vi "myRIO_BRig_RT_v0,77__PortC.vi"() -> ()   [LabVIEW 2014]
uses:
  myRIO_BRig_RT__Case_Exp_stateList.ctl
  myRIO_BRig_RT__Case_NonExp_stateList.ctl
  <vilib>/Platform/TimedLoop/XDataNode/timing_clust.ctl
  <vilib>/Platform/TimedLoop/XDataNode/nitl_modes.ctl
  <vilib>/Platform/TimedLoop/XDataNode/wakeup.ctl
  <vilib>/WebDAVClient/Advanced/SessionHandle.ctl
  <vilib>/myRIO/Common/Instrument Driver Framework/myRIO v1.0/UART/vis/myRIO v1.0 Close UART.vi
  <vilib>/FPGAPlugInAG/myRIO-1900/niLvFpga_Open_myRIO-1900.vi
  <vilib>/rvi/interface/common/dynamic/niFpgaDynamicAddResources.vi
  <vilib>/Utility/error.llb/Error Cluster From Error Code.vi
  <vilib>/rvi/errors/niLvFpgaAdjustHostInterfaceError.vi
  <vilib>/FPGAPlugInAG/Dynamic/niLvFpga_Close_Dynamic.vi
  <vilib>/myRIO/Common/Instrument Driver Framework/Utilities/vis/FPGA Ref Manager.vi
  <vilib>/myRIO/Common/Instrument Driver Framework/myRIO v1.0/myRIO v1.0 Reset FPGA.vi
  <vilib>/myRIO/Common/Instrument Driver Framework/myRIO v1.0/IRQ/vis/myRIO v1.0 IRQ Info FGV.vi
  <vilib>/myRIO/Common/Instrument Driver Framework/myRIO v1.0/IRQ/vis/myRIO v1.0 Timer IRQ Info FGV.vi
  <vilib>/myRIO/Common/Instrument Driver Framework/myRIO v1.0/IRQ/vis/myRIO v1.0 ISR Agent.vi
  <vilib>/rvi/interface/nirviOpenFPGA/nirviOpenFPGA.xnode
  FPGA Bitfiles/myRIOBRig_FPGATarget_myRIOBRigFPGAv3,_Jim92IOu6W4.lvbitx
  myRIO_BRig_FPGA_v3,70__PortC.vi
  <vilib>/rvi/interface/nirviReadWriteControl/nirviReadWriteControl.xnode
  <vilib>/Platform/TimedLoop/XDataNode/XDataNode.xnode
  <vilib>/rvi/interface/nirviCloseFPGA/nirviCloseFPGA.xnode
  <vilib>/Platform/TimedLoop/XDataNode/XDNodeRunTimeDep.lvlib
  <vilib>/rvi/interface/Simulation/niFpgaSimulationCallBeginRW.vi
  <vilib>/myRIO/Instrument Drivers/Utilities/Utilities.lvlib
  <vilib>/WebDAVClient/NI_WebDAV.lvlib
  NiFpgaLv.dll
panel:
  in  "Cue1Param_AudioLed_Count_NS":u16
  in  "Cue1Param_AudioLed_Count_Switch":u16
  in  "Cue1Param_AudioLed_Probability_NS":u16
  in  "Cue1Param_CueType_NS":u16(slide) max=2 step=1 scale=0.0..2.0
  in  "Cue1Param_AudioLed_Probability_Switch":u16
  in  "Cue1Param_CueType_Switch":u16(slide) max=2 step=1 scale=0.0..2.0
  in  "CueLed_Freq":dbl=10.0
  in  "CueLed_Tpeak":dbl=2.0
  in  "CueLed_duration":u16
  in  "Laser_power_step_l2":dbl
  in  "Laser_power_max_l2":dbl
  in  "Laser_power_min_l2":dbl
  in  "Laser_Tshutter_l2":dbl=2.0
  in  "Laser_Freq_l2":dbl=10.0
  in  "Laser_Tpeak_l2":dbl=2.0
  in  "Laser_duration_l2":u16
  in  "LC_Sel_Count_NS_l2":u16
  in  "LC_Sel_Count_Switch_l2":u16
  in  "LC_Sel_Probability_NS_l2":u16
  in  "LC_Sel_Block_NS_l2":u16(slide) max=2 step=1 scale=0.0..2.0
  in  "LC_Sel_OnOff_NS_l2":bool
  in  "LC_Sel_Probability_Switch_l2":u16
  in  "LC_Sel_Block_Switch_l2":u16(slide) max=2 step=1 scale=0.0..2.0
  in  "LC_Sel_OnOff_Switch_l2":bool
  in  "LC_Sel_Tdelay_NS_l2":u16
  in  "LC_Sel_Tdelay_Switch_l2":u16
  in  "LC_Cue1_Count_NS_l2":u16
  in  "LC_Cue1_Count_Switch_l2":u16
  in  "LC_Cue1_delayOpt_NS_l2":bool
  in  "LC_ENL1_delayOpt_NS_l2":bool
  in  "LC_ENL1_Count_NS_l2":u16
  in  "LC_ENL1_Count_Switch_l2":u16
  in  "LC_Cue1_delayOpt_Switch_l2":bool
  in  "LC_ENL1_delayOpt_Switch_l2":bool
  in  "LC_Cue1_Probability_NS_l2":u16
  in  "LC_Cue1_Block_NS_l2":u16(slide) max=2 step=1 scale=0.0..2.0
  in  "LC_Cue1_OnOff_NS_l2":bool
  in  "LC_Cue1_Probability_Switch_l2":u16
  in  "LC_Cue1_Block_Switch_l2":u16(slide) max=2 step=1 scale=0.0..2.0
  in  "LC_Cue1_OnOff_Switch_l2":bool
  in  "LC_ENL1_Probability_NS_l2":u16 max=100 step=1
  in  "LC_ENL1_Block_NS_l2":u16(slide) max=2 step=1 scale=0.0..2.0
  in  "LC_ENL1_OnOff_NS_l2":bool
  in  "LC_ENL1_Probability_Switch_l2":u16 max=100 step=1
  in  "LC_ENL1_Block_Switch_l2":u16(slide) max=2 step=1 scale=0.0..2.0
  in  "LC_Cue1_Tdelay_NS_l2":u16
  in  "LC_ENL1_Tdelay_NS_l2":u16
  in  "LC_Cue1_Tdelay_Switch_l2":u16
  in  "LC_ENL1_Tdelay_Switch_l2":u16
  in  "LC_ENL1_OnOff_Switch_l2":bool
  in  "LC_Wrong_Probability_l2":u16
  in  "LC_Wrong_Trial_l2":u16(slide) max=2 step=1 scale=0.0..2.0
  in  "LC_Wrong_Block_l2":u16(slide) max=2 step=1 scale=0.0..2.0
  in  "LC_Wrong_OnOff_l2":bool
  in  "LC_l2_Reward_Probability":u16
  in  "LC_l2_Reward_Trial":u16(slide) max=2 step=1 scale=0.0..2.0
  in  "LC_l2_Reward_Block":u16(slide) max=2 step=1 scale=0.0..2.0
  in  "LC_l2_Reward_OnOff":bool
  in  "LC_Wrong_Tdelay_l2":u16
  in  "LC_l2_Reward_Tdelay":u16
  in  "LC_Sel_Count_NS_l1":u16
  in  "LC_Sel_Count_Switch_l1":u16
  in  "LC_Sel_Probability_NS_l1":u16
  in  "LC_Sel_Block_NS_l1":u16(slide) max=2 step=1 scale=0.0..2.0
  in  "LC_Sel_OnOff_NS_l1":bool
  in  "LC_Sel_Probability_Switch_l1":u16
  in  "LC_Sel_Block_Switch_l1":u16(slide) max=2 step=1 scale=0.0..2.0
  in  "LC_Sel_OnOff_Switch_l1":bool
  in  "LC_Sel_Tdelay_NS_l1":u16
  in  "LC_Sel_Tdelay_Switch_l1":u16
  out "I_connect_TCP":bool
  out "error out 5":errorcluster
  in  "get_countPerMS":bool
  in  "count_warmup_R_reset":bool
  in  "count_warmup_L_reset":bool
  out "count_warmup_R":u16
  out "count_warmup_L":u16
  out "SolenoidReward":bool
  in  "SolenoidProbability_L":u16=50 caption="Reward Time [ms]" min=1 max=1000 step=1
  in  "SolenoidProbability_R":u16=50 caption="Reward Time [ms]" min=1 max=1000 step=1
  out "output_PortA":dbl caption="LaserPower"
  out "error out 4":errorcluster
  in  "Laser_power_step_l1":dbl
  in  "Laser_power_max_l1":dbl
  in  "Recording":bool
  out "error out 3":errorcluster
  out "error out 2":errorcluster
  in  "Laser_power_min_l1":dbl
  in  "FPGA_count2ms":dbl=159.0
  in  "Laser_Tshutter_l1":dbl=2.0
  in  "Laser_Freq_l1":dbl=10.0
  in  "Laser_Tpeak_l1":dbl=2.0
  in  "Laser_duration_l1":u16
  out "error out":errorcluster
  in  "LC_Cue1_Count_NS_l1":u16
  in  "LC_Cue1_Count_Switch_l1":u16
  in  "LC_Cue1_delayOpt_NS_l1":bool
  in  "LC_ENL1_delayOpt_NS_l1":bool
  in  "LC_ENL1_Count_NS_l1":u16
  in  "LC_ENL1_Count_Switch_l1":u16
  in  "LC_Cue1_delayOpt_Switch_l1":bool
  in  "LC_ENL1_delayOpt_Switch_l1":bool
  in  "Tcycle_Cue_max":u16=1000 caption="Max" min=5 max=5000 step=5
  in  "Tcycle_Cue_min":u16=1000 caption="Min" min=5 max=5000 step=5
  in  "SendData":bool
  out "cSpout":enum16{"Left", "Right"}(ring) caption="Left or Right Spout"
  out "A4":u32 caption="LickCounter_Right"
  out "A2":u32 caption="LickCounter_Left"
  in  "laserResponse_wrong_LED":bool
  out "error_initTrial":errorcluster
  out "error_Selection_pre":errorcluster
  out "error_Selection":errorcluster
  out "SelectWrong":bool
  out "SelectReward":bool
  in  "Left(F)_or_Right(T)":bool
  in  "ignoreWrong":bool
  in  "SelectionState":bool
  in  "laserResponse_wrong":bool
  in  "laserResponse_reward":bool
  in  "laserResponse_reward_LED":bool
  out "nRewards_Right":u16 caption="# Rewards Total (Right)"
  out "nRewards_Left":u16 caption="# Rewards Total (Left)"
  out "nRewards_cur":u16 caption="# Rewards in Current Block"
  out "TpB_target":u16 caption="Target Trials Per Block"
  out "cState_NonExp":T1 caption="WarmUp State"
  out "iBlock":u16 caption="Current Block"
  out "cState":T2 caption="Experimental State"
  out "iTrial":u16 caption="Current Trial"
  in  "warmupType":u8(slide) max=2 step=1 scale=0.0..2.0
  in  "TestConnection":bool
  in  "warmup":bool caption="WarmUp"
  in  "Data Set Prefix":string="Exp1_TM2"
  out "Connected To Host?":bool
  in  "Host Password":string="sabalab"
  in  "Host UserName":string="Test2"
  in  "sp_RightSpout":u16(slide)=2 max=2 step=1 scale=0.0..2.0
  in  "sp_LeftSpout":u16(slide)=2 max=2 step=1 scale=0.0..2.0
  in  "BUR_max":u16 caption="Count Reward Structure  (0 = off)"
  in  "LC_Wrong_Probability_l1":u16
  in  "LC_Wrong_Trial_l1":u16(slide) max=2 step=1 scale=0.0..2.0
  in  "LC_Wrong_Block_l1":u16(slide) max=2 step=1 scale=0.0..2.0
  in  "LC_Wrong_OnOff_l1":bool
  in  "LC_Reward_Probability_l1":u16
  in  "LC_Reward_Trial_l1":u16(slide) max=2 step=1 scale=0.0..2.0
  in  "LC_Reward_Block_l1":u16(slide) max=2 step=1 scale=0.0..2.0
  in  "LC_Reward_OnOff_l1":bool
  in  "LC_Cue1_Probability_NS_l1":u16
  in  "LC_Cue1_Block_NS_l1":u16(slide) max=2 step=1 scale=0.0..2.0
  in  "LC_Cue1_OnOff_NS_l1":bool
  in  "LC_Cue1_Probability_Switch_l1":u16
  in  "LC_Cue1_Block_Switch_l1":u16(slide) max=2 step=1 scale=0.0..2.0
  in  "LC_Cue1_OnOff_Switch_l1":bool
  in  "LC_ENL1_Probability_NS_l1":u16 max=100 step=1
  in  "LC_ENL1_Block_NS_l1":u16(slide) max=2 step=1 scale=0.0..2.0
  in  "LC_ENL1_OnOff_NS_l1":bool
  in  "LC_ENL1_Probability_Switch_l1":u16 max=100 step=1
  in  "LC_ENL1_Block_Switch_l1":u16(slide) max=2 step=1 scale=0.0..2.0
  in  "Tcycle_Timeout":u16=1000 caption="Timeout Time [ms]" min=10 max=10000 step=1
  in  "Tcycle_Wrong":u16=1000 caption="Wrong Time [ms]" min=10 max=10000 step=1
  in  "Tcycle_Selection":u16=1000 caption="Answer Time [ms]" min=1 max=10000 step=1
  in  "Tcycle_RewardPost":u16=1000 caption="Consumption Time [ms]" min=250 max=10000 step=250
  in  "Tcycle_Reward_L":u16=500 caption="Reward Time [ms]" min=1 max=1000 step=1
  in  "Tcycle_Reward_R":u16=500 caption="Reward Time [ms]" min=1 max=1000 step=1
  in  "TpB_Max_R":u16=4 caption="Max TrialsPerBlock" min=1 max=12 step=1
  in  "TpB_Min_R":u16=4 caption="Min TrialsPerBlock" min=1 max=12 step=1
  in  "TpB_Max_L":u16=4 caption="Max TrialsPerBlock" min=1 max=12 step=1
  in  "TpB_Min_L":u16=4 caption="Min TrialsPerBlock" min=1 max=12 step=1
  in  "BUR_min":u16 caption="Count Reward Structure\n(0 = off)"
  in  "TrialUntilReward":bool caption="Ignore Wrong Selection"
  in  "CueCycles":u16=1 caption="Cue Structure" min=1 max=1 step=1
  in  "MTrig_Laser_Tcycle":u16=10 caption="Time [ms]"
  in  "MTrig_Laser_trig":bool
  in  "MTrig_Audio_trig__R":bool caption="Trigger Audio"
  in  "MTrig_Audio_trig__L":bool caption="Trigger Audio"
  in  "RewCalib_Trig_R":bool caption="Calibrate_R"
  in  "RewCalib_Trig_L":bool caption="Calibrate_L"
  in  "MTrig_Solenoid_Tcycle__R":u16=300 caption="Time [ms]"
  in  "MTrig_Solenoid_Tcycle__L":u16=300 caption="Time [ms]"
  in  "MTrig_Solenoid_trig__R":bool caption="Solenoid"
  in  "MTrig_Solenoid_trig__L":bool caption="Solenoid"
  in  "STOP_abort":bool caption="Stop LabView\n(Stops myRio and FPGA)"
  in  "STOP_endBlock":bool caption="Stop Experiment\n@ End of Block"
  in  "STOP_endTrial":bool caption="Stop Experiment\n@ End of Trial"
  in  "START":bool caption="Start Experiment"
  in  "Tcycle_CuePenalty":u16=1000 caption="Penalty" min=1 max=10000 step=1
  in  "Audio_Amp__R":u16=100 caption="Amp"
  in  "Audio_Freq__R":u8=5 caption="Freq [kHz]" max=14 step=1
  in  "Audio_Amp__L":u16=100 caption="Amp"
  in  "Audio_Freq__L":u8=5 caption="Freq [kHz]" max=14 step=1
  in  "LC_Wrong_Tdelay_l1":u16
  in  "LC_Cue1_Tdelay_NS_l1":u16
  in  "LC_ENL1_Tdelay_NS_l1":u16
  in  "LC_Reward_Tdelay_l1":u16
  in  "LC_Cue1_Tdelay_Switch_l1":u16
  in  "LC_ENL1_Tdelay_Switch_l1":u16
  in  "LC_ENL1_OnOff_Switch_l1":bool
  in  "Tcycle_ENLPenalty":u16=100 caption="Penalty" min=10 max=10000 step=10
  in  "Tcycle_ENL_max":u16=1000 caption="Max" min=250 max=10000 step=250
  in  "Tcycle_ENL_min":u16=1000 caption="Min" min=250 max=10000 step=250
  # "Communication (Host PC)"
  # "Recording Rig"
  # "Experimental Run"
  # "Current State"
  # "STOP experiment at"
  # "Global Parameters                                                         Trial Parameters"
  # "Left/Right        Give Reward?        Laser Power [V]"
  # "FPGA Count per [ms]"
  # "Experiment Task Structure"
  # "Timing [ms]"
  # "Block                   Trial            Target Trials       # Rewards \n                                                            Per Block             Current"
  # "Min            Max            Penalty"
  # "(1) = Switching\n(2) = Two Choice"
  # "WarmUp State"
  # "Lick Counter"
  # "Enforced\nNonLick"
  # "WarmUp"
  # "Left           Right"
  # "Cue then reward (no lick)\n \nLeft                    Right"
  # "# Rewards Total\n                                                                  Left                    Right"
  # "Cue"
  # "Experimental State"
  # "Selection\n \n\n \nReward\n    Dispense\n    Time\n \n    Dispense\n    Probability\n \n\n    Consumption\n    Time\n\nWrong Choice\n \n \nTimeout Penalty"
  # "Laser1 Control\n                               On/Off      Block        Probability [%]   Delay [ms]                              Count"
  # "Left                  Right"
  # "Manual Control"
  # "Enforced\nNonLick\n      1"
  # "Min"
  # "Max"
  # "from end"
  # "Solenoid\n \nLeft              Right"
  # "Switch\nTrial"
  # "Speaker\n \nLeft                    Right"
  # "Laser"
  # "from start"
  # "Trial Per Block Structure \n               Left                        Right"
  # "from end"
  # "NonSwitch\nTrials"
  # "from start"
  # "Time\n[ms]"
  # "Time\n[ms]"
  # "Time = Cue Min"
  # "Min"
  # "Cue 1"
  # "Power = Min"
  # "from end"
  # "Switch\nTrial"
  # "Max"
  # "from start"
  # "Cue Audio Parameters"
  # "Laser1 Parameters"
  # "Left                  Right"
  # "from end"
  # "Laser1 Response\n                               On/Off      Block       Trial       Probability [%]   Delay [ms]"
  # "Frequency\n[Hz]"
  # "NonSwitch\nTrials"
  # "Frequency\n[kHz]"
  # "from start"
  # "Timing [ms]\n Duration     Peak Width   Shutter"
  # "Selection Reward"
  # "Selection"
  # "Amp\n(0 - 32,000)"
  # "from start"
  # "Switch\nTrial"
  # "Laser Power [V]\nMin          Max              Step"
  # "Speaker\nPattern\nDuring Cue"
  # "Selection Wrong"
  # "from start"
  # "NonSwitch\nTrials"
  # "Cue LED Parameters"
  # "Laser2 Parameters"
  # "Laser2 Response\n                               On/Off      Block       Trial       Probability [%]   Delay [ms]"
  # "Laser2 Control\n                               On/Off      Block        Probability [%]   Delay [ms]                              Count"
  # "Frequency\n[Hz]"
  # "Frequency\n[Hz]"
  # "Selection Reward"
  # "Enforced\nNonLick\n      1"
  # "from end"
  # "Timing [ms]\n Duration     Peak Width"
  # "Timing [ms]\n Duration     Peak Width   Shutter"
  # "Switch\nTrial"
  # "from start"
  # "Selection Wrong"
  # "from end"
  # "Laser Power [V]\nMin          Max              Step"
  # "NonSwitch\nTrials"
  # "from start"
  # "Cue 1"
  # "from end"
  # "Switch\nTrial"
  # "from start"
  # "Cue1 Control\n                                         Cue Type                     Audio or LED       LED Probability [%]      Count"
  # "from end"
  # "NonSwitch\nTrials"
  # "Cue 1"
  # "from start"
  # "Switch\nTrial"
  # "Selection"
  # "from start"
  # "Switch\nTrial"
  # "NonSwitch\nTrials"
  # "from start"
  # "NonSwitch\nTrials"
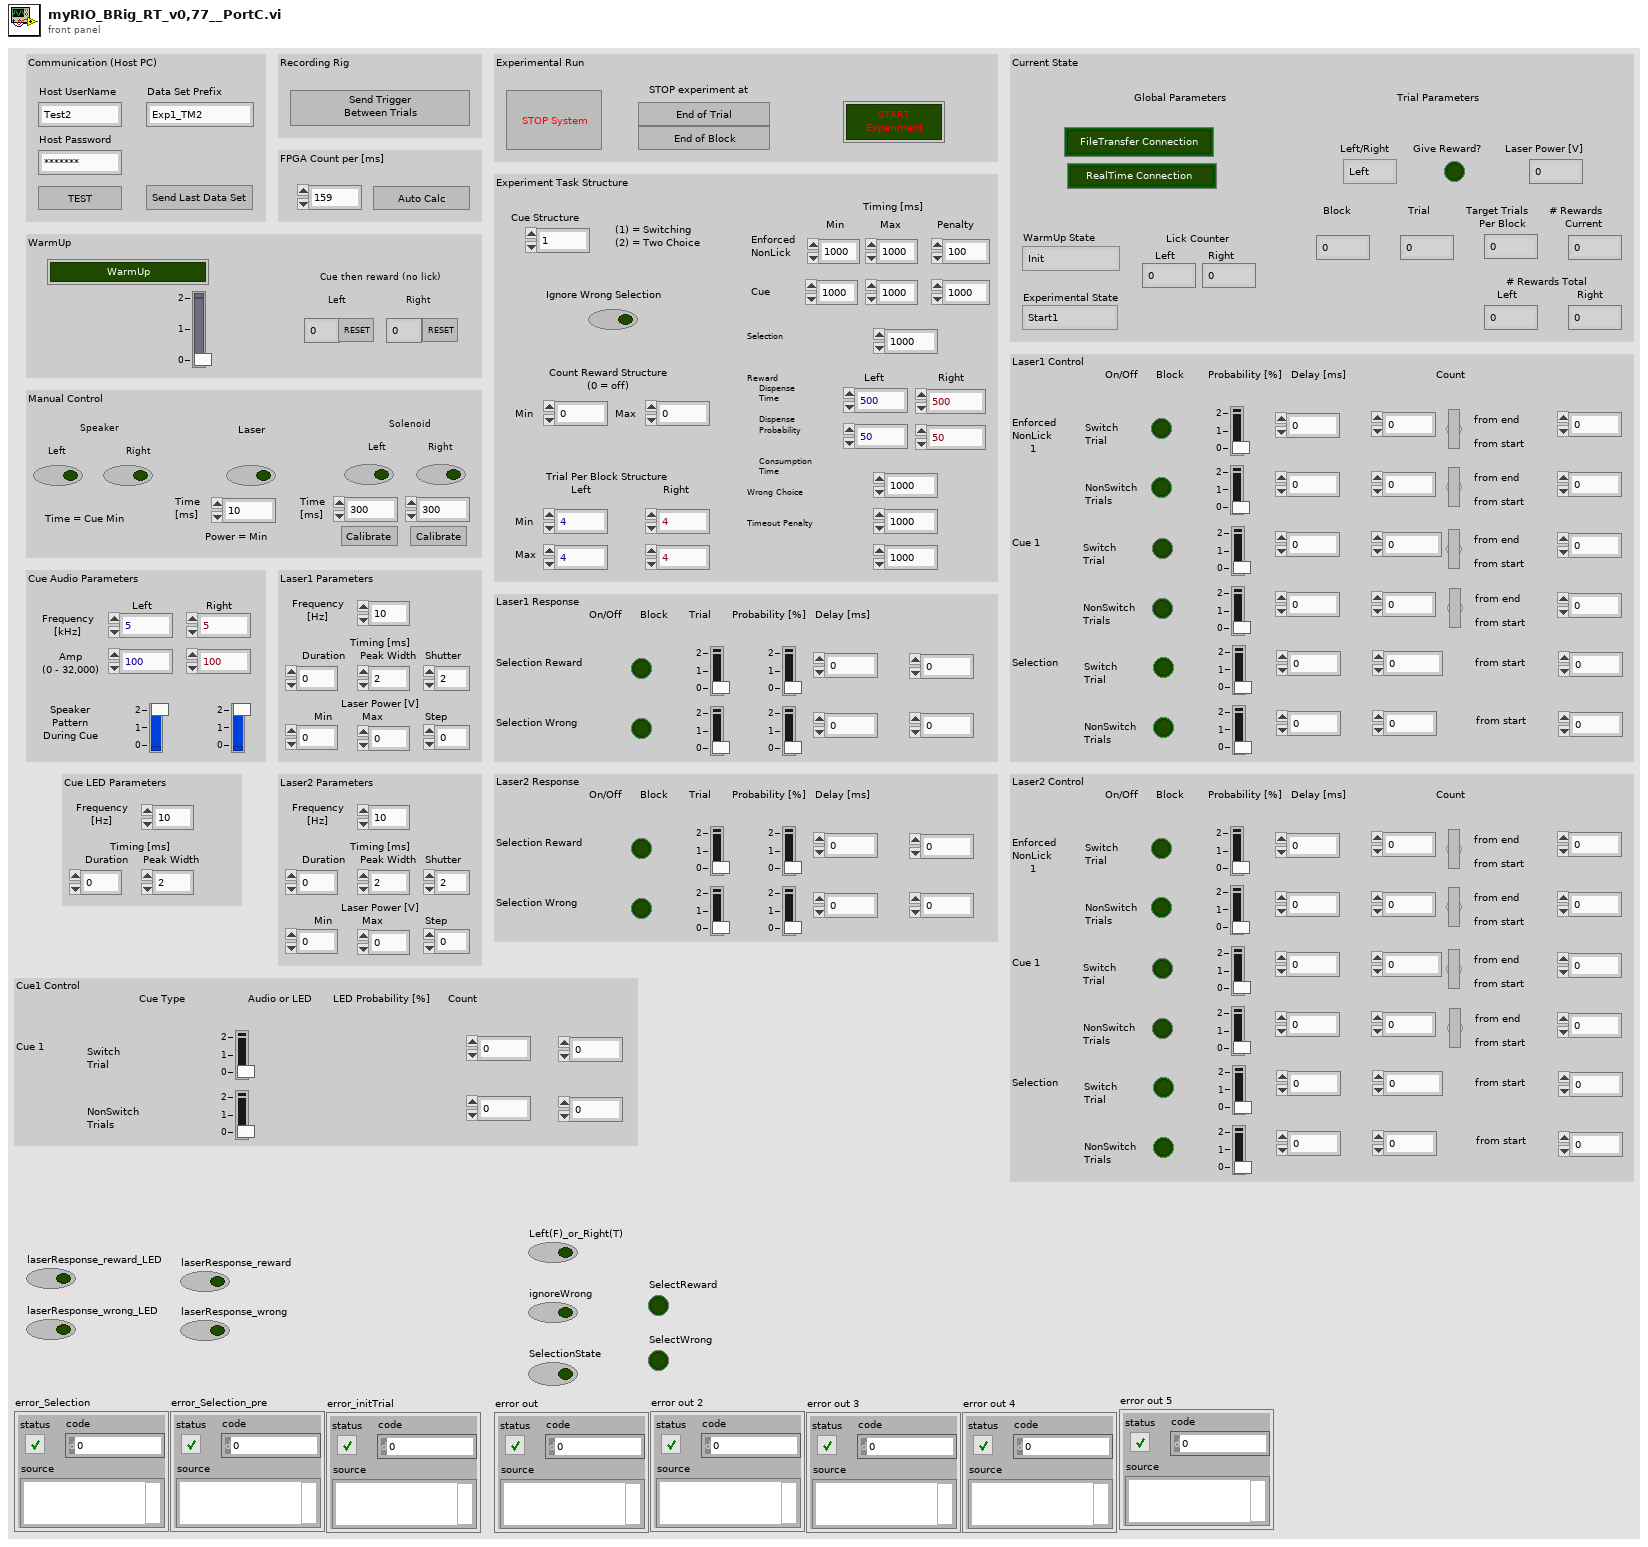
[diagram p1: front panel]
types:
  T1 = typedef "myRIO_BRig_RT__Case_NonExp_stateList.ctl" = enum16{"Init", "UploadSettings_pre", "UploadSettings_Read_dataExp", "UploadSettings_dataExp_1", "UploadSettings_dataExp_2", "UploadSettings_Read_dataLC", "UploadSettings_dataLC_1", "UploadSettings_dataLC_2", "UploadSettings_dataLC_3", "UploadSettings_dataLC_4", "UploadSettings_Read_dataMTrig", "UploadSettings_dataMTrig_1", "UploadSettings_post", "Idle_pre", "IdleEmpty", "IdleEmpty2", "IdleEmpty3", "IdleEmpty4", "Idle", "Idle_2", "Idle_3", "Idle_4", "Idle_5", "Idle_6", "Idle_post", "Cue_pre__pre", "Cue_pre", "Cue", "Cue_LED", "Cue_post", "RewardCalibration_pre", "DispenseWater_pre__pre", "DispenseWater_pre", "DispenseWater", "DispenseWater_post", "TestConnection", "SendData", "Get_FPGA_count_per_ms", "End"}
  T2 = typedef "myRIO_BRig_RT__Case_Exp_stateList.ctl" = enum16{"Start1", "Start2", "Start3", "saveSettings1", "saveSettings2", "saveSettings3", "saveSettings4", "saveSettings_LC_ENL_l1", "saveSettings_LC_ENL_l2", "saveSettings_LC_Cue_l1", "saveSettings_LC_Cue_l2", "saveSettings6_LC_l1_Other", "SaveSettings6_LC_l2_Other", "setSettings_Audio", "setSettings_Laser", "initBlock_pre", "initBlock", "initBlock2", "initBlock_post", "initTrial_pre", "initTrial", "initTrial2", "initTrial3", "initTrial4", "initTrial_LC_ENL1", "initTrial_LC_Cue1", "initTrial_LC_Cue1_2", "initTrial_LC_Sel", "initTrial_post", "ENL1_pre", "ENL1", "ENL1_post", "ENL1Penalty_pre", "ENL1Penalty", "ENL2_pre", "ENL2", "ENL2Penalty_pre", "ENL2Penalty", "Cue1_pre", "Cue1", "Cue1_post", "Cue1Penalty_pre", "Cue1Penalty", "Cue2_pre", "Cue2", "Cue2Penalty_pre", "Cue2Penalty", "Selection_pre", "Selection", "Select_post", "SelectReward_pre", "SelectReward", "SelectRewardPost_pre", "SelectRewardPost", "SelectWrong_pre", "SelectWrong", "SelectWrong_post", "SelectTimeout_pre", "SelectTimeout", "SelectTimeout_post", "endTrial_pre", "endTrial1", "endTrial2", "endTrial3", "endTrial_post", "endBlock_pre", "endBlock", "endBlock_post", "endExp", "commConnect", "commUpload_pre", "commUpload_dataBlock", "commUpload_dataCurrent", "commUpload_dataExp", "commUpload_dataLC", "commUpload_dataTrial", "commUpload_post", "saveData_pre", "saveData_dataBlock", "saveData_dataCurrent", "saveData_dataExp", "saveData_dataLC", "saveData_dataTrial", "saveData_post", "empty_endBlock1", "empty_endBlock2", "empty_endTrial1", "empty_endTrial2", "empty_endTrial3", "empty_endTrial4", "empty_endTrial5", "dummyState", "dummyState_endBlock"}
  T3 = typedef "XDNodeRunTimeDep.lvlib/timing_clust.ctl" = cluster{"Expected End [f-1]":u64, "Actual End [f-1]":u64, "Finished Late? [f-1]":bool, "Expected End [i-1]":u64, "Actual End [i-1]":u64, "Finished Late? [i-1]":bool, "Expected Start [i]":u64, "Actual Start [i]":u64, "Expected Start [f]":u64, "Actual Start [f]":u64, "Source Name":string, "Structure Name":string, "Period":i64, "Deadline":i64, "Offset":i64, "Start":i64, "Priority":i32, "Timeout":i32, "Mode":T4, "Wakeup Reason":T5, "Error":errorcluster, "Source Type":string, "Secondary Source Type":string, "Global End Time":u64, "Global Start Time":u64, "Frame Duration":u64, "Iteration Duration":u64, "Assigned CPU":i32, "I/O Scan Engine Mode":u32}
  T4 = typedef "XDNodeRunTimeDep.lvlib/nitl_modes.ctl" = enum32{"No Change", "Process missed periods, maintain original phase", "Discard missed periods, maintain original phase", "Process missed periods, ignore original phase", "Discard missed periods, ignore original phase"}
  T5 = typedef "XDNodeRunTimeDep.lvlib/wakeup.ctl" = enum32{"Normal", "Aborted", "Asynchronous wakeup", "Timing source error", "Timed loop error", "Timeout"}
  T6 = typedef "NI_WebDAV.lvlib/SessionHandle.ctl" = refnum<k1>
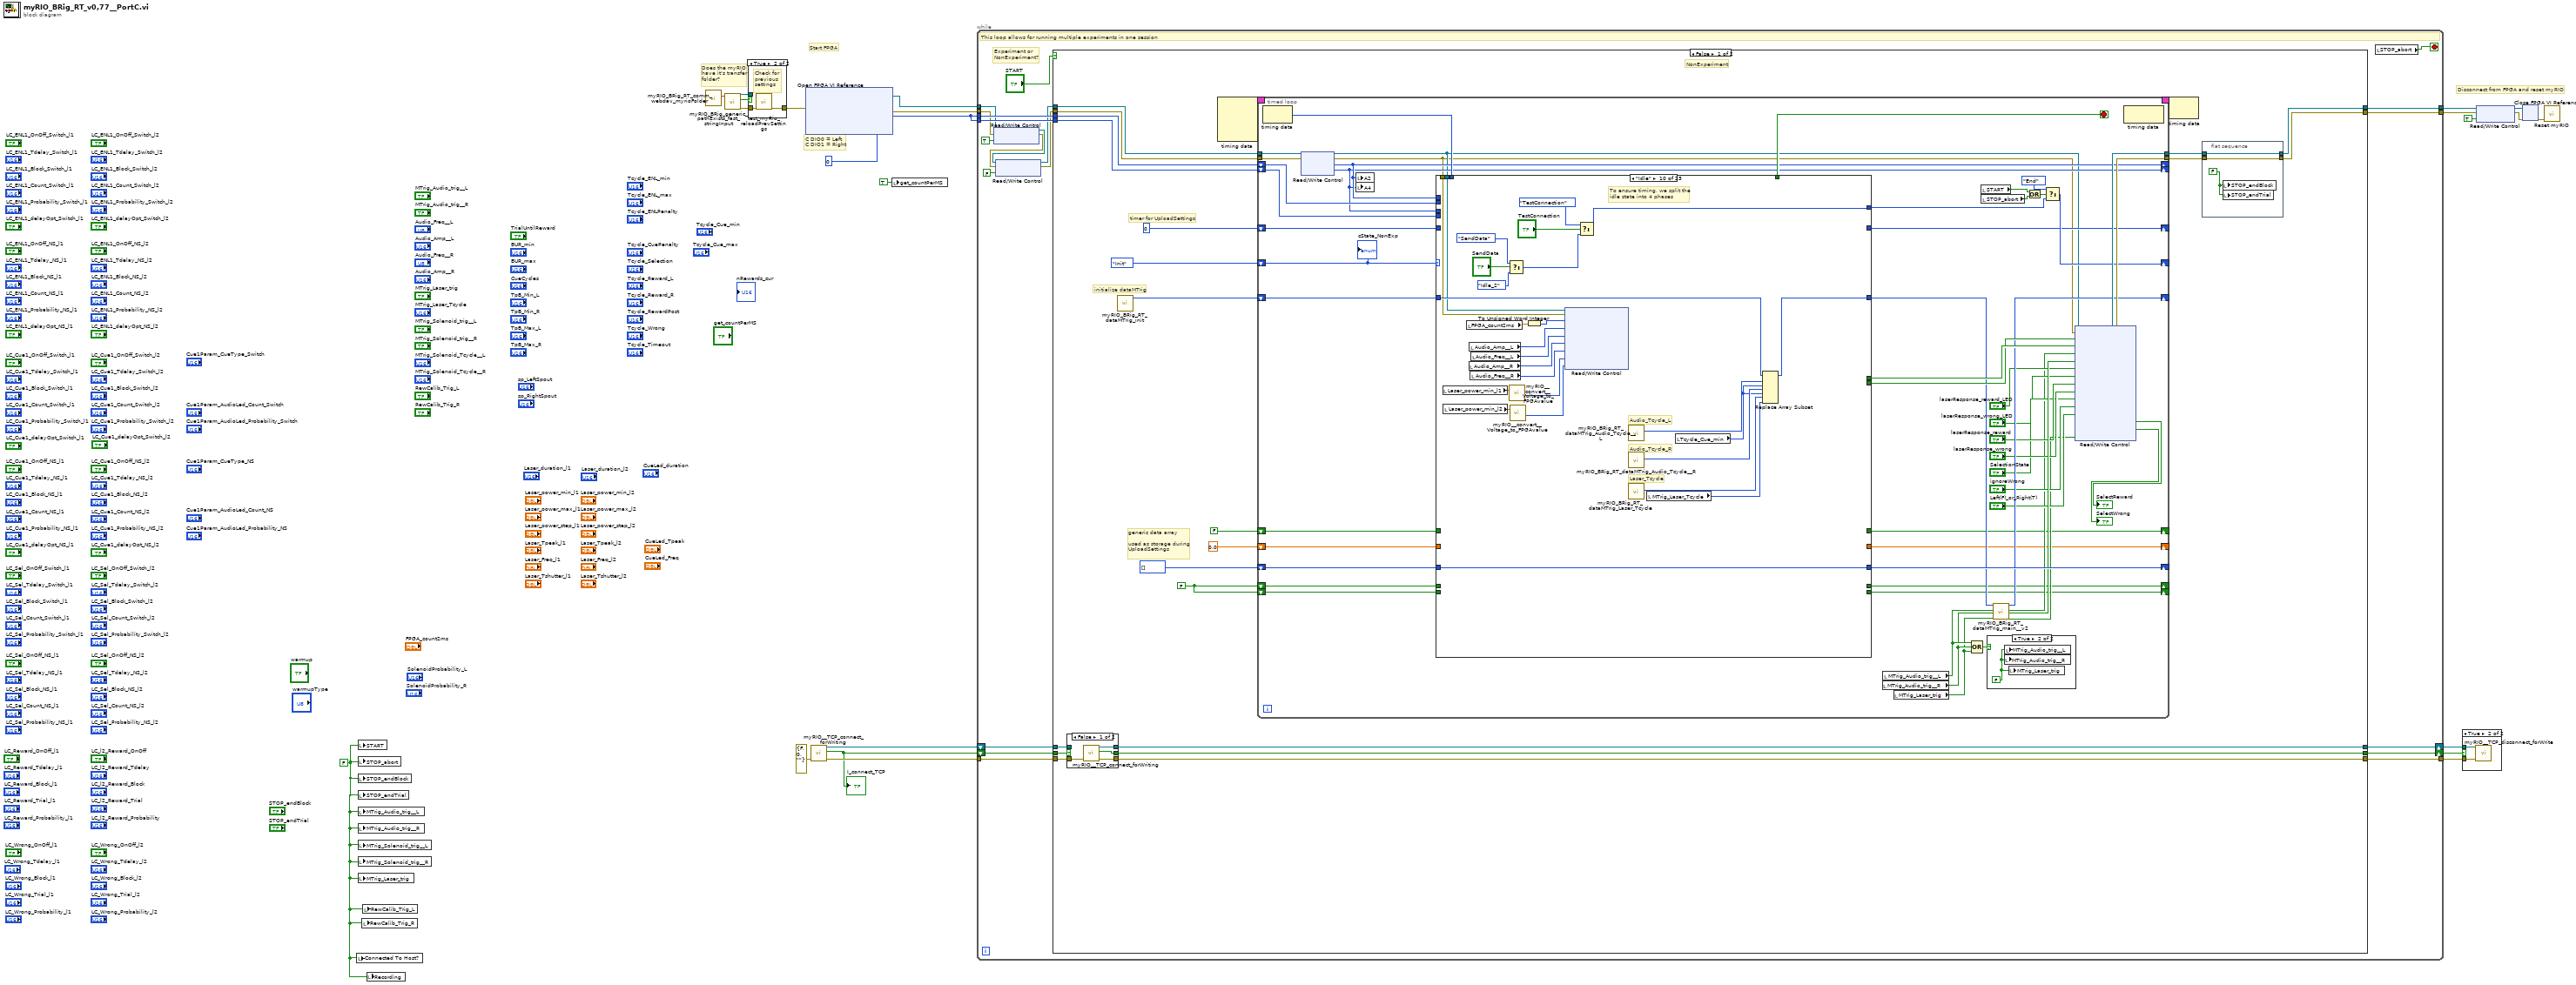
[diagram p0: block diagram]
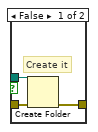
[diagram p3: hidden frame]
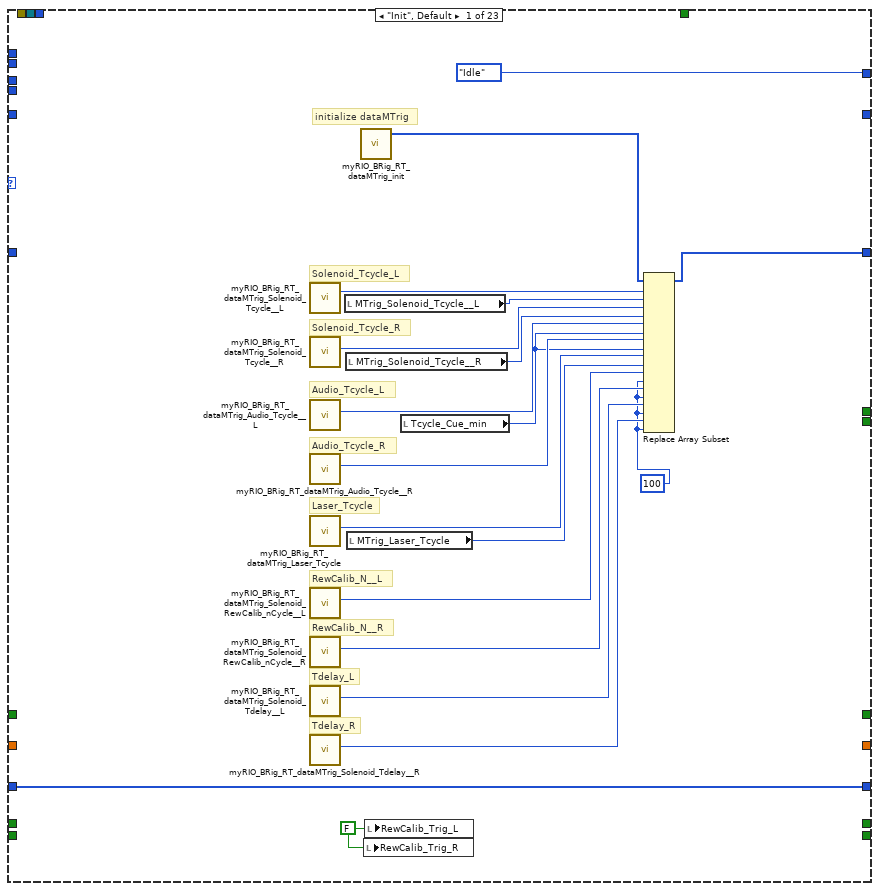
[diagram p6: hidden frame]
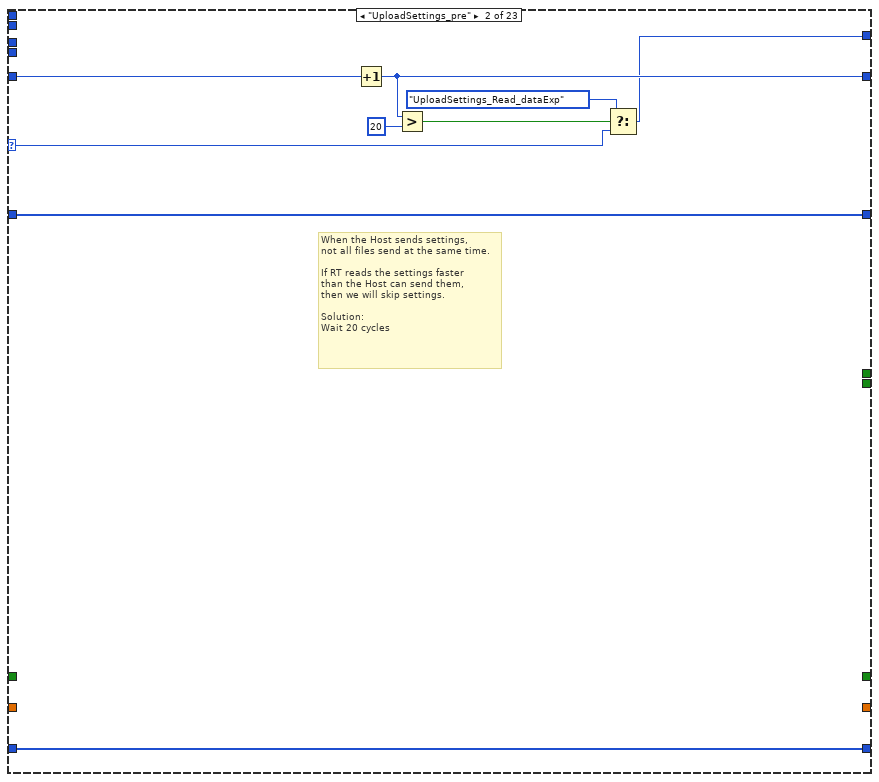
[diagram p7: hidden frame]
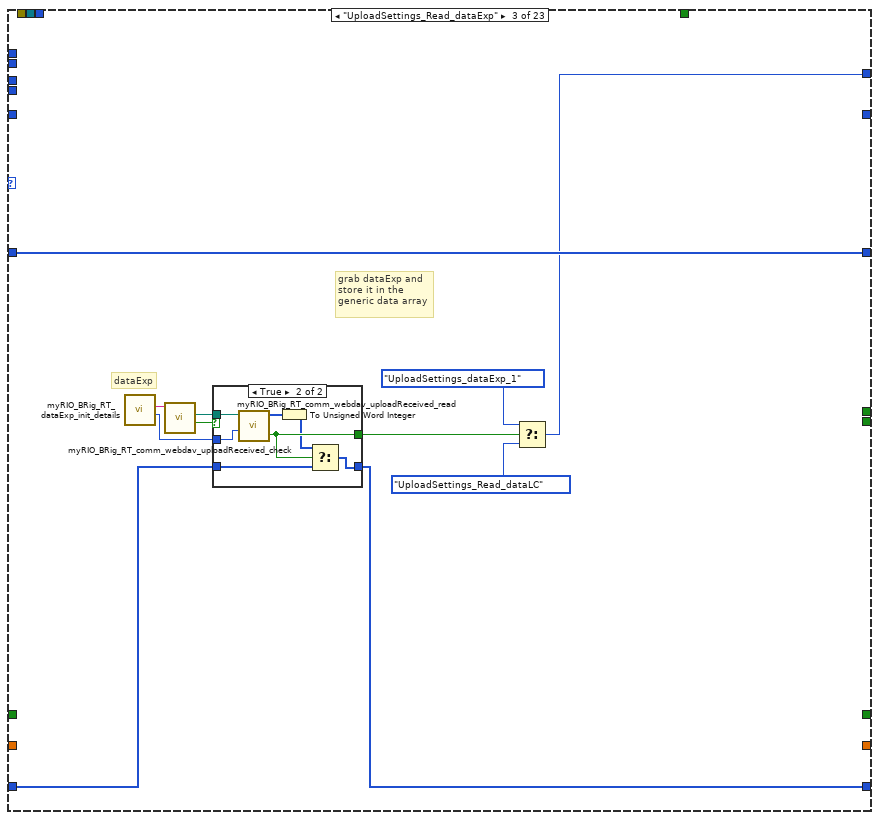
[diagram p8: hidden frame]
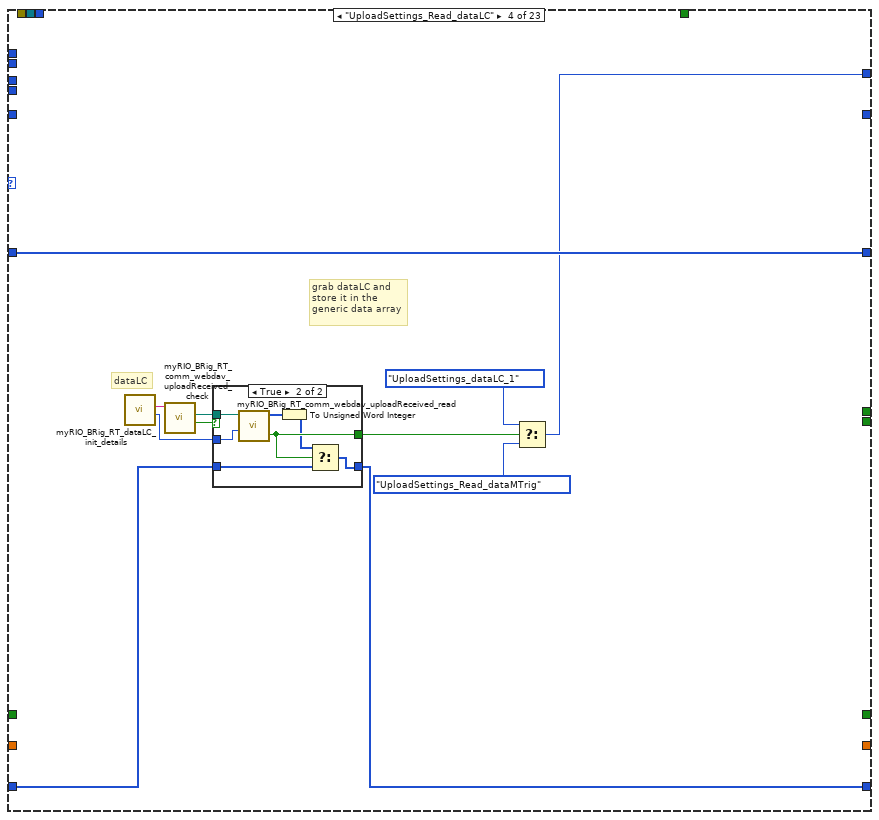
[diagram p10: hidden frame]
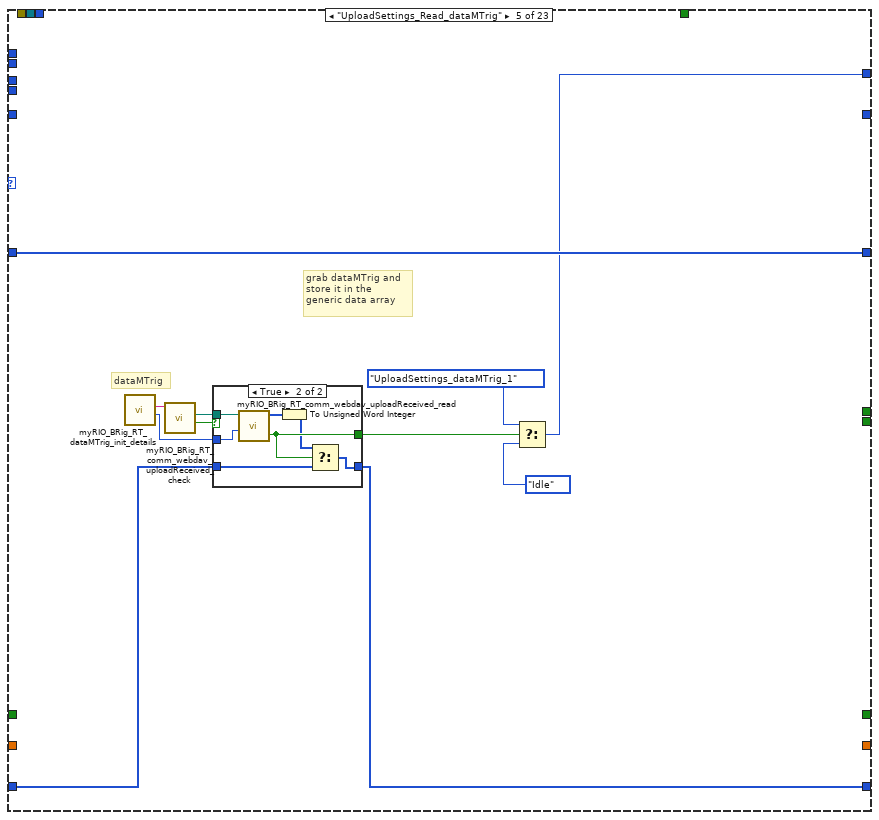
[diagram p12: hidden frame]
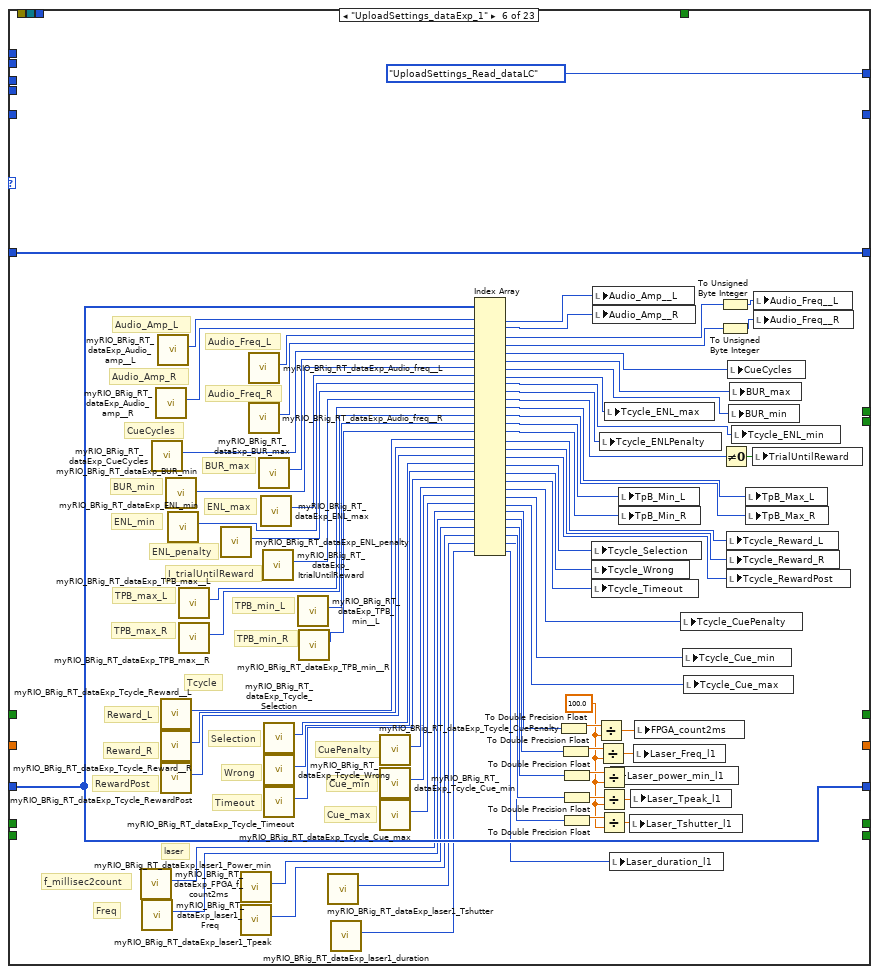
[diagram p14: hidden frame]
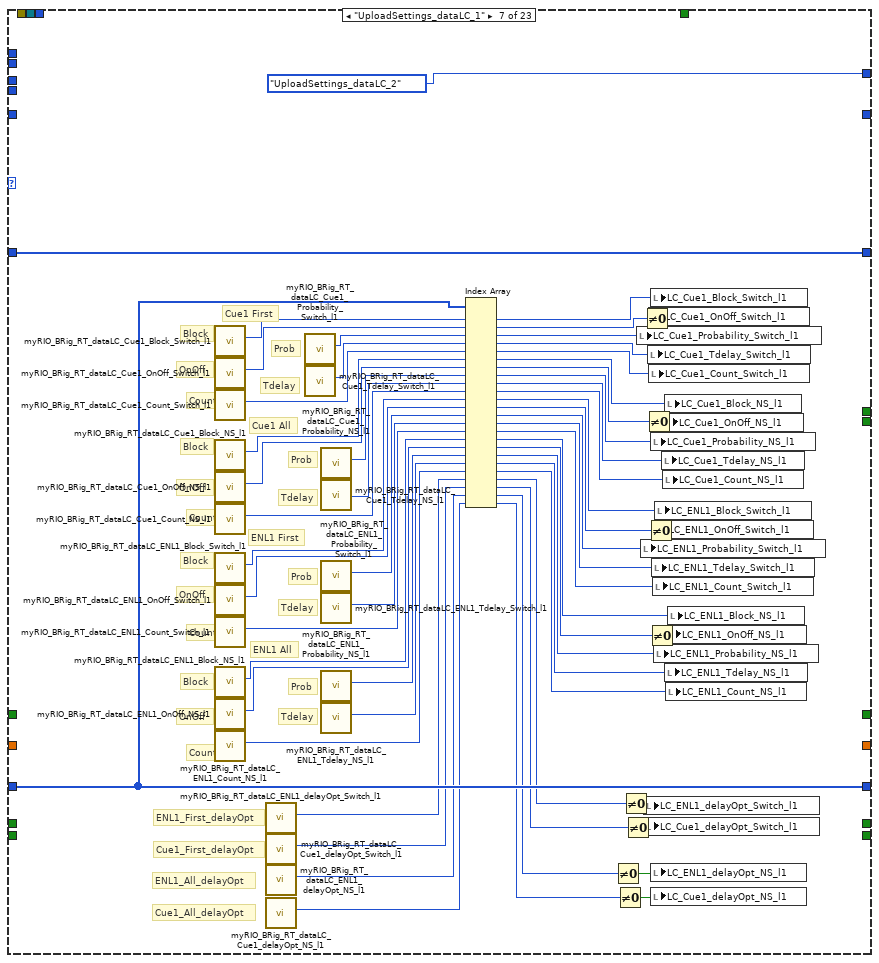
[diagram p15: hidden frame]
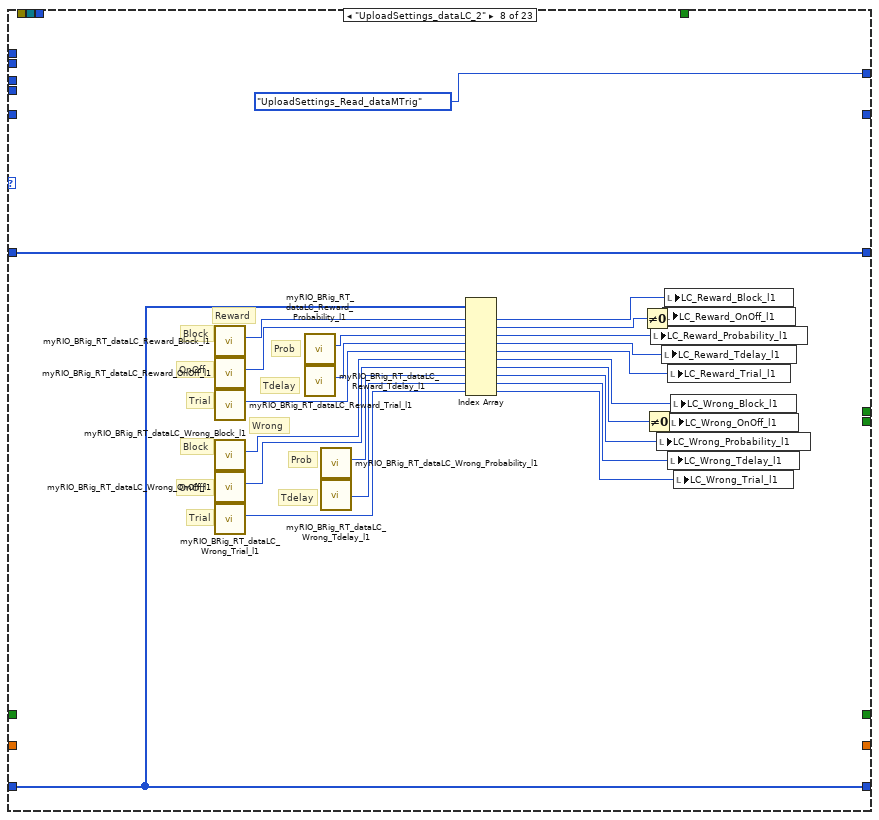
[diagram p16: hidden frame]
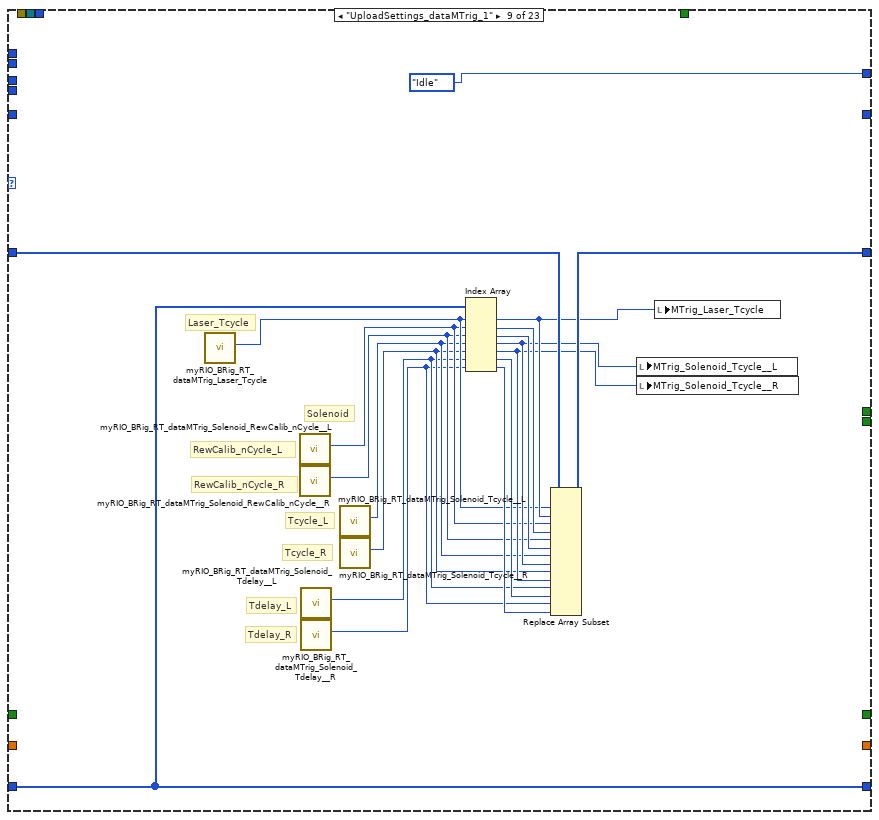
[diagram p17: hidden frame]
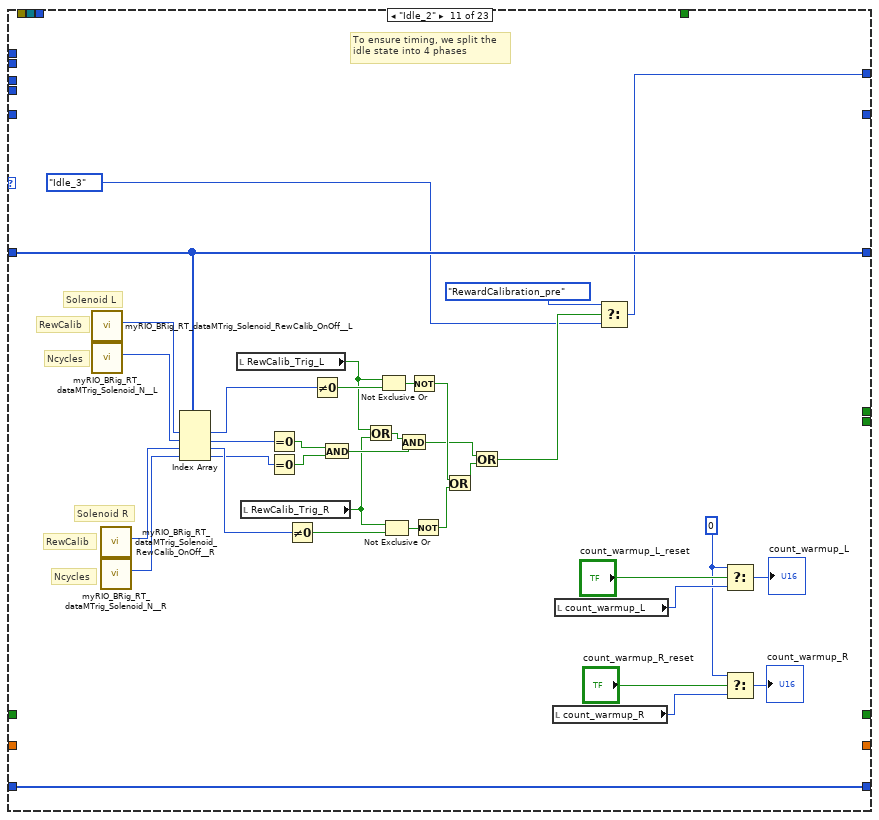
[diagram p18: hidden frame]
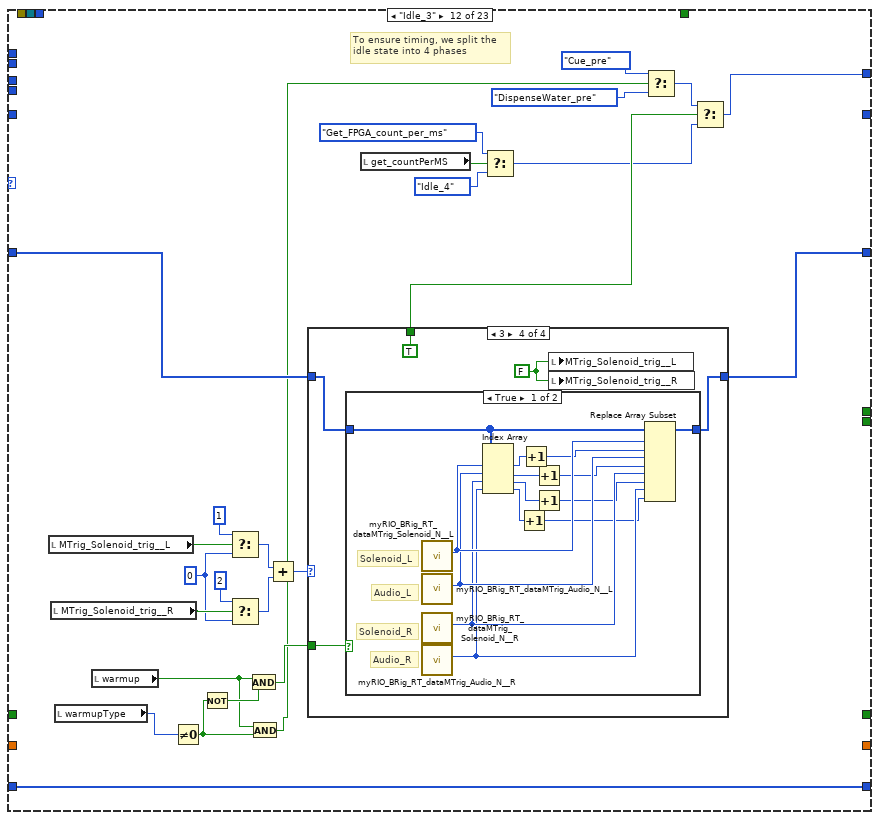
[diagram p19: hidden frame]
diagram:
  w17 = u32 0
  w1 = FALSE
  # "Does the myRIO\nhave it's transfer\nfolder?"
  # "C DIO0 = Left\nC DIO1 = Right"
  # "Start FPGA"
  # "Disconnect from FPGA and reset myRIO"
  n1 = local write "Connected To Host?"(w1) -> ()
  n2 = local write "START"(w1) -> ()
  n3 = local write "STOP_abort"(w1) -> ()
  n4 = local write "STOP_endBlock"(w1) -> ()
  n5 = local write "STOP_endTrial"(w1) -> ()
  n6 = local write "MTrig_Audio_trig__L"(w1) -> ()
  n7 = local write "MTrig_Audio_trig__R"(w1) -> ()
  n8 = local write "MTrig_Solenoid_trig__L"(w1) -> ()
  n9 = local write "MTrig_Solenoid_trig__R"(w1) -> ()
  n10 = local write "MTrig_Laser_trig"(w1) -> ()
  n11 = local write "RewCalib_Trig_R"(w1) -> ()
  n12 = local write "RewCalib_Trig_L"(w1) -> ()
  n13 = local write "Recording"(w1) -> ()
  n14 = call "myRIO_BRig_RT_comm_webdav_myrioFolder.vi"() -> ("output_myrioFolder"=w14:string)  [unwired: 11 in]
  n15 = call "myRIO_BRig_generic_pathExists_fast_stringInput.vi"("input_filePath"=w14) -> ("output_error"=w13:errorcluster, "output_Iexist"=w12:bool, "output_filePath"=w11:path)  [unwired: 8 in]
  n16 = case shown="True" w12 {
    tunnel: w11 -> [w26 _]
    tunnel: w13 -> [w25 w28]
    tunnel: [w24 w27] -> w9
    frame False {
      # "Create it"
      n17 = Create Folder(path (use dialog)=w26, error in=w25) -> (error out=w24:errorcluster)  [unwired: 1 in, 2 out]
    }
    frame True {
      # "Check for\nprevious\nsettings"
      n18 = call "test_myRio_reloadPrevSettings.vi"("input_error"=w28) -> ("output_error"=w27:errorcluster)  [unwired: 10 in]
    }
  }
  n19 = xnode "Open FPGA VI Reference"("error in"=w9) -> ("FPGA VI Reference Out"=w19:refnum<k20>, "error out"=w18:errorcluster)  [unwired: 1 in]
  n20 = call "myRIO__TCP_connect_forWriting.vi"("input_error"=errorcluster {"status"=FALSE, "code"=0, "source"=""}) -> ("output_error"=w7:errorcluster, "output_connected"=w6:bool, "output_hTCP"=w10:refnum<k5>)  [unwired: 8 in]
  "I_connect_TCP" <- w6
  n21 = local write "get_countPerMS"(TRUE ("get_countPerMS")) -> ()
  n22 = while {
    tunnel: w19 -> [w38]
    tunnel: w18 -> [w43]
    tunnel: w17 -> [w46]
    tunnel: w17 -> [w45]
    tunnel: [w36] -> w16
    tunnel: [w35] -> w15
    shift-right: [w32] -> w5
    shift-left: w6 -> [w33]
    tunnel: w7 -> [w31]
    shift-right: [w30] -> w4
    shift-left: w10 -> [w34]
    tunnel: [w29] -> w3
    stop <- w44 stop-if-true
    # "Experiment or\nNonExperiment?"
    # "This loop allows for running multiple experiments in one session"
    n23 = xnode "Read/Write Control"("FPGA VI Reference In"=w38, "error in"=w43, "Counts_Reset"=TRUE) -> ("FPGA VI Reference Out"=w40:refnum<k20>, "error out"=w41:errorcluster)
    n24 = xnode "Read/Write Control"("FPGA VI Reference In"=w40, "error in"=w41, "Counts_Reset"=FALSE) -> ("FPGA VI Reference Out"=w37:refnum<k20>, "error out"=w39:errorcluster)
    n25 = case shown="False" "START" {
      tunnel: w46 -> [w67 w989]
      tunnel: w45 -> [w66 w988]
      tunnel: w39 -> [w64 w919]
      tunnel: w37 -> [w65 w920]
      tunnel: [w62 w985] -> w36
      tunnel: [w60 w980] -> w35
      tunnel: w34 -> [w53 w931]
      tunnel: [w51 w935] -> w30
      tunnel: w33 -> [w52 w933]
      tunnel: [w50 w934] -> w32
      tunnel: w31 -> [w54 w932]
      tunnel: [w49 w930] -> w29
      frame False {
        w57 = FALSE
        # "generic data array\n\nused as storage during\nUploadSettings"
        # "timer for UploadSettings"
        # "initialize dataMTrig"
        # "NonExperiment"
        n26 = case shown="False" w52 {
          selector: w52 -> [_ w76]
          tunnel: w54 -> [w73 w78]
          tunnel: [w74 w78] -> w49
          tunnel: w53 -> [_ w77]
          tunnel: [w75 w77] -> w51
          tunnel: [w72 w76] -> w50
          frame False {
            n27 = call "myRIO__TCP_connect_forWriting.vi"("input_error"=w73) -> ("output_error"=w74:errorcluster, "output_connected"=w72:bool, "output_hTCP"=w75:refnum<k5>)  [unwired: 8 in]
          }
          frame True {
          }
        }
        n28 = call "myRIO_BRig_RT_dataMTrig_init.vi"() -> ("output_dataMTrig"=w68:u16[])  [unwired: 5 in]
        n29 = node-c288() -> (w71:T3)  [unwired: 4 in]
        n30 = timed-loop {
          timing: w71 -> [_]
          timing-out: [_] -> w70
          shift-right: [w120] -> _
          shift-left: w68 -> [w132]
          shift-right: [w114] -> _
          shift-left: myRIO_BRig_RT__Case_NonExp_stateList."Init" ("Enum") -> [w126]
          shift-right: [w98] -> _
          shift-left: w67 -> [w99]
          shift-right: [w96] -> _
          shift-left: w66 -> [w97]
          tunnel: [w128] -> w63
          tunnel: [w127] -> w61
          tunnel: w64 -> [w130]
          tunnel: w65 -> [w129]
          shift-right: [w125] -> _
          shift-left: u16[] [] ("output_data") -> [w124]
          shift-right: [w100] -> _
          shift-left: u16 0 ("Audio_Amp__L") -> [w101]
          shift-right: [w93] -> _
          shift-left: w57 -> [w95]
          shift-right: [w92] -> _
          shift-left: w57 -> [w94]
          shift-right: [w88] -> _
          shift-left: FALSE -> [w89]
          shift-right: [w86] -> _
          shift-left: 0.0 -> [w87]
          stop <- w133 stop-if-true
          n31 = node-c288() -> (w131:i64)  [unwired: 1 in]
          n32 = xnode "Read/Write Control"("FPGA VI Reference In"=w129, "error in"=w130) -> ("FPGA VI Reference Out"=w91:refnum<k20>, "error out"=w90:errorcluster, "A2_LickL"=w98:u32, "A4_LickR"=w96:u32)
          n33 = local write "A2"(w98) -> ()
          n34 = local write "A4"(w96) -> ()
          n35 = case shown="\"Idle\"" w126 {
            selector: w126 -> [_ w158 _ _ _ _ _ _ _ _ _ _ _ _ w586 _ _ w794 _ _ _ w869 w913]
            tunnel: [myRIO_BRig_RT__Case_NonExp_stateList."Idle" ("Enum") w156 w163 w182 w201 myRIO_BRig_RT__Case_NonExp_stateList."UploadSettings_Read_dataLC" ("Enum") myRIO_BRig_RT__Case_NonExp_stateList."UploadSettings_dataLC_2" ("Enum") myRIO_BRig_RT__Case_NonExp_stateList."UploadSettings_Read_dataMTrig" ("f") myRIO_BRig_RT__Case_NonExp_stateList."Idle" ("Enum") w418 w434 w473 w554 myRIO_BRig_RT__Case_NonExp_stateList."Cue" ("t") w581 myRIO_BRig_RT__Case_NonExp_stateList."DispenseWater_pre" ("Enum") w739 w792 w815 myRIO_BRig_RT__Case_NonExp_stateList."Idle" ("Enum") myRIO_BRig_RT__Case_NonExp_stateList."Idle" ("Enum") w868 w913] -> w115
            tunnel: [w145 w155 w173 w192 w211 w296 w355 w380 w396 w422 w449 w478 w552 w570 w587 w649 w776 w799 w826 w861 w867 w880 w911] -> w121
            tunnel: [_ _ _ _ _ _ _ _ _ _ _ _ _ _ _ _ _ _ _ _ _ _ TRUE] -> w133
            tunnel: w132 -> [_ w155 w173 w192 w211 w296 w355 w380 w397 w421 w449 w479 w552 w571 w588 w635 w772 w800 w827 w861 w867 w880 w911]
            tunnel: w131 -> [_ _ _ _ _ _ _ _ _ _ _ _ _ _ _ _ _ w804 _ _ _ _ _]
            tunnel: [w138 w154 w164 w183 w202 w245 w311 w356 w381 w417 w433 w467 w551 w560 w595 w630 w724 w777 w808 w853 w865 w879 w910] -> w125
            tunnel: w124 -> [w138 w154 w165 w184 w203 w245 w311 w356 w381 w417 w433 w467 w551 w560 w595 w630 w724 w777 w808 w853 w865 w879 w910]
            tunnel: [_ _ _ _ _ _ _ _ _ _ _ _ _ _ _ _ _ w801 _ _ _ _ _] -> w123
            tunnel: [_ _ _ _ _ _ _ _ _ _ _ _ _ _ _ _ _ w783 _ _ _ _ _] -> w122
            tunnel: w101 -> [_ w162 _ _ _ _ _ _ _ _ _ _ _ _ _ _ _ _ _ _ _ _ _]
            tunnel: [_ w161 _ _ _ _ _ _ _ _ _ _ _ _ _ _ _ _ _ _ _ _ _] -> w100
            tunnel: w99 -> [_ _ _ _ _ _ _ _ _ _ _ _ _ _ w592 _ _ _ _ _ _ _ _]
            tunnel: w98 -> [_ _ _ _ _ _ _ _ _ _ _ _ _ _ w593 _ _ _ _ _ _ _ _]
            tunnel: w97 -> [_ _ _ _ _ _ _ _ _ _ _ _ _ _ w590 _ _ _ _ _ _ _ _]
            tunnel: w96 -> [_ _ _ _ _ _ _ _ _ _ _ _ _ _ w591 _ _ _ _ _ _ _ _]
            tunnel: w95 -> [_ _ _ _ _ _ _ _ _ _ _ _ _ _ w578 _ _ _ _ _ _ _ _]
            tunnel: w94 -> [_ _ _ _ _ _ _ _ _ _ _ _ _ _ w577 _ _ _ _ _ _ _ _]
            tunnel: [_ _ _ _ _ _ _ _ _ _ _ _ _ w559 w578 _ _ _ _ _ _ _ _] -> w93
            tunnel: [_ _ _ _ _ _ _ _ _ _ _ _ _ w558 w577 _ _ _ _ _ _ _ _] -> w92
            tunnel: w91 -> [_ _ _ _ _ _ _ _ _ w408 _ _ _ _ _ _ _ _ _ _ _ w874 _]
            tunnel: w90 -> [_ _ _ _ _ _ _ _ _ w407 _ _ _ _ _ _ _ _ _ _ _ w873 _]
            tunnel: w89 -> [_ _ _ _ _ _ _ _ _ _ _ _ _ _ _ _ _ _ _ _ _ w878 _]
            tunnel: [_ _ _ _ _ _ _ _ _ _ _ _ _ _ _ _ _ _ _ _ _ TRUE _] -> w88
            tunnel: w87 -> [_ _ _ _ _ _ _ _ _ _ _ _ _ _ _ _ _ _ _ _ _ w876 _]
            tunnel: [_ _ _ _ _ _ _ _ _ _ _ _ _ _ _ _ _ _ _ _ _ w875 _] -> w86
            frame "Init", Default {
              w139 = FALSE ("RewCalib_Trig_L")
              w135 = u16 100 ("new element/subarray")
              # "Tdelay_R"
              # "Tdelay_L"
              # "RewCalib_N__R"
              # "RewCalib_N__L"
              # "Solenoid_Tcycle_R"
              # "Solenoid_Tcycle_L"
              # "Laser_Tcycle"
              # "Audio_Tcycle_R"
              # "Audio_Tcycle_L"
              # "initialize dataMTrig"
              n36 = call "myRIO_BRig_RT_dataMTrig_Solenoid_Tcycle__L.vi"() -> ("output_Solenoid_Tcycle__L"=w147:i32)  [unwired: 11 in]
              n37 = call "myRIO_BRig_RT_dataMTrig_Solenoid_Tcycle__R.vi"() -> ("output_Solenoid_Tcycle__R"=w148:i32)  [unwired: 11 in]
              n38 = call "myRIO_BRig_RT_dataMTrig_Audio_Tcycle__L.vi"() -> ("output_Audio_Tcycle__L"=w149:i32)  [unwired: 11 in]
              n39 = call "myRIO_BRig_RT_dataMTrig_Audio_Tcycle__R.vi"() -> ("output_Audio_Tcycle__R"=w150:i32)  [unwired: 11 in]
              n40 = call "myRIO_BRig_RT_dataMTrig_Laser_Tcycle.vi"() -> ("output_Laser_Tcycle"=w151:i32)  [unwired: 11 in]
              n41 = call "myRIO_BRig_RT_dataMTrig_Solenoid_RewCalib_nCycle__L.vi"() -> ("output_Solenoid_RewCalib_nCycle__L"=w143:i32)  [unwired: 11 in]
              n42 = call "myRIO_BRig_RT_dataMTrig_Solenoid_RewCalib_nCycle__R.vi"() -> ("output_Solenoid_RewCalib_nCycle__R"=w142:i32)  [unwired: 11 in]
              n43 = call "myRIO_BRig_RT_dataMTrig_Solenoid_Tdelay__L.vi"() -> ("output_Solenoid_Tdelay__L"=w141:i32)  [unwired: 11 in]
              n44 = call "myRIO_BRig_RT_dataMTrig_Solenoid_Tdelay__R.vi"() -> ("output_Solenoid_Tdelay__R"=w140:i32)  [unwired: 11 in]
              n45 = local read "MTrig_Solenoid_Tcycle__L"() -> (w152:u16)
              n46 = local read "MTrig_Solenoid_Tcycle__R"() -> (w153:u16)
              n47 = local read "MTrig_Laser_Tcycle"() -> (w136:u16)
              n48 = call "myRIO_BRig_RT_dataMTrig_init.vi"() -> ("output_dataMTrig"=w146:u16[])  [unwired: 5 in]
              n49 = local write "RewCalib_Trig_R"(w139) -> ()
              n50 = local write "RewCalib_Trig_L"(w139) -> ()
              n51 = local read "Tcycle_Cue_min"() -> (w137:u16)
              n52 = Replace Array Subset(array=w146, new element #1=w152, index #1=w147, new element #2=w153, index #2=w148, new element #3=w137, index #3=w149, new element #4=w137, index #4=w150, new element #5=w136, index #5=w151, new element #6=w135, index #6=w143, new element #7=w135, index #7=w142, new element #8=w135, index #8=w141, new element #9=w135, index #9=w140) -> (w145:u16[])
            }
            frame "UploadSettings_pre" {
              # "When the Host sends settings,\nnot all files send at the same time.\n\nIf RT reads the settings faster\nthan the Host can send them,\nthen we will skip settings.\n\nSolution:\nWait 20 cycles"
              n53 = Increment(x=w162) -> (x+1=w161:u16)
              n54 = Greater?(x=w161, y=u16 20) -> (0:w159:bool)
              n55 = Select(t=myRIO_BRig_RT__Case_NonExp_stateList."UploadSettings_Read_dataExp", s=w159, f=w158) -> (s? t:f=w156:T1)
            }
            frame "UploadSettings_Read_dataExp" {
              # "grab dataExp and\nstore it in the\ngeneric data array"
              # "dataExp"
              n56 = call "myRIO_BRig_RT_dataExp_init_details.vi"() -> ("output_dataSize"=w169:i32, "output_dataName"=w172:string)  [unwired: 10 in]
              n57 = call "myRIO_BRig_RT_comm_webdav_uploadReceived_check.vi"("input_dataName"=w172) -> ("output_Iexist"=w171:bool, "output_dataPath"=w170:path)  [unwired: 9 in]
              n58 = case shown="True" w171 {
                tunnel: w170 -> [_ w181]
                tunnel: w169 -> [_ w180]
                tunnel: [_ w179] -> w168
                tunnel: w165 -> [w174 w178]
                tunnel: [w174 w175] -> w164
                frame False {
                }
                frame True {
                  n59 = call "myRIO_BRig_RT_comm_webdav_uploadReceived_read.vi"("input_dataSize"=w180, "input_filePath"=w181) -> ("output_Ivalid"=w179:bool, "output_data"=w177:i64[])  [unwired: 8 in]
                  n60 = To Unsigned Word Integer(number=w177) -> (unsigned 16bit integer=w176:u16[])
                  n61 = Select(t=w176, s=w179, f=w178) -> (s? t:f=w175:u16[])
                }
              }
              n62 = Select(t=myRIO_BRig_RT__Case_NonExp_stateList."UploadSettings_dataExp_1", s=w168, f=myRIO_BRig_RT__Case_NonExp_stateList."UploadSettings_Read_dataLC" ("t")) -> (s? t:f=w163:T1)
            }
            frame "UploadSettings_Read_dataLC" {
              # "grab dataLC and\nstore it in the\ngeneric data array"
              # "dataLC"
              n63 = call "myRIO_BRig_RT_dataLC_init_details.vi"() -> ("output_dataSize"=w188:i32, "output_dataName"=w191:string)  [unwired: 10 in]
              n64 = call "myRIO_BRig_RT_comm_webdav_uploadReceived_check.vi"("input_dataName"=w191) -> ("output_Iexist"=w190:bool, "output_dataPath"=w189:path)  [unwired: 9 in]
              n65 = case shown="True" w190 {
                tunnel: w189 -> [_ w200]
                tunnel: w188 -> [_ w199]
                tunnel: [_ w198] -> w187
                tunnel: w184 -> [w193 w197]
                tunnel: [w193 w194] -> w183
                frame False {
                }
                frame True {
                  n66 = call "myRIO_BRig_RT_comm_webdav_uploadReceived_read.vi"("input_dataSize"=w199, "input_filePath"=w200) -> ("output_Ivalid"=w198:bool, "output_data"=w196:i64[])  [unwired: 8 in]
                  n67 = To Unsigned Word Integer(number=w196) -> (unsigned 16bit integer=w195:u16[])
                  n68 = Select(t=w195, s=w198, f=w197) -> (s? t:f=w194:u16[])
                }
              }
              n69 = Select(t=myRIO_BRig_RT__Case_NonExp_stateList."UploadSettings_dataLC_1", s=w187, f=myRIO_BRig_RT__Case_NonExp_stateList."UploadSettings_Read_dataMTrig" ("t")) -> (s? t:f=w182:T1)
            }
            frame "UploadSettings_Read_dataMTrig" {
              # "grab dataMTrig and\nstore it in the\ngeneric data array"
              # "dataMTrig"
              n70 = call "myRIO_BRig_RT_dataMTrig_init_details.vi"() -> ("output_dataSize"=w207:i32, "output_dataName"=w210:string)  [unwired: 10 in]
              n71 = call "myRIO_BRig_RT_comm_webdav_uploadReceived_check.vi"("input_dataName"=w210) -> ("output_Iexist"=w209:bool, "output_dataPath"=w208:path)  [unwired: 9 in]
              n72 = case shown="True" w209 {
                tunnel: w208 -> [_ w219]
                tunnel: w207 -> [_ w218]
                tunnel: [_ w217] -> w206
                tunnel: w203 -> [w212 w216]
                tunnel: [w212 w213] -> w202
                frame False {
                }
                frame True {
                  n73 = call "myRIO_BRig_RT_comm_webdav_uploadReceived_read.vi"("input_dataSize"=w218, "input_filePath"=w219) -> ("output_Ivalid"=w217:bool, "output_data"=w215:i64[])  [unwired: 8 in]
                  n74 = To Unsigned Word Integer(number=w215) -> (unsigned 16bit integer=w214:u16[])
                  n75 = Select(t=w214, s=w217, f=w216) -> (s? t:f=w213:u16[])
                }
              }
              n76 = Select(t=myRIO_BRig_RT__Case_NonExp_stateList."UploadSettings_dataMTrig_1", s=w206, f=myRIO_BRig_RT__Case_NonExp_stateList."Idle" ("t")) -> (s? t:f=w201:T1)
            }
            frame "UploadSettings_dataExp_1" {
              w228 = 100.0 ("y")
              # "Freq"
              # "f_millisec2count"
              # "laser"
              # "Cue_max"
              # "Cue_min"
              # "CuePenalty"
              # "Timeout"
              # "Wrong"
              # "Selection"
              # "RewardPost"
              # "Reward_R"
              # "Reward_L"
              # "Tcycle"
              # "TPB_min_R"
              # "TPB_min_L"
              # "TPB_max_R"
              # "TPB_max_L"
              # "I_trialUntilReward"
              # "ENL_penalty"
              # "ENL_min"
              # "ENL_max"
              # "BUR_max"
              # "BUR_min"
              # "CueCycles"
              # "Audio_Freq_R"
              # "Audio_Freq_L"
              # "Audio_Amp_R"
              # "Audio_Amp_L"
              n77 = call "myRIO_BRig_RT_dataExp_FPGA_f_count2ms.vi"() -> ("output_FPGA_f_count2ms"=w242:i32)  [unwired: 11 in]
              n78 = call "myRIO_BRig_RT_dataExp_laser1_Freq.vi"() -> ("output_laser1_Freq"=w241:i32)  [unwired: 11 in]
              n79 = call "myRIO_BRig_RT_dataExp_CueCycles.vi"() -> ("output_CueCycles"=w288:i32)  [unwired: 11 in]
              n80 = call "myRIO_BRig_RT_dataExp_Audio_amp__R.vi"() -> ("output_Audio_amp__R"=w292:i32)  [unwired: 11 in]
              n81 = call "myRIO_BRig_RT_dataExp_Audio_amp__L.vi"() -> ("output_Audio_amp__L"=w294:i32)  [unwired: 11 in]
              n82 = call "myRIO_BRig_RT_dataExp_Tcycle_Reward__L.vi"() -> ("output_Tcycle_Reward__L"=w265:i32)  [unwired: 11 in]
              n83 = call "myRIO_BRig_RT_dataExp_Tcycle_Reward__R.vi"() -> ("output_Tcycle_Reward__R"=w264:i32)  [unwired: 11 in]
              n84 = call "myRIO_BRig_RT_dataExp_Tcycle_RewardPost.vi"() -> ("output_Tcycle_RewardPost"=w263:i32)  [unwired: 11 in]
              n85 = call "myRIO_BRig_RT_dataExp_BUR_min.vi"() -> ("output_BUR_min"=w285:i32)  [unwired: 11 in]
              n86 = call "myRIO_BRig_RT_dataExp_ENL_min.vi"() -> ("output_ENL_min"=w281:i32)  [unwired: 11 in]
              n87 = call "myRIO_BRig_RT_dataExp_TPB_max__L.vi"() -> ("output_TPB_max__L"=w273:i32)  [unwired: 11 in]
              n88 = call "myRIO_BRig_RT_dataExp_TPB_max__R.vi"() -> ("output_TPB_max__R"=w272:i32)  [unwired: 11 in]
              n89 = call "myRIO_BRig_RT_dataExp_ENL_penalty.vi"() -> ("output_ENL_penalty"=w280:i32)  [unwired: 11 in]
              n90 = call "myRIO_BRig_RT_dataExp_laser1_Power_min.vi"() -> ("output_laser1_Power_min"=w240:i32)  [unwired: 11 in]
              n91 = call "myRIO_BRig_RT_dataExp_laser1_Tpeak.vi"() -> ("output_laser1_Tpeak"=w239:i32)  [unwired: 11 in]
              n92 = call "myRIO_BRig_RT_dataExp_Audio_freq__L.vi"() -> ("output_Audio_freq__L"=w290:i32)  [unwired: 11 in]
              n93 = call "myRIO_BRig_RT_dataExp_Audio_freq__R.vi"() -> ("output_Audio_freq__R"=w289:i32)  [unwired: 11 in]
              n94 = call "myRIO_BRig_RT_dataExp_BUR_max.vi"() -> ("output_BUR_max"=w286:i32)  [unwired: 11 in]
              n95 = call "myRIO_BRig_RT_dataExp_ENL_max.vi"() -> ("output_ENL_max"=w282:i32)  [unwired: 11 in]
              n96 = call "myRIO_BRig_RT_dataExp_ItrialUntilReward.vi"() -> ("output_I_trialUntilReward"=w276:i32)  [unwired: 11 in]
              n97 = call "myRIO_BRig_RT_dataExp_Tcycle_Selection.vi"() -> ("output_Tcycle_Selection"=w262:i32)  [unwired: 11 in]
              n98 = call "myRIO_BRig_RT_dataExp_Tcycle_Wrong.vi"() -> ("output_Tcycle_Wrong"=w261:i32)  [unwired: 11 in]
              n99 = call "myRIO_BRig_RT_dataExp_Tcycle_Timeout.vi"() -> ("output_Tcycle_Timeout"=w260:i32)  [unwired: 11 in]
              n100 = call "myRIO_BRig_RT_dataExp_TPB_min__L.vi"() -> ("output_TPB_min__L"=w271:i32)  [unwired: 11 in]
              n101 = call "myRIO_BRig_RT_dataExp_TPB_min__R.vi"() -> ("output_TPB_min__R"=w270:i32)  [unwired: 11 in]
              n102 = call "myRIO_BRig_RT_dataExp_laser1_Tshutter.vi"() -> ("output_laser1_Tshutter"=w238:i32)  [unwired: 11 in]
              n103 = call "myRIO_BRig_RT_dataExp_laser1_duration.vi"() -> ("output_laser1_duration"=w237:i32)  [unwired: 11 in]
              n104 = call "myRIO_BRig_RT_dataExp_Tcycle_CuePenalty.vi"() -> ("output_Tcycle_CuePenalty"=w253:i32)  [unwired: 11 in]
              n105 = call "myRIO_BRig_RT_dataExp_Tcycle_Cue_min.vi"() -> ("output_Tcycle_Cue_min"=w252:i32)  [unwired: 11 in]
              n106 = call "myRIO_BRig_RT_dataExp_Tcycle_Cue_max.vi"() -> ("output_Tcycle_Cue_max"=w251:i32)  [unwired: 11 in]
              n107 = Index Array(array=w245, index #1=w294, index #2=w292, index #3=w290, index #4=w289, index #5=w288, index #6=w286, index #7=w285, index #8=w282, index #9=w281, index #10=w280, index #11=w276, index #12=w273, index #13=w272, index #14=w271, index #15=w270, index #16=w265, index #17=w264, index #18=w263, index #19=w262, index #20=w261, index #21=w260, index #22=w253, index #23=w252, index #24=w251, index #25=w242, index #26=w241, index #27=w240, index #28=w239, index #29=w238, index #30=w237) -> (element #1=w293:u16, element #2=w291:u16, element #3=w248:u16, element #4=w247:u16, element #5=w287:u16, element #6=w284:u16, element #7=w283:u16, element #8=w279:u16, element #9=w278:u16, element #10=w277:u16, element #11=w274:u16, element #12=w269:u16, element #13=w268:u16, element #14=w267:u16, element #15=w266:u16, element #16=w259:u16, element #17=w258:u16, element #18=w257:u16, element #19=w256:u16, element #20=w255:u16, element #21=w254:u16, element #22=w250:u16, element #23=w244:u16, element #24=w243:u16, element #25=w236:u16, element #26=w227:u16, element #27=w226:u16, element #28=w225:u16, element #29=w224:u16, element #30=w220:u16)
              n108 = To Double Precision Float(number=w236) -> (double precision float=w235:dbl)
              n109 = To Double Precision Float(number=w227) -> (double precision float=w233:dbl)
              n110 = To Double Precision Float(number=w226) -> (double precision float=w231:dbl)
              n111 = To Double Precision Float(number=w225) -> (double precision float=w230:dbl)
              n112 = To Double Precision Float(number=w224) -> (double precision float=w229:dbl)
              n113 = local write "Tcycle_Selection"(w256) -> ()
              n114 = local write "Tcycle_Wrong"(w255) -> ()
              n115 = local write "Tcycle_Timeout"(w254) -> ()
              n116 = local write "Audio_Amp__L"(w293) -> ()
              n117 = local write "Audio_Amp__R"(w291) -> ()
              n118 = Divide(x=w235, y=w228) -> (x/y=w234:dbl)
              n119 = Divide(x=w233, y=w228) -> (x/y=w232:dbl)
              n120 = Divide(x=w231, y=w228) -> (x/y=w223:dbl)
              n121 = Divide(x=w230, y=w228) -> (x/y=w222:dbl)
              n122 = Divide(x=w229, y=w228) -> (x/y=w221:dbl)
              n123 = local write "Tcycle_ENLPenalty"(w277) -> ()
              n124 = local write "Tcycle_ENL_max"(w279) -> ()
              n125 = local write "Laser_duration_l1"(w220) -> ()
              n126 = local write "Laser_power_min_l1"(w223) -> ()
              n127 = local write "TpB_Min_L"(w267) -> ()
              n128 = local write "TpB_Min_R"(w266) -> ()
              n129 = local write "Laser_Tshutter_l1"(w221) -> ()
              n130 = local write "Laser_Tpeak_l1"(w222) -> ()
              n131 = local write "Laser_Freq_l1"(w232) -> ()
              n132 = local write "FPGA_count2ms"(w234) -> ()
              n133 = local write "Tcycle_CuePenalty"(w250) -> ()
              n134 = local write "Tcycle_Cue_min"(w244) -> ()
              n135 = local write "Tcycle_Cue_max"(w243) -> ()
              n136 = To Unsigned Byte Integer(number=w248) -> (unsigned 8bit integer=w249:u8)
              n137 = To Unsigned Byte Integer(number=w247) -> (unsigned 8bit integer=w246:u8)
              n138 = Not Equal To 0?(x=w274) -> (x != 0?=w275:bool)
              n139 = local write "Tcycle_Reward_L"(w259) -> ()
              n140 = local write "Tcycle_Reward_R"(w258) -> ()
              n141 = local write "Tcycle_RewardPost"(w257) -> ()
              n142 = local write "CueCycles"(w287) -> ()
              n143 = local write "BUR_min"(w283) -> ()
              n144 = local write "BUR_max"(w284) -> ()
              n145 = local write "Tcycle_ENL_min"(w278) -> ()
              n146 = local write "TpB_Max_L"(w269) -> ()
              n147 = local write "TpB_Max_R"(w268) -> ()
              n148 = local write "TrialUntilReward"(w275) -> ()
              n149 = local write "Audio_Freq__L"(w249) -> ()
              n150 = local write "Audio_Freq__R"(w246) -> ()
            }
            frame "UploadSettings_dataLC_1" {
              # "Cue1_All_delayOpt"
              # "ENL1_All_delayOpt"
              # "Cue1_First_delayOpt"
              # "ENL1_First_delayOpt"
              # "ENL1 First"
              # "Cue1 All"
              # "Cue1 First"
              # "Count"
              # "Tdelay"
              # "Prob"
              # "OnOff"
              # "Block"
              # "ENL1 All"
              # "Count"
              # "Tdelay"
              # "Prob"
              # "OnOff"
              # "Block"
              # "Count"
              # "Tdelay"
              # "Prob"
              # "Block"
              # "OnOff"
              # "Count"
              # "Tdelay"
              # "Prob"
              # "OnOff"
              # "Block"
              n151 = call "myRIO_BRig_RT_dataLC_Cue1_Block_Switch_l1.vi"() -> ("output_Cue1_Block_Switch_l1"=w353:i32)  [unwired: 11 in]
              n152 = call "myRIO_BRig_RT_dataLC_Cue1_OnOff_Switch_l1.vi"() -> ("output_Cue1_OnOff_Switch_l1"=w351:i32)  [unwired: 11 in]
              n153 = call "myRIO_BRig_RT_dataLC_Cue1_Count_Switch_l1.vi"() -> ("output_Cue1_Count_Switch_l1"=w348:i32)  [unwired: 11 in]
              n154 = call "myRIO_BRig_RT_dataLC_Cue1_Block_NS_l1.vi"() -> ("output_Cue1_Block_NS_l1"=w335:i32)  [unwired: 11 in]
              n155 = call "myRIO_BRig_RT_dataLC_Cue1_OnOff_NS_l1.vi"() -> ("output_Cue1_OnOff_NS_l1"=w334:i32)  [unwired: 11 in]
              n156 = call "myRIO_BRig_RT_dataLC_Cue1_Count_NS_l1.vi"() -> ("output_Cue1_Count_NS_l1"=w345:i32)  [unwired: 11 in]
              n157 = call "myRIO_BRig_RT_dataLC_ENL1_Block_Switch_l1.vi"() -> ("output_ENL1_Block_Switch_l1"=w333:i32)  [unwired: 11 in]
              n158 = call "myRIO_BRig_RT_dataLC_ENL1_OnOff_Switch_l1.vi"() -> ("output_ENL1_OnOff_Switch_l1"=w344:i32)  [unwired: 11 in]
              n159 = call "myRIO_BRig_RT_dataLC_ENL1_Count_Switch_l1.vi"() -> ("output_ENL1_Count_Switch_l1"=w341:i32)  [unwired: 11 in]
              n160 = call "myRIO_BRig_RT_dataLC_ENL1_Block_NS_l1.vi"() -> ("output_ENL1_All_Block"=w340:i32)  [unwired: 11 in]
              n161 = call "myRIO_BRig_RT_dataLC_ENL1_OnOff_NS_l1.vi"() -> ("output_ENL1_OnOff_NS_l1"=w339:i32)  [unwired: 11 in]
              n162 = call "myRIO_BRig_RT_dataLC_ENL1_Count_NS_l1.vi"() -> ("output_ENL1_Count_NS_l1"=w336:i32)  [unwired: 11 in]
              n163 = call "myRIO_BRig_RT_dataLC_ENL1_delayOpt_Switch_l1.vi"() -> ("output_ENL1_delayOpt_Switch_l1"=w310:i32)  [unwired: 11 in]
              n164 = call "myRIO_BRig_RT_dataLC_Cue1_delayOpt_Switch_l1.vi"() -> ("output_Cue1_delayOpt_Switch_l1"=w309:i32)  [unwired: 11 in]
              n165 = call "myRIO_BRig_RT_dataLC_ENL1_delayOpt_NS_l1.vi"() -> ("output_ENL1_delayOpt_NS_l1"=w302:i32)  [unwired: 11 in]
              n166 = call "myRIO_BRig_RT_dataLC_Cue1_delayOpt_NS_l1.vi"() -> ("output_Cue1_delayOpt_NS_l1"=w301:i32)  [unwired: 11 in]
              n167 = call "myRIO_BRig_RT_dataLC_Cue1_Probability_Switch_l1.vi"() -> ("output_Cue1_Probability_Switch_l1"=w350:i32)  [unwired: 11 in]
              n168 = call "myRIO_BRig_RT_dataLC_Cue1_Tdelay_Switch_l1.vi"() -> ("output_Cue1_Tdelay_Switch_l1"=w349:i32)  [unwired: 11 in]
              n169 = call "myRIO_BRig_RT_dataLC_Cue1_Probability_NS_l1.vi"() -> ("output_Cue1_l1_All_Probability"=w347:i32)  [unwired: 11 in]
              n170 = call "myRIO_BRig_RT_dataLC_Cue1_Tdelay_NS_l1.vi"() -> ("output_Cue1_Tdelay_NS_l1"=w346:i32)  [unwired: 11 in]
              n171 = call "myRIO_BRig_RT_dataLC_ENL1_Probability_Switch_l1.vi"() -> ("output_ENL1_Probability_Switch_l1"=w343:i32)  [unwired: 11 in]
              n172 = call "myRIO_BRig_RT_dataLC_ENL1_Tdelay_Switch_l1.vi"() -> ("output_ENL1_Tdelay_Switch_l1"=w342:i32)  [unwired: 11 in]
              n173 = call "myRIO_BRig_RT_dataLC_ENL1_Probability_NS_l1.vi"() -> ("output_ENL1_Probability_NS_l1"=w338:i32)  [unwired: 11 in]
              n174 = call "myRIO_BRig_RT_dataLC_ENL1_Tdelay_NS_l1.vi"() -> ("output_ENL1_Tdelay_NS_l1"=w337:i32)  [unwired: 11 in]
              n175 = Index Array(array=w311, index #1=w353, index #2=w351, index #3=w350, index #4=w349, index #5=w348, index #6=w335, index #7=w334, index #8=w347, index #9=w346, index #10=w345, index #11=w333, index #12=w344, index #13=w343, index #14=w342, index #15=w341, index #16=w340, index #17=w339, index #18=w338, index #19=w337, index #20=w336, index #21=w310, index #22=w309, index #23=w302, index #24=w301) -> (element #1=w352:u16, element #2=w331:u16, element #3=w330:u16, element #4=w329:u16, element #5=w328:u16, element #6=w324:u16, element #7=w323:u16, element #8=w322:u16, element #9=w321:u16, element #10=w320:u16, element #11=w319:u16, element #12=w318:u16, element #13=w317:u16, element #14=w316:u16, element #15=w303:u16, element #16=w315:u16, element #17=w314:u16, element #18=w313:u16, element #19=w312:u16, element #20=w304:u16, element #21=w307:u16, element #22=w305:u16, element #23=w298:u16, element #24=w297:u16)
              n176 = Not Equal To 0?(x=w298) -> (x != 0?=w300:bool)
              n177 = Not Equal To 0?(x=w297) -> (x != 0?=w299:bool)
              n178 = Not Equal To 0?(x=w307) -> (x != 0?=w308:bool)
              n179 = Not Equal To 0?(x=w305) -> (x != 0?=w306:bool)
              n180 = local write "LC_Cue1_Probability_Switch_l1"(w330) -> ()
              n181 = local write "LC_ENL1_Probability_Switch_l1"(w317) -> ()
              n182 = Not Equal To 0?(x=w331) -> (x != 0?=w332:bool)
              n183 = Not Equal To 0?(x=w323) -> (x != 0?=w327:bool)
              n184 = local write "LC_ENL1_delayOpt_Switch_l1"(w308) -> ()
              n185 = local write "LC_Cue1_delayOpt_Switch_l1"(w306) -> ()
              n186 = Not Equal To 0?(x=w318) -> (x != 0?=w326:bool)
              n187 = Not Equal To 0?(x=w314) -> (x != 0?=w325:bool)
              n188 = local write "LC_Cue1_Tdelay_Switch_l1"(w329) -> ()
              n189 = local write "LC_Cue1_OnOff_Switch_l1"(w332) -> ()
              n190 = local write "LC_Cue1_Count_Switch_l1"(w328) -> ()
              n191 = local write "LC_Cue1_Block_Switch_l1"(w352) -> ()
              n192 = local write "LC_Cue1_Probability_NS_l1"(w322) -> ()
              n193 = local write "LC_ENL1_delayOpt_NS_l1"(w300) -> ()
              n194 = local write "LC_Cue1_delayOpt_NS_l1"(w299) -> ()
              n195 = local write "LC_ENL1_Tdelay_Switch_l1"(w316) -> ()
              n196 = local write "LC_ENL1_OnOff_Switch_l1"(w326) -> ()
              n197 = local write "LC_ENL1_Count_Switch_l1"(w303) -> ()
              n198 = local write "LC_ENL1_Probability_NS_l1"(w313) -> ()
              n199 = local write "LC_ENL1_Block_Switch_l1"(w319) -> ()
              n200 = local write "LC_Cue1_Tdelay_NS_l1"(w321) -> ()
              n201 = local write "LC_Cue1_OnOff_NS_l1"(w327) -> ()
              n202 = local write "LC_Cue1_Count_NS_l1"(w320) -> ()
              n203 = local write "LC_Cue1_Block_NS_l1"(w324) -> ()
              n204 = local write "LC_ENL1_Tdelay_NS_l1"(w312) -> ()
              n205 = local write "LC_ENL1_OnOff_NS_l1"(w325) -> ()
              n206 = local write "LC_ENL1_Count_NS_l1"(w304) -> ()
              n207 = local write "LC_ENL1_Block_NS_l1"(w315) -> ()
            }
            frame "UploadSettings_dataLC_2" {
              # "Wrong"
              # "Reward"
              # "Trial"
              # "Tdelay"
              # "Prob"
              # "Block"
              # "OnOff"
              # "Trial"
              # "Tdelay"
              # "Prob"
              # "OnOff"
              # "Block"
              n208 = call "myRIO_BRig_RT_dataLC_Reward_Block_l1.vi"() -> ("output_Reward_Block_l1"=w378:i32)  [unwired: 11 in]
              n209 = call "myRIO_BRig_RT_dataLC_Reward_OnOff_l1.vi"() -> ("output_Reward_OnOff_l1"=w376:i32)  [unwired: 11 in]
              n210 = call "myRIO_BRig_RT_dataLC_Reward_Trial_l1.vi"() -> ("output_Reward_Trial_l1"=w373:i32)  [unwired: 11 in]
              n211 = call "myRIO_BRig_RT_dataLC_Wrong_Block_l1.vi"() -> ("output_Wrong_Block_l1"=w369:i32)  [unwired: 11 in]
              n212 = call "myRIO_BRig_RT_dataLC_Wrong_OnOff_l1.vi"() -> ("output_Wrong_OnOff_l1"=w368:i32)  [unwired: 11 in]
              n213 = call "myRIO_BRig_RT_dataLC_Wrong_Trial_l1.vi"() -> ("output_Wrong_Trial_l1"=w370:i32)  [unwired: 11 in]
              n214 = call "myRIO_BRig_RT_dataLC_Reward_Probability_l1.vi"() -> ("output_Reward_Probability_l1"=w375:i32)  [unwired: 11 in]
              n215 = call "myRIO_BRig_RT_dataLC_Reward_Tdelay_l1.vi"() -> ("output_Reward_Tdelay_l1"=w374:i32)  [unwired: 11 in]
              n216 = call "myRIO_BRig_RT_dataLC_Wrong_Probability_l1.vi"() -> ("output_Wrong_Probability_l1"=w372:i32)  [unwired: 11 in]
              n217 = call "myRIO_BRig_RT_dataLC_Wrong_Tdelay_l1.vi"() -> ("output_Wrong_Tdelay_l1"=w371:i32)  [unwired: 11 in]
              n218 = Index Array(array=w356, index #1=w378, index #2=w376, index #3=w375, index #4=w374, index #5=w373, index #6=w369, index #7=w368, index #8=w372, index #9=w371, index #10=w370) -> (element #1=w377:u16, element #2=w366:u16, element #3=w365:u16, element #4=w364:u16, element #5=w363:u16, element #6=w361:u16, element #7=w360:u16, element #8=w359:u16, element #9=w358:u16, element #10=w357:u16)
              n219 = Not Equal To 0?(x=w366) -> (x != 0?=w367:bool)
              n220 = Not Equal To 0?(x=w360) -> (x != 0?=w362:bool)
              n221 = local write "LC_Reward_Probability_l1"(w365) -> ()
              n222 = local write "LC_Wrong_Probability_l1"(w359) -> ()
              n223 = local write "LC_Reward_Tdelay_l1"(w364) -> ()
              n224 = local write "LC_Reward_OnOff_l1"(w367) -> ()
              n225 = local write "LC_Reward_Block_l1"(w377) -> ()
              n226 = local write "LC_Reward_Trial_l1"(w363) -> ()
              n227 = local write "LC_Wrong_Tdelay_l1"(w358) -> ()
              n228 = local write "LC_Wrong_OnOff_l1"(w362) -> ()
              n229 = local write "LC_Wrong_Block_l1"(w361) -> ()
              n230 = local write "LC_Wrong_Trial_l1"(w357) -> ()
            }
            frame "UploadSettings_dataMTrig_1" {
              # "Tdelay_R"
              # "Tdelay_L"
              # "Tcycle_R"
              # "Tcycle_L"
              # "RewCalib_nCycle_R"
              # "RewCalib_nCycle_L"
              # "Solenoid"
              # "Laser_Tcycle"
              n231 = call "myRIO_BRig_RT_dataMTrig_Laser_Tcycle.vi"() -> ("output_Laser_Tcycle"=w388:i32)  [unwired: 11 in]
              n232 = call "myRIO_BRig_RT_dataMTrig_Solenoid_RewCalib_nCycle__L.vi"() -> ("output_Solenoid_RewCalib_nCycle__L"=w387:i32)  [unwired: 11 in]
              n233 = call "myRIO_BRig_RT_dataMTrig_Solenoid_RewCalib_nCycle__R.vi"() -> ("output_Solenoid_RewCalib_nCycle__R"=w386:i32)  [unwired: 11 in]
              n234 = call "myRIO_BRig_RT_dataMTrig_Solenoid_Tdelay__L.vi"() -> ("output_Solenoid_Tdelay__L"=w383:i32)  [unwired: 11 in]
              n235 = call "myRIO_BRig_RT_dataMTrig_Solenoid_Tdelay__R.vi"() -> ("output_Solenoid_Tdelay__R"=w382:i32)  [unwired: 11 in]
              n236 = call "myRIO_BRig_RT_dataMTrig_Solenoid_Tcycle__L.vi"() -> ("output_Solenoid_Tcycle__L"=w385:i32)  [unwired: 11 in]
              n237 = call "myRIO_BRig_RT_dataMTrig_Solenoid_Tcycle__R.vi"() -> ("output_Solenoid_Tcycle__R"=w384:i32)  [unwired: 11 in]
              n238 = Index Array(array=w381, index #1=w388, index #2=w387, index #3=w386, index #4=w385, index #5=w384, index #6=w383, index #7=w382) -> (element #1=w395:u16, element #2=w394:u16, element #3=w393:u16, element #4=w392:u16, element #5=w391:u16, element #6=w390:u16, element #7=w389:u16)
              n239 = Replace Array Subset(array=w397, new element #1=w395, index #1=w388, new element #2=w394, index #2=w387, new element #3=w393, index #3=w386, new element #4=w392, index #4=w385, new element #5=w391, index #5=w384, new element #6=w390, index #6=w383, new element #7=w389, index #7=w382) -> (w396:u16[])
              n240 = local write "MTrig_Solenoid_Tcycle__L"(w392) -> ()
              n241 = local write "MTrig_Solenoid_Tcycle__R"(w391) -> ()
              n242 = local write "MTrig_Laser_Tcycle"(w395) -> ()
            }
            frame "Idle" {
              # "To ensure timing, we split the\nidle state into 4 phases"
              # "Laser_Tcycle"
              # "Audio_Tcycle_R"
              # "Audio_Tcycle_L"
              n243 = local read "Laser_power_min_l1"() -> (w402:dbl)
              n244 = local read "Laser_power_min_l2"() -> (w400:dbl)
              n245 = local read "FPGA_count2ms"() -> (w410:dbl)
              n246 = local read "Audio_Amp__R"() -> (w404:u16)
              n247 = local read "Audio_Amp__L"() -> (w406:u16)
              n248 = local read "Audio_Freq__R"() -> (w403:u8)
              n249 = local read "Audio_Freq__L"() -> (w405:u8)
              n250 = Select(t=myRIO_BRig_RT__Case_NonExp_stateList."SendData" ("Enum"), s="SendData", f=myRIO_BRig_RT__Case_NonExp_stateList."Idle_2" ("Enum")) -> (s? t:f=w413:T1)
              n251 = call "myRIO__convert__Voltage_to_FPGAvalue.vi"("input_voltage"=w402) -> ("output_PortC"=w401:i16)  [unwired: 9 in, 1 out]
              n252 = call "myRIO__convert__Voltage_to_FPGAvalue.vi"("input_voltage"=w400) -> ("output_PortC"=w399:i16)  [unwired: 9 in, 1 out]
              n253 = To Unsigned Word Integer(number=w410) -> (unsigned 16bit integer=w409:u16)
              n254 = xnode "Read/Write Control"("FPGA VI Reference In"=w408, "error in"=w407, "k1__counter_per_ms"=w409, "audioAmp_L"=w406, "audioFreq_L_kHz"=w405, "audioAmp_R"=w404, "audioFreq_R_kHz"=w403, "AnaOut_0"=w401, "AnaOut_1"=w399) -> ()  [unwired: 2 out]
              n255 = Select(t=myRIO_BRig_RT__Case_NonExp_stateList."TestConnection" ("Enum"), s="TestConnection", f=w413) -> (s? t:f=w418:T1)
              n256 = call "myRIO_BRig_RT_dataMTrig_Audio_Tcycle__L.vi"() -> ("output_Audio_Tcycle__L"=w425:i32)  [unwired: 11 in]
              n257 = call "myRIO_BRig_RT_dataMTrig_Audio_Tcycle__R.vi"() -> ("output_Audio_Tcycle__R"=w424:i32)  [unwired: 11 in]
              n258 = call "myRIO_BRig_RT_dataMTrig_Laser_Tcycle.vi"() -> ("output_Laser_Tcycle"=w423:i32)  [unwired: 11 in]
              n259 = local read "MTrig_Laser_Tcycle"() -> (w411:u16)
              n260 = local read "Tcycle_Cue_min"() -> (w412:u16)
              n261 = Replace Array Subset(array=w421, new element #1=w412, index #1=w425, new element #2=w412, index #2=w424, new element #3=w411, index #3=w423) -> (w422:u16[])
            }
            frame "Idle_2" {
              w427 = u16 0 ("t")
              # "To ensure timing, we split the\nidle state into 4 phases"
              # "Ncycles"
              # "Ncycles"
              # "RewCalib"
              # "RewCalib"
              # "Solenoid R"
              # "Solenoid L"
              n262 = call "myRIO_BRig_RT_dataMTrig_Solenoid_RewCalib_OnOff__L.vi"() -> ("output_Solenoid_RewCalib_OnOff__L"=w458:i32)  [unwired: 11 in]
              n263 = call "myRIO_BRig_RT_dataMTrig_Solenoid_N__L.vi"() -> ("output_Solenoid_N__L"=w446:i32)  [unwired: 11 in]
              n264 = call "myRIO_BRig_RT_dataMTrig_Solenoid_RewCalib_OnOff__R.vi"() -> ("output_Solenoid_RewCalib_OnOff__R"=w443:i32)  [unwired: 11 in]
              n265 = call "myRIO_BRig_RT_dataMTrig_Solenoid_N__R.vi"() -> ("output_Solenoid_N__R"=w442:i32)  [unwired: 11 in]
              n266 = Index Array(array=w449, index #1=w458, index #2=w446, index #3=w443, index #4=w442) -> (element #1=w445:u16, element #2=w440:u16, element #3=w441:u16, element #4=w439:u16)
              n267 = local read "RewCalib_Trig_L"() -> (w438:bool)
              n268 = local read "RewCalib_Trig_R"() -> (w437:bool)
              n269 = Equal To 0?(x=w440) -> (x = 0?=w448:bool)
              n270 = Equal To 0?(x=w439) -> (x = 0?=w447:bool)
              n271 = Not Equal To 0?(x=w441) -> (x != 0?=w459:bool)
              n272 = Not Equal To 0?(x=w445) -> (x != 0?=w460:bool)
              n273 = And(x=w448, y=w447) -> (x .and. y?=w452:bool)
              n274 = Or(x=w438, y=w437) -> (x .or. y?=w453:bool)
              n275 = Not Exclusive Or(1:w460, 2:w438) -> (0:w455:bool)
              n276 = Not Exclusive Or(1:w459, 2:w437) -> (0:w457:bool)
              n277 = And(x=w453, y=w452) -> (x .and. y?=w435:bool)
              n278 = Not(x=w455) -> (.not. x?=w454:bool)
              n279 = Not(x=w457) -> (.not. x?=w456:bool)
              n280 = Or(x=w454, y=w456) -> (x .or. y?=w436:bool)
              n281 = Or(x=w435, y=w436) -> (x .or. y?=w451:bool)
              n282 = local read "count_warmup_R"() -> (w426:u16)
              n283 = local read "count_warmup_L"() -> (w431:u16)
              n284 = Select(t=myRIO_BRig_RT__Case_NonExp_stateList."RewardCalibration_pre" ("Enum"), s=w451, f=myRIO_BRig_RT__Case_NonExp_stateList."Idle_3" ("Enum")) -> (s? t:f=w434:T1)
              n285 = Select(t=w427, s="count_warmup_L_reset", f=w431) -> (s? t:f=→"count_warmup_L":u16)
              n286 = Select(t=w427, s="count_warmup_R_reset", f=w426) -> (s? t:f=→"count_warmup_R":u16)
            }
            frame "Idle_3" {
              w483 = u8 0 ("f")
              # "To ensure timing, we split the\nidle state into 4 phases"
              n287 = local read "MTrig_Solenoid_trig__L"() -> (w474:bool)
              n288 = local read "MTrig_Solenoid_trig__R"() -> (w484:bool)
              n289 = local read "warmupType"() -> (w466:u8)
              n290 = local read "warmup"() -> (w476:bool)
              n291 = Not Equal To 0?(x=w466) -> (x != 0?=w465:bool)
              n292 = Not(x=w465) -> (.not. x?=w477:bool)
              n293 = Select(t=u8 1, s=w474, f=w483) -> (s? t:f=w482:u8)
              n294 = Select(t=u8 2, s=w484, f=w483) -> (s? t:f=w481:u8)
              n295 = And(x=w476, y=w477) -> (x .and. y?=w475:bool)
              n296 = And(x=w476, y=w465) -> (x .and. y?=w470:bool)
              n297 = Add(x=w482, y=w481) -> (x+y=w480:u8)
              n298 = case shown="3" w480 {
                tunnel: w479 -> [w487 w491 w509 w527]
                tunnel: [w487 w490 w508 w526] -> w478
                tunnel: w475 -> [_ w489 w507 w525]
                tunnel: [_ TRUE TRUE TRUE] -> w472
                frame 0, Default {
                }
                frame 1 {
                  n299 = case shown="True" w489 {
                    tunnel: w491 -> [w500 w505]
                    tunnel: [w499 w504] -> w490
                    frame True {
                      # "Audio_L"
                      # "Solenoid_L"
                      n300 = call "myRIO_BRig_RT_dataMTrig_Solenoid_N__L.vi"() -> ("output_Solenoid_N__L"=w496:i32)  [unwired: 11 in]
                      n301 = call "myRIO_BRig_RT_dataMTrig_Audio_N__L.vi"() -> ("output_Audio_N__L"=w494:i32)  [unwired: 11 in]
                      n302 = Index Array(array=w500, index #1=w496, index #2=w494) -> (element #1=w498:u16, element #2=w497:u16)
                      n303 = Increment(x=w498) -> (x+1=w495:u16)
                      n304 = Increment(x=w497) -> (x+1=w493:u16)
                      n305 = Replace Array Subset(array=w500, new element #1=w495, index #1=w496, new element #2=w493, index #2=w494) -> (w499:u16[])
                    }
                    frame False {
                      # "Solenoid_L"
                      n306 = call "myRIO_BRig_RT_dataMTrig_Solenoid_N__L.vi"() -> ("output_Solenoid_N__L"=w502:i32)  [unwired: 11 in]
                      n307 = Index Array(array=w505, index=w502) -> (element=w503:u16)
                      n308 = Increment(x=w503) -> (x+1=w501:u16)
                      n309 = Replace Array Subset(array=w505, new element=w501, index=w502) -> (w504:u16[])
                    }
                  }
                  n310 = local write "MTrig_Solenoid_trig__L"(FALSE) -> ()
                }
                frame 2 {
                  n311 = case shown="True" w507 {
                    tunnel: w509 -> [w518 w523]
                    tunnel: [w517 w522] -> w508
                    frame True {
                      # "Audio_R"
                      # "Solenoid_R"
                      n312 = call "myRIO_BRig_RT_dataMTrig_Solenoid_N__R.vi"() -> ("output_Solenoid_N__R"=w514:i32)  [unwired: 11 in]
                      n313 = call "myRIO_BRig_RT_dataMTrig_Audio_N__R.vi"() -> ("output_Audio_N__R"=w513:i32)  [unwired: 11 in]
                      n314 = Index Array(array=w518, index #1=w514, index #2=w513) -> (element #1=w516:u16, element #2=w515:u16)
                      n315 = Increment(x=w515) -> (x+1=w511:u16)
                      n316 = Increment(x=w516) -> (x+1=w512:u16)
                      n317 = Replace Array Subset(array=w518, new element #1=w512, index #1=w514, new element #2=w511, index #2=w513) -> (w517:u16[])
                    }
                    frame False {
                      # "Solenoid_R"
                      n318 = call "myRIO_BRig_RT_dataMTrig_Solenoid_N__R.vi"() -> ("output_Solenoid_N__R"=w519:i32)  [unwired: 11 in]
                      n319 = Index Array(array=w523, index=w519) -> (element=w521:u16)
                      n320 = Increment(x=w521) -> (x+1=w520:u16)
                      n321 = Replace Array Subset(array=w523, new element=w520, index=w519) -> (w522:u16[])
                    }
                  }
                  n322 = local write "MTrig_Solenoid_trig__R"(FALSE) -> ()
                }
                frame 3 {
                  w528 = FALSE
                  n323 = case shown="True" w525 {
                    tunnel: w527 -> [w542 w550]
                    tunnel: [w541 w549] -> w526
                    frame True {
                      # "Audio_R"
                      # "Solenoid_R"
                      # "Audio_L"
                      # "Solenoid_L"
                      n324 = call "myRIO_BRig_RT_dataMTrig_Solenoid_N__L.vi"() -> ("output_Solenoid_N__L"=w536:i32)  [unwired: 11 in]
                      n325 = call "myRIO_BRig_RT_dataMTrig_Audio_N__L.vi"() -> ("output_Audio_N__L"=w534:i32)  [unwired: 11 in]
                      n326 = call "myRIO_BRig_RT_dataMTrig_Solenoid_N__R.vi"() -> ("output_Solenoid_N__R"=w532:i32)  [unwired: 11 in]
                      n327 = call "myRIO_BRig_RT_dataMTrig_Audio_N__R.vi"() -> ("output_Audio_N__R"=w531:i32)  [unwired: 11 in]
                      n328 = Index Array(array=w542, index #1=w536, index #2=w534, index #3=w532, index #4=w531) -> (element #1=w540:u16, element #2=w539:u16, element #3=w538:u16, element #4=w537:u16)
                      n329 = Increment(x=w537) -> (x+1=w529:u16)
                      n330 = Increment(x=w540) -> (x+1=w535:u16)
                      n331 = Increment(x=w539) -> (x+1=w533:u16)
                      n332 = Increment(x=w538) -> (x+1=w530:u16)
                      n333 = Replace Array Subset(array=w542, new element #1=w535, index #1=w536, new element #2=w533, index #2=w534, new element #3=w530, index #3=w532, new element #4=w529, index #4=w531) -> (w541:u16[])
                    }
                    frame False {
                      # "Solenoid_R"
                      # "Solenoid_L"
                      n334 = call "myRIO_BRig_RT_dataMTrig_Solenoid_N__L.vi"() -> ("output_Solenoid_N__L"=w546:i32)  [unwired: 11 in]
                      n335 = call "myRIO_BRig_RT_dataMTrig_Solenoid_N__R.vi"() -> ("output_Solenoid_N__R"=w543:i32)  [unwired: 11 in]
                      n336 = Index Array(array=w550, index #1=w546, index #2=w543) -> (element #1=w548:u16, element #2=w547:u16)
                      n337 = Increment(x=w548) -> (x+1=w545:u16)
                      n338 = Increment(x=w547) -> (x+1=w544:u16)
                      n339 = Replace Array Subset(array=w550, new element #1=w545, index #1=w546, new element #2=w544, index #2=w543) -> (w549:u16[])
                    }
                  }
                  n340 = local write "MTrig_Solenoid_trig__L"(w528) -> ()
                  n341 = local write "MTrig_Solenoid_trig__R"(w528) -> ()
                }
              }
              n342 = local read "get_countPerMS"() -> (w464:bool)
              n343 = Select(t=myRIO_BRig_RT__Case_NonExp_stateList."Get_FPGA_count_per_ms" ("Enum"), s=w464, f=myRIO_BRig_RT__Case_NonExp_stateList."Idle_4" ("Enum")) -> (s? t:f=w462:T1)
              n344 = Select(t=myRIO_BRig_RT__Case_NonExp_stateList."Cue_pre", s=w470, f=myRIO_BRig_RT__Case_NonExp_stateList."DispenseWater_pre" ("Enum")) -> (s? t:f=w468:T1)
              n345 = Select(t=w468, s=w472, f=w462) -> (s? t:f=w473:T1)
            }
            frame "Idle_4" {
              # "use dataMTrig as it is one of the last to transfer"
              # "To ensure timing, we split the\nidle state into 4 phases"
              n346 = call "myRIO_BRig_RT_comm_webdav_uploadReceived_check_v2,0.vi"("input_dataName"="dataMTrig") -> ("output_Iexist"=w556:bool)  [unwired: 9 in, 1 out]
              n347 = Select(t=myRIO_BRig_RT__Case_NonExp_stateList."UploadSettings_pre" ("Enum"), s=w556, f=myRIO_BRig_RT__Case_NonExp_stateList."Idle") -> (s? t:f=w554:T1)
            }
            frame "Cue_pre" {
              w566 = u16 1 ("t")
              w565 = u16 0 ("new element/subarray")
              w562 = u16 0 ("new element/subarray")
              # "Ncycle"
              # "count"
              # "Audio_R"
              # "Solenoid_R"
              # "Solenoid_L"
              # "Ncycle"
              # "count"
              # "Audio_L"
              n348 = call "myRIO_BRig_RT_dataMTrig_Solenoid_N__L.vi"() -> ("output_Solenoid_N__L"=w575:i32)  [unwired: 11 in]
              n349 = call "myRIO_BRig_RT_dataMTrig_Solenoid_N__R.vi"() -> ("output_Solenoid_N__R"=w574:i32)  [unwired: 11 in]
              n350 = Index Array(array=w571, index #1=w575, index #2=w574) -> (element #1=w573:u16, element #2=w572:u16)
              n351 = Not Equal To 0?(x=w572) -> (x != 0?=w558:bool)
              n352 = Not Equal To 0?(x=w573) -> (x != 0?=w559:bool)
              n353 = Select(t=w566, s=w559, f=w565) -> (s? t:f=w567:u16)
              n354 = Select(t=w566, s=w558, f=w565) -> (s? t:f=w561:u16)
              n355 = call "myRIO_BRig_RT_dataMTrig_Audio_c__L.vi"() -> ("output_Audio_c__L"=w569:i32)  [unwired: 11 in]
              n356 = call "myRIO_BRig_RT_dataMTrig_Audio_N__L.vi"() -> ("output_Audio_N__L"=w568:i32)  [unwired: 11 in]
              n357 = call "myRIO_BRig_RT_dataMTrig_Audio_c__R.vi"() -> ("output_Audio_c__R"=w564:i32)  [unwired: 11 in]
              n358 = call "myRIO_BRig_RT_dataMTrig_Audio_N__R.vi"() -> ("output_Audio_N__R"=w563:i32)  [unwired: 11 in]
              n359 = Replace Array Subset(array=w571, new element #1=w562, index #1=w569, new element #2=w567, index #2=w568, new element #3=w562, index #3=w564, new element #4=w561, index #4=w563) -> (w570:u16[])
            }
            frame "Cue" {
              # "lick did not occur or warmupType==1"
              # "lick occurred?"
              # "Ncycle"
              # "Audio_R"
              # "Ncycle"
              # "Audio_L"
              n360 = local read "warmupType"() -> (w585:u8)
              n361 = Greater?(x=w591, y=w590) -> (0:w594:bool)
              n362 = Greater?(x=w593, y=w592) -> (0:w589:bool)
              n363 = Or(x=w589, y=w594) -> (x .or. y?=w583:bool)
              n364 = Equal?(x=w585, y=u8 1) -> (x = y?=w579:bool)
              n365 = Not(x=w583) -> (.not. x?=w582:bool)
              n366 = call "myRIO_BRig_RT_dataMTrig_Audio_N__L.vi"() -> ("output_Audio_N__L"=w597:i32)  [unwired: 11 in]
              n367 = call "myRIO_BRig_RT_dataMTrig_Audio_N__R.vi"() -> ("output_Audio_N__R"=w596:i32)  [unwired: 11 in]
              n368 = Or(x=w582, y=w579) -> (x .or. y?=w580:bool)
              n369 = case shown="True" w580 {
                tunnel: w597 -> [w603 w621]
                tunnel: w596 -> [w602 w620]
                tunnel: w588 -> [w605 w615]
                tunnel: [w604 w615] -> w587
                tunnel: w586 -> [_ w613]
                tunnel: [myRIO_BRig_RT__Case_NonExp_stateList."Idle" ("t") w612] -> w581
                tunnel: w579 -> [_ w611]
                tunnel: w578 -> [_ w607]
                tunnel: w577 -> [_ w606]
                frame False {
                  w598 = u16 0 ("new element/subarray")
                  # "lick occurred and warmupType==2"
                  n370 = call "myRIO_BRig_RT_dataMTrig_Solenoid_N__R.vi"() -> ("output_Solenoid_N__R"=w599:i32)  [unwired: 11 in]
                  n371 = call "myRIO_BRig_RT_dataMTrig_Solenoid_N__L.vi"() -> ("output_Solenoid_N__L"=w600:i32)  [unwired: 11 in]
                  n372 = Replace Array Subset(array=w605, new element #1=w598, index #1=w603, new element #2=w598, index #2=w602, new element #3=w598, index #3=w600, new element #4=w598, index #4=w599) -> (w604:u16[])
                }
                frame True {
                  n373 = Not(x=w611) -> (.not. x?=w610:bool)
                  n374 = Index Array(array=w615, index #1=w621, index #2=w620) -> (element #1=w619:u16, element #2=w618:u16)
                  n375 = Equal To 0?(x=w619) -> (x = 0?=w617:bool)
                  n376 = Equal To 0?(x=w618) -> (x = 0?=w616:bool)
                  n377 = And(x=w617, y=w616) -> (x .and. y?=w609:bool)
                  n378 = And(x=w609, y=w610) -> (x .and. y?=w608:bool)
                  n379 = case shown="True" w608 {
                    tunnel: w607 -> [_ w629]
                    tunnel: w606 -> [_ w624]
                    frame False {
                    }
                    frame True {
                      n380 = local read "count_warmup_R"() -> (w622:u16)
                      n381 = local read "count_warmup_L"() -> (w627:u16)
                      n382 = Increment(x=w622) -> (x+1=w625:u16)
                      n383 = Increment(x=w627) -> (x+1=w628:u16)
                      n384 = Select(t=w625, s=w624, f=w622) -> (s? t:f=w623:u16)
                      n385 = Select(t=w628, s=w629, f=w627) -> (s? t:f=w626:u16)
                      n386 = local write "count_warmup_R"(w623) -> ()
                      n387 = local write "count_warmup_L"(w626) -> ()
                    }
                  }
                  n388 = Select(t=myRIO_BRig_RT__Case_NonExp_stateList."DispenseWater_pre", s=w609, f=w613) -> (s? t:f=w612:T1)
                }
              }
            }
            frame "RewardCalibration_pre" {
              (unwired) FALSE
              w631 = FALSE
              w642 = u8 0
              w658 = u8 0
              # "Are we starting a RewardCalibration?\nOr are we stopping a RewardCalibration?\nOr is a RewardCalibration over?"
              # "RewCalib\nOnOff"
              # "N"
              # "Solenoid R"
              # "RewCalib\nOnOff"
              # "N"
              # "Solenoid L"
              n389 = local read "RewCalib_Trig_L"() -> (w665:bool)
              n390 = local read "RewCalib_Trig_R"() -> (w634:bool)
              n391 = call "myRIO_BRig_RT_dataMTrig_Solenoid_N__R.vi"() -> ("output_Solenoid_N__R"=w636:i32)  [unwired: 11 in]
              n392 = call "myRIO_BRig_RT_dataMTrig_Solenoid_RewCalib_OnOff__R.vi"() -> ("output_Solenoid_RewCalib_OnOff__R"=w633:i32)  [unwired: 11 in]
              n393 = call "myRIO_BRig_RT_dataMTrig_Solenoid_N__L.vi"() -> ("output_Solenoid_N__L"=w651:i32)  [unwired: 11 in]
              n394 = call "myRIO_BRig_RT_dataMTrig_Solenoid_RewCalib_OnOff__L.vi"() -> ("output_Solenoid_RewCalib_OnOff__L"=w652:i32)  [unwired: 11 in]
              n395 = Index Array(array=w635, index #1=w636, index #2=w633) -> (element #1=w646:u16, element #2=w641:u16)
              n396 = Index Array(array=w635, index #1=w651, index #2=w652) -> (element #1=w662:u16, element #2=w657:u16)
              n397 = Equal To 0?(x=w646) -> (x = 0?=w647:bool)
              n398 = Not Equal To 0?(x=w641) -> (x != 0?=w644:bool)
              n399 = Equal To 0?(x=w662) -> (x = 0?=w663:bool)
              n400 = Not Equal To 0?(x=w657) -> (x != 0?=w660:bool)
              n401 = local write "MTrig_Solenoid_trig__L"(w631) -> ()
              n402 = local write "MTrig_Solenoid_trig__R"(w631) -> ()
              n403 = Select(t=u8 1, s=w634, f=w642) -> (s? t:f=w638:u8)
              n404 = Select(t=u8 1, s=w665, f=w658) -> (s? t:f=w654:u8)
              n405 = Select(t=u8 2, s=w647, f=w642) -> (s? t:f=w639:u8)
              n406 = Select(t=u8 4, s=w644, f=w642) -> (s? t:f=w640:u8)
              n407 = Select(t=u8 2, s=w663, f=w658) -> (s? t:f=w655:u8)
              n408 = Select(t=u8 4, s=w660, f=w658) -> (s? t:f=w656:u8)
              n409 = Compound Arithmetic op=ADD(w638, w639, w640) -> (w637:u8)
              n410 = Compound Arithmetic op=ADD(w654, w655, w656) -> (w653:u8)
              n411 = case shown="7" w653 {
                tunnel: w635 -> [w695 w700 w702 w707 w712 w714 w717 w722]
                tunnel: [w695 w701 w702 w708 w713 w714 w718 w723] -> w650
                tunnel: w652 -> [_ w698 _ w705 w710 _ w716 w721]
                tunnel: w651 -> [_ w699 _ w706 w711 _ _ _]
                frame 0, Default {
                }
                frame 1 {
                  n412 = Replace Array Subset(array=w700, new element #1=u16 100 ("new element/subarray"), index #1=w699, new element #2=u16 1 ("new element/subarray"), index #2=w698) -> (w701:u16[])
                }
                frame 2 {
                }
                frame 3 {
                  n413 = Replace Array Subset(array=w707, new element #1=u16 100 ("new element/subarray"), index #1=w706, new element #2=u16 1 ("new element/subarray"), index #2=w705) -> (w708:u16[])
                }
                frame 4 {
                  w709 = u16 0 ("new element/subarray")
                  n414 = Replace Array Subset(array=w712, new element #1=w709, index #1=w711, new element #2=w709, index #2=w710) -> (w713:u16[])
                }
                frame 5 {
                }
                frame 6 {
                  n415 = Replace Array Subset(array=w717, new element=u16 0 ("new element/subarray"), index=w716) -> (w718:u16[])
                }
                frame 7 {
                  n416 = local write "RewCalib_Trig_L"(FALSE ("RewCalib_Trig_L")) -> ()
                  n417 = Replace Array Subset(array=w722, new element=u16 0 ("new element/subarray"), index=w721) -> (w723:u16[])
                }
              }
              n418 = case shown="7" w637 {
                tunnel: w650 -> [w666 w671 w673 w678 w683 w685 w688 w693]
                tunnel: [w666 w672 w673 w679 w684 w685 w689 w694] -> w649
                tunnel: w633 -> [_ w669 _ w676 w681 _ w687 w692]
                tunnel: w636 -> [_ w670 _ w677 w682 _ _ _]
                frame 0, Default {
                }
                frame 1 {
                  n419 = Replace Array Subset(array=w671, new element #1=u16 100 ("new element/subarray"), index #1=w670, new element #2=u16 1 ("new element/subarray"), index #2=w669) -> (w672:u16[])
                }
                frame 2 {
                }
                frame 3 {
                  n420 = Replace Array Subset(array=w678, new element #1=u16 100 ("new element/subarray"), index #1=w677, new element #2=u16 1 ("new element/subarray"), index #2=w676) -> (w679:u16[])
                }
                frame 4 {
                  w680 = u16 0 ("new element/subarray")
                  n421 = Replace Array Subset(array=w683, new element #1=w680, index #1=w682, new element #2=w680, index #2=w681) -> (w684:u16[])
                }
                frame 5 {
                }
                frame 6 {
                  n422 = Replace Array Subset(array=w688, new element=u16 0 ("new element/subarray"), index=w687) -> (w689:u16[])
                }
                frame 7 {
                  n423 = local write "RewCalib_Trig_R"(FALSE ("RewCalib_Trig_L")) -> ()
                  n424 = Replace Array Subset(array=w693, new element=u16 0 ("new element/subarray"), index=w692) -> (w694:u16[])
                }
              }
            }
            frame "DispenseWater_pre" {
              w730 = u16 0 ("t")
              w773 = u16 0 ("new element/subarray")
              # "just trust me on this one"
              # "RewCalib\nOnOff"
              # "RewCalib\nOnOff"
              # "nCycle"
              # "Solenoid__R"
              # "Tdelay"
              # "delay"
              # "nCycle"
              # "Solenoid__L"
              # "Tdelay"
              # "delay"
              # "Solenoid__R"
              # "count"
              # "Solenoid_Tcycle_R"
              # "Solenoid_Tcycle_L"
              # "Solenoid__L"
              # "count"
              n425 = call "myRIO_BRig_RT_dataMTrig_Solenoid_RewCalib_OnOff__L.vi"() -> ("output_Solenoid_RewCalib_OnOff__L"=w737:i32)  [unwired: 11 in]
              n426 = call "myRIO_BRig_RT_dataMTrig_Solenoid_N__L.vi"() -> ("output_Solenoid_N__L"=w728:i32)  [unwired: 11 in]
              n427 = call "myRIO_BRig_RT_dataMTrig_Solenoid_delay__L.vi"() -> ("output_Solenoid_delay__L"=w771:i32)  [unwired: 11 in]
              n428 = call "myRIO_BRig_RT_dataMTrig_Solenoid_Tdelay__L.vi"() -> ("output_Solenoid_Tdelay__L"=w770:i32)  [unwired: 11 in]
              n429 = call "myRIO_BRig_RT_dataMTrig_Solenoid_N__R.vi"() -> ("output_Solenoid_N__R"=w726:i32)  [unwired: 11 in]
              n430 = call "myRIO_BRig_RT_dataMTrig_Solenoid_delay__R.vi"() -> ("output_Solenoid_delay__R"=w760:i32)  [unwired: 11 in]
              n431 = call "myRIO_BRig_RT_dataMTrig_Solenoid_Tdelay__R.vi"() -> ("output_Solenoid_Tdelay__R"=w759:i32)  [unwired: 11 in]
              n432 = call "myRIO_BRig_RT_dataMTrig_Solenoid_RewCalib_OnOff__R.vi"() -> ("output_Solenoid_RewCalib_OnOff__R"=w733:i32)  [unwired: 11 in]
              n433 = Index Array(array=w772, index #1=w728, index #2=w771, index #3=w770, index #4=w726, index #5=w760, index #6=w759, index #7=w737, index #8=w733) -> (element #1=w729:u16, element #2=w769:u16, element #3=w764:u16, element #4=w732:u16, element #5=w754:u16, element #6=w753:u16, element #7=w738:u16, element #8=w735:u16)
              n434 = Equal To 0?(x=w769) -> (x = 0?=w768:bool)
              n435 = Equal To 0?(x=w754) -> (x = 0?=w758:bool)
              n436 = local read "RewCalib_Trig_L"() -> (w749:bool)
              n437 = local read "RewCalib_Trig_R"() -> (w744:bool)
              n438 = Not Equal To 0?(x=w729) -> (x != 0?=w767:bool)
              n439 = Not Equal To 0?(x=w732) -> (x != 0?=w757:bool)
              n440 = local read "MTrig_Solenoid_Tcycle__L"() -> (w766:u16)
              n441 = local read "MTrig_Solenoid_Tcycle__R"() -> (w752:u16)
              n442 = Not Equal To 0?(x=w738) -> (x != 0?=w748:bool)
              n443 = Not Equal To 0?(x=w735) -> (x != 0?=w746:bool)
              n444 = Not(x=w749) -> (.not. x?=w747:bool)
              n445 = Not(x=w744) -> (.not. x?=w745:bool)
              n446 = And(x=w748, y=w747) -> (x .and. y?=w743:bool)
              n447 = And(x=w746, y=w745) -> (x .and. y?=w742:bool)
              n448 = call "myRIO_BRig_RT_dataMTrig_Solenoid_c__L.vi"() -> ("output_Solenoid_c__L"=w775:i32)  [unwired: 11 in]
              n449 = call "myRIO_BRig_RT_dataMTrig_Solenoid_c__R.vi"() -> ("output_Solenoid_c__R"=w774:i32)  [unwired: 11 in]
              n450 = Select(t=w766, s=w767, f=u16 0) -> (s? t:f=w763:u16)
              n451 = Or(x=w743, y=w742) -> (x .or. y?=w731:bool)
              n452 = Select(t=w752, s=w757, f=u16 0) -> (s? t:f=w755:u16)
              n453 = Select(t=w763, s=w768, f=w764) -> (s? t:f=w761:u16)
              n454 = Select(t=w755, s=w758, f=w753) -> (s? t:f=w750:u16)
              n455 = call "myRIO_BRig_RT_dataMTrig_Solenoid_Tcycle__L.vi"() -> ("output_Solenoid_Tcycle__L"=w762:i32)  [unwired: 11 in]
              n456 = call "myRIO_BRig_RT_dataMTrig_Solenoid_Tcycle__R.vi"() -> ("output_Solenoid_Tcycle__R"=w751:i32)  [unwired: 11 in]
              n457 = Select(t=w730, s=w731, f=w729) -> (s? t:f=w727:u16)
              n458 = Select(t=w730, s=w731, f=w732) -> (s? t:f=w725:u16)
              n459 = Select(t=myRIO_BRig_RT__Case_NonExp_stateList."Idle" ("Enum"), s=w731, f=myRIO_BRig_RT__Case_NonExp_stateList."DispenseWater" ("Enum")) -> (s? t:f=w739:T1)
              n460 = Select(t=w730, s=w731, f=w738) -> (s? t:f=w736:u16)
              n461 = Select(t=w730, s=w731, f=w735) -> (s? t:f=w734:u16)
              n462 = Replace Array Subset(array=w772, new element #1=w773, index #1=w775, new element #2=w773, index #2=w774, new element #3=w761, index #3=w762, new element #4=w750, index #4=w751, new element #5=w736, index #5=w737, new element #6=w734, index #6=w733, new element #7=w727, index #7=w728, new element #8=w725, index #8=w726) -> (w776:u16[])
            }
            frame "DispenseWater" {
              # "D"
              # "C"
              # "B"
              # "A"
              # "(A) Add COUNT and INCREMENT\n(B) Is (A) smaller than Tcycle?\n(C) Are we dispensing water or in the delay phase?\n(D) If (A) is smaller than Tcycle   AND   if we are dispensing water\n      then send TRUE to solenoid"
              # "delay"
              # "Tcycle"
              # "Solenoid__R"
              # "count"
              # "delay"
              # "Tcycle"
              # "Solenoid__L"
              # "count"
              n463 = To Unsigned Word Integer(number=w804) -> (unsigned 16bit integer=w786:u16)
              n464 = call "myRIO_BRig_RT_dataMTrig_Solenoid_delay__R.vi"() -> ("output_Solenoid_delay__R"=w790:i32)  [unwired: 11 in]
              n465 = call "myRIO_BRig_RT_dataMTrig_Solenoid_c__R.vi"() -> ("output_Solenoid_c__R"=w789:i32)  [unwired: 11 in]
              n466 = call "myRIO_BRig_RT_dataMTrig_Solenoid_Tcycle__R.vi"() -> ("output_Solenoid_Tcycle__R"=w791:i32)  [unwired: 11 in]
              n467 = call "myRIO_BRig_RT_dataMTrig_Solenoid_delay__L.vi"() -> ("output_Solenoid_delay__L"=w806:i32)  [unwired: 11 in]
              n468 = call "myRIO_BRig_RT_dataMTrig_Solenoid_c__L.vi"() -> ("output_Solenoid_c__L"=w798:i32)  [unwired: 11 in]
              n469 = call "myRIO_BRig_RT_dataMTrig_Solenoid_Tcycle__L.vi"() -> ("output_Solenoid_Tcycle__L"=w807:i32)  [unwired: 11 in]
              n470 = Index Array(array=w800, index #1=w798, index #2=w807, index #3=w806, index #4=w789, index #5=w791, index #6=w790) -> (element #1=w805:u16, element #2=w795:u16, element #3=w803:u16, element #4=w785:u16, element #5=w782:u16, element #6=w781:u16)
              n471 = Add(x=w805, y=w786) -> (x+y=w796:u16)
              n472 = Add(x=w785, y=w786) -> (x+y=w787:u16)
              n473 = Less?(x=w796, y=w795) -> (x < y?=w779:bool)
              n474 = Equal To 0?(x=w803) -> (x = 0?=w802:bool)
              n475 = Less?(x=w787, y=w782) -> (x < y?=w780:bool)
              n476 = Equal To 0?(x=w781) -> (x = 0?=w788:bool)
              n477 = And(x=w779, y=w802) -> (x .and. y?=w801:bool)
              n478 = Or(x=w779, y=w780) -> (x .or. y?=w778:bool)
              n479 = And(x=w780, y=w788) -> (x .and. y?=w783:bool)
              n480 = Select(t=w796, s=w779, f=w795) -> (s? t:f=w797:u16)
              n481 = Select(t=w787, s=w780, f=w782) -> (s? t:f=w784:u16)
              n482 = Replace Array Subset(array=w800, new element #1=w797, index #1=w798, new element #2=w784, index #2=w789) -> (w799:u16[])
              n483 = Select(t=w794, s=w778, f=myRIO_BRig_RT__Case_NonExp_stateList."DispenseWater_post" ("Enum")) -> (s? t:f=w792:T1)
            }
            frame "DispenseWater_post" {
              # "nCycle"
              # "delay"
              # "Solenoid__R"
              # "nCycle"
              # "delay"
              # "Solenoid__L"
              n484 = call "myRIO_BRig_RT_dataMTrig_Solenoid_N__L.vi"() -> ("output_Solenoid_N__L"=w825:i32)  [unwired: 11 in]
              n485 = call "myRIO_BRig_RT_dataMTrig_Solenoid_delay__L.vi"() -> ("output_Solenoid_delay__L"=w824:i32)  [unwired: 11 in]
              n486 = call "myRIO_BRig_RT_dataMTrig_Solenoid_N__R.vi"() -> ("output_Solenoid_N__R"=w821:i32)  [unwired: 11 in]
              n487 = call "myRIO_BRig_RT_dataMTrig_Solenoid_delay__R.vi"() -> ("output_Solenoid_delay__R"=w820:i32)  [unwired: 11 in]
              n488 = Index Array(array=w827, index #1=w825, index #2=w824, index #3=w821, index #4=w820) -> (element #1=w829:u16, element #2=w828:u16, element #3=w812:u16, element #4=w814:u16)
              n489 = Not Equal To 0?(x=w829) -> (x != 0?=w830:bool)
              n490 = Not Equal To 0?(x=w812) -> (x != 0?=w813:bool)
              n491 = case shown="True" w813 {
                selector: w813 -> [_ w834]
                tunnel: w812 -> [w832 w840]
                tunnel: w814 -> [_ w841]
                tunnel: [w832 w838] -> w811
                tunnel: [u16 0 w837] -> w810
                tunnel: [_ w834] -> w809
                frame False {
                }
                frame True {
                  n492 = Equal To 0?(x=w841) -> (x = 0?=w833:bool)
                  n493 = Decrement(x=w840) -> (x-1=w839:u16)
                  n494 = Select(t=w839, s=w833, f=w840) -> (s? t:f=w838:u16)
                  n495 = Select(t=u16 1, s=w833, f=u16 0) -> (s? t:f=w837:u16)
                }
              }
              n496 = case shown="True" w830 {
                selector: w830 -> [_ w845]
                tunnel: w829 -> [w843 w851]
                tunnel: w828 -> [_ w852]
                tunnel: [w843 w849] -> w823
                tunnel: [u16 0 w848] -> w822
                tunnel: [_ w845] -> w819
                frame False {
                }
                frame True {
                  n497 = Equal To 0?(x=w852) -> (x = 0?=w844:bool)
                  n498 = Decrement(x=w851) -> (x-1=w850:u16)
                  n499 = Select(t=w850, s=w844, f=w851) -> (s? t:f=w849:u16)
                  n500 = Select(t=u16 1, s=w844, f=u16 0) -> (s? t:f=w848:u16)
                }
              }
              n501 = Or(x=w819, y=w809) -> (x .or. y?=w818:bool)
              n502 = Replace Array Subset(array=w827, new element #1=w823, index #1=w825, new element #2=w822, index #2=w824, new element #3=w811, index #3=w821, new element #4=w810, index #4=w820) -> (w826:u16[])
              n503 = Select(t=myRIO_BRig_RT__Case_NonExp_stateList."DispenseWater_pre" ("Enum"), s=w818, f=myRIO_BRig_RT__Case_NonExp_stateList."Idle" ("Enum")) -> (s? t:f=w815:T1)
            }
            frame "TestConnection" {
              n504 = local read "Host Password"() -> (w859:string)
              n505 = local read "Host UserName"() -> (w860:string)
              n506 = call "myRIO_BRig_RT_comm_webdav_testConnect.vi"("input_password"=w859, "input_username"=w860) -> ("output_Iconnected"=w857:bool)  [unwired: 9 in]
              n507 = Select(t="Connection accepted!" ("message"), s=w857, f="Error!") -> (s? t:f=w855:string)
              n508 = One Button Dialog(message=w855) -> ()  [unwired: 1 in, 1 out]
            }
            frame "SendData" {
              n509 = local read "Data Set Prefix"() -> (w862:string)
              n510 = local read "Host Password"() -> (w863:string)
              n511 = local read "Host UserName"() -> (w864:string)
              n512 = call "myRIO_BRig_RT_comm_webdav_sendData_all.vi"("Host Filename Prefix"=w862, "Host Password"=w863, "Host UserName"=w864) -> ()  [unwired: 9 in]
            }
            frame "Get_FPGA_count_per_ms" {
              n513 = case shown="False" w878 {
                selector: w878 -> [w881 _]
                tunnel: w876 -> [_ w894]
                tunnel: [w885 w894] -> w875
                tunnel: w874 -> [w884 w892]
                tunnel: w873 -> [w883 w891]
                tunnel: [w882 w889] -> w872
                tunnel: [w881 w888] -> w871
                frame False {
                  n514 = Get Date/Time In Seconds() -> (seconds since 1Jan1904=w886:timestamp)
                  n515 = xnode "Read/Write Control"("FPGA VI Reference In"=w884, "error in"=w883, "timeTrial_trig"=TRUE ("timeTrial")) -> ("error out"=w882:errorcluster)  [unwired: 1 out]
                  n516 = To Double Precision Float(number=w886) -> (double precision float=w885:dbl)
                  n517 = local write "get_countPerMS"(w881) -> ()
                }
                frame True {
                  w890 = 1.0
                  n518 = Get Date/Time In Seconds() -> (seconds since 1Jan1904=w895:timestamp)
                  n519 = To Double Precision Float(number=w895) -> (double precision float=w896:dbl)
                  n520 = Subtract(x=w896, y=w894) -> (x-y=w893:dbl)
                  n521 = Less Or Equal?(x=w890, y=w893) -> (x <= y?=w888:bool)
                  n522 = case shown="True" w888 {
                    tunnel: w892 -> [_ w909]
                    tunnel: w891 -> [w897 w908]
                    tunnel: w890 -> [_ w899]
                    tunnel: [w897 w898] -> w889
                    frame False {
                    }
                    frame True {
                      n523 = xnode "Read/Write Control"("FPGA VI Reference In"=w909, "error in"=w908) -> ("FPGA VI Reference Out"=w906:refnum<k20>, "error out"=w905:errorcluster, "timeTrial_count"=w900:u32)
                      n524 = Multiply(x=w899, y=1000.0) -> (x*y=w903:dbl)
                      n525 = To Double Precision Float(number=w900) -> (double precision float=w902:dbl)
                      n526 = Divide(x=w902, y=w903) -> (x/y=w904:dbl)
                      n527 = local write "FPGA_count2ms"(w904) -> ()
                      n528 = xnode "Read/Write Control"("FPGA VI Reference In"=w906, "error in"=w905, "timeTrial_trig"=FALSE ("timeTrial")) -> ("error out"=w898:errorcluster)  [unwired: 1 out]
                    }
                  }
                }
              }
              "error out 5" <- w872
              n529 = Select(t=myRIO_BRig_RT__Case_NonExp_stateList."Idle" ("Enum"), s=w871, f=w869) -> (s? t:f=w868:T1)
            }
            frame "End" {
            }
          }
          n530 = local read "MTrig_Audio_trig__R"() -> (w84:bool)
          n531 = local read "MTrig_Audio_trig__L"() -> (w85:bool)
          n532 = local read "MTrig_Laser_trig"() -> (w83:bool)
          n533 = Compound Arithmetic op=OR(w85, w84, w83) -> (w82:bool)
          n534 = local read "START"() -> (w118:bool)
          n535 = local read "STOP_abort"() -> (w117:bool)
          n536 = case shown="True" w82 {
            frame False {
            }
            frame True {
              w134 = FALSE
              n537 = local write "MTrig_Audio_trig__R"(w134) -> ()
              n538 = local write "MTrig_Audio_trig__L"(w134) -> ()
              n539 = local write "MTrig_Laser_trig"(w134) -> ()
            }
          }
          n540 = call "myRIO_BRig_RT_dataMTrig_main__v2.vi"("input_dataMTrig"=w121, "input_Audio_trig_L"=w85, "input_Audio_trig_R"=w84, "input_Laser_trig"=w83) -> ("output_dataMTrig"=w120:u16[], "output_Audio_L"=w102:bool, "output_Audio_R"=w113:bool, "output_Laser"=w105:bool)  [unwired: 12 in]
          n541 = Or(x=w118, y=w117) -> (x .or. y?=w116:bool)
          n542 = Select(t=myRIO_BRig_RT__Case_NonExp_stateList."End" ("Enum"), s=w116, f=w115) -> (s? t:f=w114:T1)
          n543 = xnode "Read/Write Control"("FPGA VI Reference In"=w91, "error in"=w90, "A1_SR"=w122, "A3_SL"=w123, "audioTrigger_L"=w102, "audioTrigger_R"=w113, "LR_reward_Event_l1"="laserResponse_reward_LED", "LR_wrong_Event_l1"="laserResponse_wrong_LED", "LR_reward_Laser_l1"="laserResponse_reward", "LR_wrong_Laser_l1"="laserResponse_wrong", "SelectionState"="SelectionState", "ignoreWrong"="ignoreWrong", "Left(F)_or_Right(T)"="Left(F)_or_Right(T)", "LC_Laser_l1"=w105) -> ("FPGA VI Reference Out"=w128:refnum<k20>, "error out"=w127:errorcluster, "SelectReward"=→"SelectReward":bool, "SelectWrong"=→"SelectWrong":bool)
          n544 = node-c288() -> ()  [unwired: 1 in, 1 out]
          "cState_NonExp" <- w126
        }
        n545 = node-c288(w70) -> ()  [unwired: 1 out]
        n546 = flat-sequence {
          tunnel: w63 -> [w81]
          tunnel: [w81] -> w62
          tunnel: w61 -> [w80]
          tunnel: [w80] -> w60
          frame #0 {
            w79 = FALSE
            n547 = local write "STOP_endBlock"(w79) -> ()
            n548 = local write "STOP_endTrial"(w79) -> ()
          }
        }
      }
      frame True {
        w922 = u16 0
        w941 = u8 0
        w942 = u16 0 ("idxDataBlock")
        w944 = u16 100 ("new element/subarray")
        w945 = u16 100 ("new element/subarray")
        w965 = T6 refnum items=["Session NI_WebDAV"] ("output_hSession")
        w974 = FALSE
        w975 = u16 0
        w929 = FALSE
        # "dummyState counter"
        # "audio__L\naudio__R"
        # "Audio params"
        # "nRewards"
        # "idxDataBlock"
        # "Solenoid_Tdelay_R"
        # "Solenoid_Tdelay_L"
        # "RewCalib_N__R"
        # "RewCalib_N__L"
        # "Save dataLick to file\nSend file to Host\nSave dataMTrig\nSend file to Host\nDisconnect"
        # "dataTrial"
        # "dataTrial"
        # "Solenoid_Tcycle_R"
        # "Solenoid_Tcycle_L"
        # "Laser_Tcycle"
        # "Audio_Tcycle_R"
        # "Audio_Tcycle_L"
        # "dataLick"
        # "dataLC"
        # "dataLC"
        # "dataBlock"
        # "dataBlock"
        # "dataMTrig"
        # "dataMTrig"
        # "dataExp"
        # "dataCurrent"
        # "dataExp"
        # "dataCurrent"
        # "spout"
        # "state"
        n549 = call "myRIO_BRig_RT_dataMTrig_Solenoid_Tcycle__L.vi"() -> ("output_Solenoid_Tcycle__L"=w971:i32)  [unwired: 11 in]
        n550 = call "myRIO_BRig_RT_dataMTrig_Solenoid_Tcycle__R.vi"() -> ("output_Solenoid_Tcycle__R"=w970:i32)  [unwired: 11 in]
        n551 = call "myRIO_BRig_RT_dataMTrig_Audio_Tcycle__L.vi"() -> ("output_Audio_Tcycle__L"=w969:i32)  [unwired: 11 in]
        n552 = call "myRIO_BRig_RT_dataMTrig_Audio_Tcycle__R.vi"() -> ("output_Audio_Tcycle__R"=w968:i32)  [unwired: 11 in]
        n553 = call "myRIO_BRig_RT_dataMTrig_Laser_Tcycle.vi"() -> ("output_Laser_Tcycle"=w967:i32)  [unwired: 11 in]
        n554 = local read "MTrig_Solenoid_Tcycle__L"() -> (w950:u16)
        n555 = local read "MTrig_Solenoid_Tcycle__R"() -> (w949:u16)
        n556 = local read "Tcycle_Reward_L"() -> (w946:u16)
        n557 = local read "Tcycle_Reward_R"() -> (w947:u16)
        n558 = local read "MTrig_Laser_Tcycle"() -> (w948:u16)
        n559 = call "myRIO_BRig_RT_dataMTrig_Solenoid_RewCalib_nCycle__L.vi"() -> ("output_Solenoid_RewCalib_nCycle__L"=w953:i32)  [unwired: 11 in]
        n560 = call "myRIO_BRig_RT_dataMTrig_Solenoid_Tdelay__L.vi"() -> ("output_Solenoid_Tdelay__L"=w955:i32)  [unwired: 11 in]
        n561 = call "myRIO_BRig_RT_dataMTrig_Solenoid_RewCalib_nCycle__R.vi"() -> ("output_Solenoid_RewCalib_nCycle__R"=w954:i32)  [unwired: 11 in]
        n562 = call "myRIO_BRig_RT_dataMTrig_Solenoid_Tdelay__R.vi"() -> ("output_Solenoid_Tdelay__R"=w956:i32)  [unwired: 11 in]
        n563 = case shown="False" w933 {
          selector: w933 -> [_ w997]
          tunnel: w932 -> [w994 w999]
          tunnel: [w995 w999] -> w927
          tunnel: w931 -> [_ w998]
          tunnel: [w996 w998] -> w928
          tunnel: [w993 w997] -> w926
          frame False {
            n564 = call "myRIO__TCP_connect_forWriting.vi"("input_error"=w994) -> ("output_error"=w995:errorcluster, "output_connected"=w993:bool, "output_hTCP"=w996:refnum<k5>)  [unwired: 8 in]
          }
          frame True {
          }
        }
        n565 = call "myRIO_BRig_RT_dataLick_init.vi"() -> ("output_dataLick"=w977:u16[][])  [unwired: 11 in]
        n566 = call "myRIO_BRig_RT_dataCurrent_init.vi"() -> ("output_dataCurrent"=w984:u16[])  [unwired: 11 in]
        n567 = call "myRIO_BRig_RT_dataExp_init.vi"() -> ("output_dataExp"=w983:u16[])  [unwired: 11 in]
        n568 = call "myRIO_BRig_RT_dataMTrig_init.vi"() -> ("output_dataMTrig"=w973:u16[])  [unwired: 5 in]
        n569 = call "myRIO_BRig_RT_dataLC_init.vi"() -> ("output_dataLC"=w981:u16[])  [unwired: 11 in]
        n570 = call "myRIO_BRig_RT_dataBlock_init.vi"() -> ("output_dataBlock"=w982:u16[][])  [unwired: 11 in]
        n571 = call "myRIO_BRig_RT_dataTrial_init.vi"() -> ("output_dataTrial"=w966:u16[][])  [unwired: 11 in]
        n572 = local write "I_connect_TCP"(w926) -> ()
        n573 = Replace Array Subset(array=w973, new element #1=w945, index #1=w953, new element #2=w945, index #2=w954, new element #3=w944, index #3=w955, new element #4=w944, index #4=w956, new element #5=w950, index #5=w971, new element #6=w949, index #6=w970, new element #7=w946, index #7=w969, new element #8=w947, index #8=w968, new element #9=w948, index #9=w967) -> (w972:u16[])
        n574 = call "myRIO_BRig_RT_dataAnalog_init.vi"() -> ("output_dataAnalog"=w938:u16[][])  [unwired: 11 in]
        n575 = call "myRIO_BRig_RT_TCP__start_exp.vi"("input_hTCP"=w928, "input_I_connected_TCP"=w926, "input_error"=w927) -> ("output_hTCP"=w925:refnum<k5>, "output_error"=w924:errorcluster)  [unwired: 11 in]
        n576 = Get Date/Time In Seconds() -> (seconds since 1Jan1904=w952:timestamp)
        n577 = call "myRIO_BRig_RT_arrTrig_init.vi"() -> ("output_arrTrig"=w921:bool[])  [unwired: 11 in]
        n578 = To Double Precision Float(number=w952) -> (double precision float=w951:dbl)
        n579 = node-c288() -> (w992:T3)  [unwired: 4 in]
        n580 = timed-loop {
          timing: w992 -> [_]
          timing-out: [_] -> w991
          shift-right: [w1123] -> _
          shift-left: myRIO_BRig_RT__Case_Exp_stateList."Start1" ("Enum") -> [w1058]
          shift-right: [w1055] -> _
          shift-left: enum16{"Left", "Right"}."Left" -> [w1172]
          tunnel: w920 -> [w1170]
          tunnel: w919 -> [w1169]
          shift-right: [w1164] -> _
          shift-left: w989 -> [w1168]
          shift-right: [w1163] -> _
          shift-left: w988 -> [w1167]
          tunnel: [w1146] -> w986
          tunnel: [w1147] -> w987
          shift-right: [w1148] -> w957
          shift-left: w984 -> [w1115]
          shift-right: [w1162] -> _
          shift-left: w983 -> [w1112]
          shift-right: [w1135] -> w961
          shift-left: w972 -> [w1136]
          shift-right: [w1160] -> _
          shift-left: w982 -> [w1161]
          shift-right: [w1158] -> _
          shift-left: w981 -> [w1159]
          shift-right: [w1150] -> w963
          shift-left: w977 -> [w1151]
          shift-right: [w1137] -> _
          shift-left: w975 -> [w1145]
          shift-right: [w1109] -> _
          shift-left: w941 -> [w1144]
          shift-right: [w1138] -> _
          shift-left: w975 -> [w1143]
          shift-right: [w1139] -> _
          shift-left: w941 -> [w1142]
          shift-right: [w1110] -> _
          shift-left: w974 -> [w1140]
          shift-right: [w1111] -> _
          shift-left: w974 -> [w1141]
          shift-right: [w1121] -> _
          shift-left: w966 -> [w1122]
          shift-right: [w1120] -> w959
          shift-left: w965 -> [w1118]
          shift-right: [w1119] -> w960
          shift-left: FALSE ("output_Iconnected") -> [w1117]
          tunnel: "Data Set Prefix" -> [w1116]
          tunnel: [w1116] -> w958
          shift-right: [w1094] -> _
          shift-left: w929 -> [w1114]
          tunnel: w951 -> [w1113]
          shift-right: [w1107] -> _
          shift-left: 0 ("idxDataBlock") -> [w1108]
          shift-right: [w1104] -> _
          shift-left: w942 -> [w1106]
          shift-right: [w1103] -> _
          shift-left: w942 -> [w1105]
          shift-right: [w1093] -> _
          shift-left: w929 -> [w1099]
          shift-right: [w1096] -> _
          shift-left: w929 -> [w1098]
          shift-right: [w1095] -> _
          shift-left: w929 -> [w1097]
          shift-right: [w1081] -> w936
          shift-left: 0 -> [w1065]
          shift-right: [w1056] -> _
          shift-left: w922 -> [w1076]
          shift-right: [w1057] -> _
          shift-left: w922 -> [w1072]
          shift-right: [w1085] -> _
          shift-left: FALSE -> [w1085]
          shift-right: [w1071] -> _
          shift-left: w922 -> [w1079]
          shift-right: [w1082] -> w937
          shift-left: w938 -> [w1083]
          tunnel: w925 -> [w1070]
          tunnel: [w1069] -> w935
          tunnel: w926 -> [w1066]
          tunnel: [w1066] -> w934
          tunnel: w924 -> [w1068]
          tunnel: [w1067] -> w930
          shift-right: [w1061] -> _
          shift-left: w929 -> [w1062]
          shift-right: [w1059] -> _
          shift-left: w929 -> [w1060]
          shift-right: [w1053] -> _
          shift-left: u16 0 -> [w1054]
          shift-right: [w1051] -> _
          shift-left: w922 -> [w1052]
          shift-right: [w1048] -> _
          shift-left: w921 -> [w1049]
          stop <- w1157 stop-if-true
          # "Sel"
          # "Sel"
          # "Cue1"
          # "Cue1"
          # "ENL1"
          # "ENL1"
          # "iState"
          # "dataAnalog"
          # "index"
          # "iEvent"
          # "iBlock"
          # "iTrial"
          # "Laser"
          # "Audio R"
          # "Audio L"
          # "Solenoid R"
          # "Solenoid L"
          # "manual triggering"
          # "dataTrial"
          # "dataBlock"
          # "nRewards"
          # "dataExp"
          # "dataCurrent"
          # "audio__L\naudio__R"
          # "time stamp"
          # "Audio params"
          # "nRewards"
          # "idxDataBlock"
          # "idxDataBlock"
          # "activate"
          # "audio__L\naudio__R"
          # "amp__R\nfreq__R"
          # "amp__L\nfreq__L"
          # "dataLC"
          # "solenoid__R"
          # "solenoid__L"
          # "Did a lick occur?"
          # "Update lick counter"
          # "spout"
          # "spout"
          # "state"
          # "state"
          n581 = node-c288() -> ()  [unwired: 1 in, 1 out]
          n582 = local read "MTrig_Solenoid_trig__L"() -> (w1133:bool)
          n583 = local read "MTrig_Solenoid_trig__R"() -> (w1132:bool)
          n584 = local read "MTrig_Audio_trig__L"() -> (w1131:bool)
          n585 = local read "MTrig_Audio_trig__R"() -> (w1130:bool)
          n586 = xnode "Read/Write Control"("FPGA VI Reference In"=w1170, "error in"=w1169) -> ("FPGA VI Reference Out"=w1102:refnum<k20>, "error out"=w1101:errorcluster, "A2_LickL"=w1164:u32, "A4_LickR"=w1163:u32)
          "A2" <- w1164
          "A4" <- w1163
          n587 = local read "MTrig_Laser_trig"() -> (w1129:bool)
          n588 = Greater?(x=w1164, y=w1168) -> (0:w1166:bool)
          n589 = Greater?(x=w1163, y=w1167) -> (0:w1165:bool)
          n590 = Or(x=w1166, y=w1165) -> (x .or. y?=w1171:bool)
          n591 = call "myRIO_BRig_RT_dataMTrig_main.vi"("input_dataMTrig"=w1136, "input_Solenoid_trig_L"=w1133, "input_Solenoid_trig_R"=w1132, "input_Audio_trig_L"=w1131, "input_Audio_trig_R"=w1130, "input_Laser_trig"=w1129) -> ("output_Laser"=w1091:bool, "output_dataMTrig"=w1135:u16[], "output_Solenoid_L"=w1047:bool, "output_Solenoid_R"=w1125:bool, "output_Audio_L"=w1127:bool, "output_Audio_R"=w1128:bool)  [unwired: 8 in]
          n592 = Compound Arithmetic op=OR(w1133, w1132, w1131, w1130, w1129) -> (w1134:bool)
          n593 = case shown="True" w1134 {
            frame False {
            }
            frame True {
              w1173 = FALSE
              n594 = local write "MTrig_Solenoid_trig__L"(w1173) -> ()
              n595 = local write "MTrig_Solenoid_trig__R"(w1173) -> ()
              n596 = local write "MTrig_Audio_trig__L"(w1173) -> ()
              n597 = local write "MTrig_Audio_trig__R"(w1173) -> ()
              n598 = local write "MTrig_Laser_trig"(w1173) -> ()
            }
          }
          n599 = case shown="\"setSettings_Laser\"" w1058 {
            selector: w1058 -> [_ _ _ _ _ _ _ _ _ _ _ _ _ _ _ _ _ _ _ _ _ _ _ _ _ _ w2250 _ w2317 _ _ _ _ _ w2468 _ w2547 _ _ _ _ _ w2702 _ w2776 _ w2840 _ w2884 _ _ w2954 _ _ _ _ _ w3125 _ _ _ _ _ _ _ _ _ _ _ _ w3406 w3439]
            tunnel: [myRIO_BRig_RT__Case_Exp_stateList."Start2" ("Enum") myRIO_BRig_RT__Case_Exp_stateList."Start3" ("Enum") myRIO_BRig_RT__Case_Exp_stateList."saveSettings1" ("Enum") myRIO_BRig_RT__Case_Exp_stateList."saveSettings2" ("Enum") myRIO_BRig_RT__Case_Exp_stateList."saveSettings3" ("Enum") myRIO_BRig_RT__Case_Exp_stateList."saveSettings4" ("Enum") myRIO_BRig_RT__Case_Exp_stateList."saveSettings_LC_ENL_l1" ("Enum") myRIO_BRig_RT__Case_Exp_stateList."saveSettings_LC_ENL_l2" ("Enum") myRIO_BRig_RT__Case_Exp_stateList."saveSettings_LC_Cue_l1" ("Enum") myRIO_BRig_RT__Case_Exp_stateList."saveSettings_LC_Cue_l2" ("Enum") myRIO_BRig_RT__Case_Exp_stateList."saveSettings6_LC_l1_Other" ("Enum") myRIO_BRig_RT__Case_Exp_stateList."SaveSettings6_LC_l2_Other" ("Enum") myRIO_BRig_RT__Case_Exp_stateList."setSettings_Audio" ("Enum") myRIO_BRig_RT__Case_Exp_stateList."setSettings_Laser" ("Enum") myRIO_BRig_RT__Case_Exp_stateList."commConnect" ("Enum") w1944 myRIO_BRig_RT__Case_Exp_stateList."initTrial" ("Enum") w1989 myRIO_BRig_RT__Case_Exp_stateList."initTrial3" ("Enum") myRIO_BRig_RT__Case_Exp_stateList."initTrial_LC_ENL1" ("Enum") myRIO_BRig_RT__Case_Exp_stateList."ENL1_pre" ("Enum") myRIO_BRig_RT__Case_Exp_stateList."initTrial_LC_Cue1" ("Enum") myRIO_BRig_RT__Case_Exp_stateList."initTrial_LC_Cue1_2" ("Enum") myRIO_BRig_RT__Case_Exp_stateList."initTrial_LC_Sel" ("Enum") myRIO_BRig_RT__Case_Exp_stateList."initTrial4" ("Enum") w2209 w2247 myRIO_BRig_RT__Case_Exp_stateList."ENL1Penalty" ("Enum") w2318 myRIO_BRig_RT__Case_Exp_stateList."endExp" ("Enum") myRIO_BRig_RT__Case_Exp_stateList."endExp" ("Enum") myRIO_BRig_RT__Case_Exp_stateList."endExp" ("Enum") myRIO_BRig_RT__Case_Exp_stateList."endExp" ("Enum") w2421 w2467 myRIO_BRig_RT__Case_Exp_stateList."Cue1Penalty" ("Enum") w2545 myRIO_BRig_RT__Case_Exp_stateList."endExp" ("Enum") myRIO_BRig_RT__Case_Exp_stateList."endExp" ("Enum") myRIO_BRig_RT__Case_Exp_stateList."endExp" ("Enum") myRIO_BRig_RT__Case_Exp_stateList."endExp" ("Enum") w2642 w2708 myRIO_BRig_RT__Case_Exp_stateList."SelectReward" ("Enum") w2777 myRIO_BRig_RT__Case_Exp_stateList."SelectRewardPost" ("Enum") w2841 myRIO_BRig_RT__Case_Exp_stateList."SelectWrong" ("Enum") w2880 myRIO_BRig_RT__Case_Exp_stateList."endTrial1" ("Enum") myRIO_BRig_RT__Case_Exp_stateList."SelectTimeout" ("Enum") w2956 myRIO_BRig_RT__Case_Exp_stateList."endTrial1" ("Enum") myRIO_BRig_RT__Case_Exp_stateList."endTrial2" ("Enum") myRIO_BRig_RT__Case_Exp_stateList."endTrial3" ("Enum") w3042 w3108 w3125 myRIO_BRig_RT__Case_Exp_stateList."initBlock" ("Enum") w3152 myRIO_BRig_RT__Case_Exp_stateList."commUpload_dataExp" ("Enum") myRIO_BRig_RT__Case_Exp_stateList."endBlock" ("Enum") myRIO_BRig_RT__Case_Exp_stateList."commUpload_dataLC" ("Enum") myRIO_BRig_RT__Case_Exp_stateList."commUpload_dataTrial" ("Enum") myRIO_BRig_RT__Case_Exp_stateList."commUpload_dataCurrent" ("Enum") myRIO_BRig_RT__Case_Exp_stateList."saveData_dataCurrent" ("Enum") myRIO_BRig_RT__Case_Exp_stateList."saveData_dataExp" ("Enum") myRIO_BRig_RT__Case_Exp_stateList."saveData_dataLC" ("Enum") myRIO_BRig_RT__Case_Exp_stateList."saveData_dataTrial" ("Enum") myRIO_BRig_RT__Case_Exp_stateList."commUpload_pre" ("Enum") w3405 w3438] -> w1123
            tunnel: [w1202 w1221 w1243 w1298 w1346 w1414 w1481 w1545 w1609 w1673 w1737 w1780 w1824 w1850 w1915 w1921 w1952 w1966 w2005 w2036 w2072 w2097 w2122 w2139 w2183 w2225 w2263 w2294 w2322 w2338 w2360 w2379 w2398 w2438 w2489 w2515 w2544 w2565 w2586 w2605 w2624 w2653 w2726 w2751 w2774 w2788 w2838 w2862 w2894 w2915 w2935 w2966 w2989 w3001 w3020 w3062 w3081 w3124 w3141 w3155 w3189 w3210 w3231 w3252 w3273 w3301 w3321 w3348 w3368 w3392 w3426 w3459] -> w1055
            tunnel: w1172 -> [w1202 w1221 w1243 w1298 w1346 w1414 w1481 w1545 w1609 w1673 w1737 w1780 w1824 w1850 w1915 w1943 w1952 w1966 w2005 w2036 w2072 w2097 w2122 w2139 w2183 w2225 w2263 w2294 w2322 w2338 w2360 w2379 w2398 w2438 w2489 w2515 w2544 w2565 w2586 w2605 w2624 w2653 w2726 w2751 w2774 w2788 w2838 w2862 w2894 w2915 w2935 w2966 w2989 w3001 w3020 w3062 w3081 w3124 w3141 w3155 w3189 w3210 w3231 w3252 w3273 w3301 w3321 w3348 w3368 w3392 w3426 w3459]
            tunnel: w1171 -> [w1205 w1224 w1240 w1301 w1349 w1417 w1484 w1548 w1612 w1676 w1740 w1783 w1827 w1853 w1918 w1937 w1963 w1990 w2023 w2052 w2086 w2110 w2135 w2166 w2196 w2212 w2244 w2297 w2325 w2344 w2363 w2382 w2401 w2420 w2466 w2523 w2551 w2570 w2589 w2608 w2627 w2651 w2724 w2761 w2784 w2819 w2846 w2873 w2897 w2914 w2947 w2971 w2986 w3009 w3019 w3073 w3107 w3128 w3138 w3164 w3192 w3213 w3234 w3255 w3276 w3304 w3324 w3351 w3371 w3395 w3429 w3462]
            tunnel: w1166 -> [w1204 w1223 w1241 w1300 w1348 w1416 w1483 w1547 w1611 w1675 w1739 w1782 w1826 w1852 w1917 w1936 w1962 w1991 w2022 w2053 w2087 w2111 w2136 w2167 w2197 w2235 w2265 w2296 w2324 w2343 w2362 w2381 w2400 w2452 w2490 w2522 w2550 w2569 w2588 w2607 w2626 w2652 w2723 w2760 w2783 w2818 w2845 w2872 w2896 w2913 w2946 w2970 w2987 w3010 w3018 w3072 w3106 w3127 w3139 w3165 w3191 w3212 w3233 w3254 w3275 w3303 w3323 w3350 w3370 w3394 w3428 w3461]
            tunnel: w1165 -> [w1203 w1222 w1242 w1299 w1347 w1415 w1482 w1546 w1610 w1674 w1738 w1781 w1825 w1851 w1916 w1935 w1961 w1992 w2021 w2054 w2088 w2112 w2137 w2168 w2198 w2234 w2264 w2295 w2323 w2342 w2361 w2380 w2399 w2451 w2491 w2521 w2549 w2568 w2587 w2606 w2625 w2670 w2727 w2759 w2782 w2817 w2844 w2871 w2895 w2912 w2945 w2969 w2988 w3011 w3017 w3071 w3105 w3126 w3140 w3166 w3190 w3211 w3232 w3253 w3274 w3302 w3322 w3349 w3369 w3393 w3427 w3460]
            tunnel: [w1205 w1224 w1240 w1301 w1349 w1417 w1484 w1548 w1612 w1676 w1740 w1783 w1827 w1853 w1918 w1937 w1963 w1990 w2023 w2052 w2086 w2110 w2135 w2166 w2196 w2212 w2244 w2297 w2325 w2344 w2363 w2382 w2401 w2420 w2466 w2523 w2551 w2570 w2589 w2608 w2627 w2651 w2724 w2761 w2784 w2819 w2846 w2873 w2897 w2914 w2947 w2971 w2986 w3009 w3019 w3073 w3107 w3128 w3138 w3164 w3192 w3213 w3234 w3255 w3276 w3304 w3324 w3351 w3371 w3395 w3429 w3462] -> w1154
            tunnel: [w1204 w1223 w1241 w1300 w1348 w1416 w1483 w1547 w1611 w1675 w1739 w1782 w1826 w1852 w1917 w1936 w1962 w1991 w2022 w2053 w2087 w2111 w2136 w2167 w2197 w2235 w2265 w2296 w2324 w2343 w2362 w2381 w2400 w2452 w2490 w2522 w2550 w2569 w2588 w2607 w2626 w2652 w2723 w2760 w2783 w2818 w2845 w2872 w2896 w2913 w2946 w2970 w2987 w3010 w3018 w3072 w3106 w3127 w3139 w3165 w3191 w3212 w3233 w3254 w3275 w3303 w3323 w3350 w3370 w3394 w3428 w3461] -> w1153
            tunnel: [w1203 w1222 w1242 w1299 w1347 w1415 w1482 w1546 w1610 w1674 w1738 w1781 w1825 w1851 w1916 w1935 w1961 w1992 w2021 w2054 w2088 w2112 w2137 w2168 w2198 w2234 w2264 w2295 w2323 w2342 w2361 w2380 w2399 w2451 w2491 w2521 w2549 w2568 w2587 w2606 w2625 w2670 w2727 w2759 w2782 w2817 w2844 w2871 w2895 w2912 w2945 w2969 w2988 w3011 w3017 w3071 w3105 w3126 w3140 w3166 w3190 w3211 w3232 w3253 w3274 w3302 w3322 w3349 w3369 w3393 w3427 w3460] -> w1152
            tunnel: w1115 -> [w1201 w1220 w1239 w1265 w1322 w1391 w1466 w1544 w1608 w1672 w1736 w1779 w1823 w1848 w1891 w1942 w1951 w1988 w1994 w2037 w2067 w2094 w2121 w2149 w2182 w2224 w2249 w2288 w2321 w2339 w2359 w2378 w2397 w2424 w2486 w2514 w2548 w2566 w2585 w2604 w2623 w2637 w2704 w2743 w2779 w2790 w2843 w2863 w2893 w2911 w2936 w2968 w2985 w2998 w3022 w3044 w3079 w3123 w3142 w3167 w3186 w3207 w3228 w3249 w3260 w3290 w3309 w3333 w3365 w3381 w3404 w3437]
            tunnel: w1112 -> [w1200 w1219 w1238 w1296 w1344 w1411 w1478 w1542 w1606 w1670 w1734 w1777 w1821 w1841 w1911 w1941 w1960 w1987 w2002 w2035 w2074 w2100 w2125 w2156 w2186 w2227 w2262 w2287 w2319 w2341 w2358 w2377 w2396 w2440 w2488 w2512 w2543 w2567 w2584 w2603 w2622 w2663 w2725 w2757 w2781 w2811 w2839 w2864 w2891 w2910 w2938 w2965 w2984 w3008 w3025 w3043 w3098 w3122 w3143 w3168 w3185 w3206 w3227 w3248 w3261 w3298 w3318 w3329 w3364 w3389 w3423 w3456]
            tunnel: [w1201 w1220 w1239 w1265 w1322 w1390 w1465 w1544 w1608 w1672 w1736 w1779 w1823 w1848 w1897 w1926 w1951 w1976 w1994 w2037 w2067 w2093 w2120 w2148 w2181 w2228 w2248 w2289 w2320 w2339 w2359 w2378 w2397 w2447 w2485 w2513 w2546 w2566 w2585 w2604 w2623 w2664 w2701 w2758 w2778 w2812 w2842 w2865 w2892 w2911 w2939 w2967 w2985 w2997 w3021 w3044 w3077 w3123 w3142 w3167 w3186 w3207 w3228 w3249 w3260 w3290 w3309 w3333 w3365 w3381 w3404 w3437] -> w1149
            tunnel: [w1200 w1219 w1238 w1295 w1343 w1406 w1477 w1542 w1606 w1670 w1734 w1777 w1821 w1841 w1911 w1940 w1960 w1986 w2002 w2035 w2074 w2100 w2125 w2156 w2186 w2227 w2262 w2287 w2319 w2341 w2358 w2377 w2396 w2440 w2488 w2512 w2543 w2567 w2584 w2603 w2622 w2663 w2725 w2757 w2781 w2811 w2839 w2864 w2891 w2910 w2938 w2965 w2984 w3008 w3025 w3043 w3098 w3122 w3143 w3168 w3185 w3206 w3227 w3248 w3261 w3298 w3318 w3332 w3364 w3389 w3423 w3456] -> w1162
            tunnel: [_ _ _ _ _ _ _ _ _ _ _ _ _ _ _ _ _ _ _ _ _ _ _ _ _ _ _ _ _ _ _ _ _ _ _ _ _ _ _ _ _ _ _ _ w2772 _ _ _ _ _ _ _ _ _ _ _ _ _ _ _ _ _ _ _ _ _ _ _ _ _ _ _] -> w1046
            tunnel: [_ _ _ _ _ _ _ _ _ _ _ _ _ _ _ _ _ _ _ _ _ _ _ _ _ _ _ _ _ _ _ _ _ _ _ _ _ _ _ _ _ _ _ _ w2773 _ _ _ _ _ _ _ _ _ _ _ _ _ _ _ _ _ _ _ _ _ _ _ _ _ _ _] -> w1126
            tunnel: w1161 -> [w1198 w1217 w1236 w1267 w1324 w1412 w1479 w1543 w1607 w1671 w1735 w1778 w1822 w1846 w1912 w1938 w1953 w1984 w2014 w2050 w2084 w2090 w2117 w2138 w2178 w2226 w2261 w2284 w2315 w2340 w2356 w2375 w2394 w2446 w2487 w2511 w2541 w2563 w2582 w2601 w2620 w2662 w2721 w2749 w2780 w2792 w2836 w2861 w2889 w2908 w2937 w2964 w2982 w3000 w3027 w3069 w3090 w3120 w3145 w3170 w3183 w3204 w3225 w3246 w3270 w3284 w3311 w3339 w3358 w3383 w3417 w3450]
            tunnel: [w1198 w1217 w1236 w1267 w1324 w1412 w1479 w1543 w1607 w1671 w1735 w1778 w1822 w1846 w1912 w1938 w1950 w1984 w2014 w2050 w2084 w2090 w2117 w2138 w2178 w2226 w2261 w2284 w2315 w2340 w2356 w2375 w2394 w2446 w2487 w2511 w2541 w2563 w2582 w2601 w2620 w2662 w2721 w2749 w2780 w2791 w2836 w2861 w2889 w2908 w2937 w2964 w2982 w2999 w3027 w3069 w3090 w3120 w3145 w3170 w3183 w3204 w3225 w3246 w3270 w3284 w3311 w3339 w3358 w3383 w3417 w3450] -> w1160
            tunnel: w1159 -> [w1199 w1218 w1237 w1266 w1323 w1413 w1480 w1540 w1604 w1668 w1732 w1775 w1819 w1847 w1913 w1939 w1959 w1985 w1993 w2051 w2085 w2098 w2123 w2154 w2184 w2223 w2243 w2285 w2316 w2337 w2357 w2376 w2395 w2445 w2465 w2510 w2542 w2564 w2583 w2602 w2621 w2661 w2722 w2750 w2775 w2809 w2837 w2860 w2890 w2909 w2934 w2963 w2983 w3007 w3026 w3070 w3097 w3121 w3144 w3169 w3184 w3205 w3226 w3247 w3271 w3297 w3317 w3345 w3356 w3388 w3422 w3455]
            tunnel: [w1199 w1218 w1237 w1266 w1323 w1413 w1480 w1541 w1605 w1669 w1733 w1776 w1820 w1847 w1913 w1939 w1959 w1985 w1993 w2051 w2085 w2098 w2123 w2154 w2184 w2223 w2243 w2285 w2316 w2337 w2357 w2376 w2395 w2445 w2465 w2510 w2542 w2564 w2583 w2602 w2621 w2661 w2722 w2750 w2775 w2809 w2837 w2860 w2890 w2909 w2934 w2963 w2983 w3007 w3026 w3070 w3097 w3121 w3144 w3169 w3184 w3205 w3226 w3247 w3271 w3297 w3317 w3345 w3356 w3388 w3422 w3455] -> w1158
            tunnel: [_ _ _ _ _ _ _ _ _ _ _ _ _ _ _ _ _ _ _ _ _ _ _ _ _ _ _ _ _ _ _ _ _ _ _ _ _ _ _ _ _ _ _ _ _ _ _ _ _ _ _ _ _ _ _ _ _ TRUE _ _ _ _ _ _ _ _ _ _ _ _ _ _] -> w1155
            tunnel: w1145 -> [w1196 w1215 w1234 w1257 w1317 w1401 w1476 w1527 w1591 w1655 w1719 w1747 w1791 _ w1903 w1934 w1958 w1983 w2013 w2049 w2083 w2109 w2134 w2165 w2195 w2222 w2260 w2282 w2314 w2335 w2354 w2373 w2392 w2444 w2482 w2508 w2540 w2561 w2580 w2599 w2618 w2660 w2720 w2739 w2771 w2807 w2835 w2858 w2888 w2907 w2932 w2962 w2981 w3005 w3031 w3068 w3094 w3118 w3136 w3163 w3181 w3202 w3223 w3244 w3268 w3295 w3315 w3343 w3362 w3387 w3421 w3454]
            tunnel: w1144 -> [w1195 w1214 w1233 w1256 w1316 w1400 w1475 w1526 w1590 w1654 w1718 w1748 w1792 _ w1902 w1933 w1957 w1982 w2012 w2048 w2082 w2108 w2133 w2164 w2194 w2221 w2259 w2281 w2313 w2334 w2353 w2372 w2391 w2443 w2481 w2507 w2539 w2560 w2579 w2598 w2617 w2659 w2719 w2738 w2770 w2806 w2834 w2857 w2887 w2906 w2931 w2961 w2980 w3004 w3030 w3067 w3093 w3117 w3135 w3162 w3180 w3201 w3222 w3243 w3267 w3294 w3314 w3342 w3361 w3386 w3420 w3453]
            tunnel: w1143 -> [w1194 w1213 w1232 w1255 w1315 w1399 w1474 w1525 w1589 w1653 w1717 w1749 w1793 _ w1901 w1932 w1956 w1981 w2011 w2047 w2081 w2107 w2132 w2163 w2193 w2220 w2258 w2280 w2312 w2333 w2352 w2371 w2390 w2442 w2480 w2506 w2538 w2559 w2578 w2597 w2616 w2658 w2718 w2737 w2769 w2805 w2833 w2856 w2886 w2905 w2930 w2960 w2979 w3003 w3029 w3066 w3092 w3116 w3134 w3161 w3179 w3200 w3221 w3242 w3266 w3293 w3313 w3341 w3360 w3385 w3419 w3452]
            tunnel: w1142 -> [w1193 w1212 w1231 w1254 w1314 w1398 w1473 w1524 w1588 w1652 w1716 w1750 w1794 _ w1900 w1931 w1955 w1980 w2010 w2046 w2080 w2106 w2131 w2162 w2192 w2219 w2257 w2279 w2311 w2332 w2351 w2370 w2389 w2441 w2479 w2505 w2537 w2558 w2577 w2596 w2615 w2657 w2717 w2736 w2768 w2804 w2832 w2855 w2885 w2904 w2929 w2959 w2978 w3002 w3028 w3065 w3091 w3115 w3133 w3160 w3178 w3199 w3220 w3241 w3265 w3292 w3312 w3340 w3359 w3384 w3418 w3451]
            tunnel: w1141 -> [_ _ _ _ _ _ _ _ _ _ _ _ _ _ _ _ _ _ _ _ _ _ _ _ _ _ _ _ _ _ _ _ _ _ w2484 _ _ _ _ _ _ _ _ _ _ _ _ _ _ _ _ _ _ _ _ _ _ _ _ _ _ _ _ _ _ _ _ _ _ _ _ _]
            tunnel: w1140 -> [_ _ _ _ _ _ _ _ _ _ _ _ _ _ _ _ _ _ _ _ _ _ _ _ _ _ _ _ _ _ _ _ _ _ w2483 _ _ _ _ _ _ _ _ _ _ _ _ _ _ _ _ _ _ _ _ _ _ _ _ _ _ _ _ _ _ _ _ _ _ _ _ _]
            tunnel: [w1196 w1215 w1234 w1257 w1317 w1401 w1476 w1527 w1591 w1655 w1719 w1747 w1791 w1840 w1903 w1934 w1958 w1983 w2013 w2049 w2083 w2109 w2134 w2165 w2195 w2222 w2260 w2282 w2314 w2335 w2354 w2373 w2392 w2444 w2482 w2508 w2540 w2561 w2580 w2599 w2618 w2660 w2720 w2739 w2771 w2807 w2835 w2858 w2888 w2907 w2932 w2962 w2981 w3005 w3031 w3068 w3094 w3118 w3136 w3163 w3181 w3202 w3223 w3244 w3268 w3295 w3315 w3343 w3362 w3387 w3421 w3454] -> w1137
            tunnel: [w1195 w1214 w1233 w1256 w1316 w1400 w1475 w1526 w1590 w1654 w1718 w1748 w1792 w1831 w1902 w1933 w1957 w1982 w2012 w2048 w2082 w2108 w2133 w2164 w2194 w2221 w2259 w2281 w2313 w2334 w2353 w2372 w2391 w2443 w2481 w2507 w2539 w2560 w2579 w2598 w2617 w2659 w2719 w2738 w2770 w2806 w2834 w2857 w2887 w2906 w2931 w2961 w2980 w3004 w3030 w3067 w3093 w3117 w3135 w3162 w3180 w3201 w3222 w3243 w3267 w3294 w3314 w3342 w3361 w3386 w3420 w3453] -> w1109
            tunnel: [w1194 w1213 w1232 w1255 w1315 w1399 w1474 w1525 w1589 w1653 w1717 w1749 w1793 w1839 w1901 w1932 w1956 w1981 w2011 w2047 w2081 w2107 w2132 w2163 w2193 w2220 w2258 w2280 w2312 w2333 w2352 w2371 w2390 w2442 w2480 w2506 w2538 w2559 w2578 w2597 w2616 w2658 w2718 w2737 w2769 w2805 w2833 w2856 w2886 w2905 w2930 w2960 w2979 w3003 w3029 w3066 w3092 w3116 w3134 w3161 w3179 w3200 w3221 w3242 w3266 w3293 w3313 w3341 w3360 w3385 w3419 w3452] -> w1138
            tunnel: [w1193 w1212 w1231 w1254 w1314 w1398 w1473 w1524 w1588 w1652 w1716 w1750 w1794 w1829 w1900 w1931 w1955 w1980 w2010 w2046 w2080 w2106 w2131 w2162 w2192 w2219 w2257 w2279 w2311 w2332 w2351 w2370 w2389 w2441 w2479 w2505 w2537 w2558 w2577 w2596 w2615 w2657 w2717 w2736 w2768 w2804 w2832 w2855 w2885 w2904 w2929 w2959 w2978 w3002 w3028 w3065 w3091 w3115 w3133 w3160 w3178 w3199 w3220 w3241 w3265 w3292 w3312 w3340 w3359 w3384 w3418 w3451] -> w1139
            tunnel: [_ _ _ _ _ _ _ _ _ _ _ _ _ _ _ _ _ _ _ _ _ _ _ _ _ _ _ _ _ _ _ _ _ w2405 w2484 _ _ _ _ _ _ _ _ _ _ _ _ _ _ _ _ _ _ _ _ _ _ _ _ _ _ _ _ _ _ _ _ _ _ _ _ _] -> w1111
            tunnel: [_ _ _ _ _ _ _ _ _ _ _ _ _ _ _ _ _ _ _ _ _ _ _ _ _ _ _ _ _ _ _ _ _ w2403 w2483 _ _ _ _ _ _ _ _ _ _ _ _ _ _ _ _ _ _ _ _ _ _ _ _ _ _ _ _ _ _ _ _ _ _ _ _ _] -> w1110
            tunnel: w1122 -> [w1192 w1211 w1230 w1253 w1313 w1397 w1472 w1523 w1587 w1651 w1715 w1746 w1790 w1838 w1910 w1930 w1954 w1979 w1996 w2039 w2066 w2092 w2119 w2150 w2180 w2218 w2256 w2278 w2310 w2331 w2350 w2369 w2388 w2431 w2478 w2504 w2536 w2557 w2576 w2595 w2614 w2656 w2716 w2733 w2767 w2803 w2831 w2852 w2879 w2903 w2926 w2953 w2977 w2996 w3024 w3058 w3089 w3114 w3146 w3171 w3182 w3203 w3224 w3245 w3269 w3296 w3316 w3344 w3363 w3378 w3416 w3449]
            tunnel: [w1192 w1211 w1230 w1253 w1313 w1397 w1472 w1523 w1587 w1651 w1715 w1746 w1790 w1838 w1910 w1930 w1954 w1979 w1995 w2038 w2059 w2091 w2118 w2150 w2179 w2218 w2256 w2278 w2310 w2331 w2350 w2369 w2388 w2431 w2478 w2504 w2536 w2557 w2576 w2595 w2614 w2656 w2716 w2733 w2767 w2803 w2831 w2852 w2879 w2903 w2926 w2953 w2977 w2996 w3023 w3058 w3089 w3114 w3146 w3171 w3182 w3203 w3224 w3245 w3269 w3296 w3316 w3344 w3363 w3378 w3416 w3449] -> w1121
            tunnel: [w1191 w1210 w1229 w1252 w1312 w1396 w1471 w1522 w1586 w1650 w1714 w1745 w1789 w1837 w1909 w1929 w1965 w1978 w2016 w2045 w2079 w2105 w2130 w2161 w2191 w2217 w2255 w2277 w2309 w2330 w2349 w2368 w2387 w2430 w2477 w2503 w2535 w2556 w2575 w2594 w2613 w2655 w2715 w2732 w2766 w2802 w2830 w2851 w2878 w2902 w2925 w2952 w2976 w2995 w3016 w3064 w3088 w3112 w3147 w3157 w3177 w3198 w3219 w3240 w3264 w3300 w3320 w3347 w3367 w3391 w3425 w3458] -> w1120
            tunnel: [w1190 w1209 w1228 w1251 w1311 w1395 w1470 w1521 w1585 w1649 w1713 w1744 w1788 w1836 w1908 w1928 w1964 w1977 w2015 w2044 w2078 w2104 w2129 w2160 w2190 w2216 w2254 w2276 w2308 w2329 w2348 w2367 w2386 w2429 w2476 w2502 w2534 w2555 w2574 w2593 w2612 w2654 w2714 w2731 w2765 w2801 w2829 w2850 w2877 w2901 w2924 w2951 w2975 w2994 w3015 w3063 w3087 w3113 w3129 w3154 w3187 w3208 w3229 w3250 w3272 w3299 w3319 w3346 w3366 w3390 w3424 w3457] -> w1119
            tunnel: w1118 -> [w1191 w1210 w1229 w1252 w1312 w1396 w1471 w1522 w1586 w1650 w1714 w1745 w1789 w1837 w1909 w1929 w1965 w1978 w2016 w2045 w2079 w2105 w2130 w2161 w2191 w2217 w2255 w2277 w2309 w2330 w2349 w2368 w2387 w2430 w2477 w2503 w2535 w2556 w2575 w2594 w2613 w2655 w2715 w2732 w2766 w2802 w2830 w2851 w2878 w2902 w2925 w2952 w2976 w2995 w3016 w3064 w3088 w3112 _ w3157 w3177 w3198 w3219 w3240 w3264 w3300 w3320 w3347 w3367 w3391 w3425 w3458]
            tunnel: w1117 -> [w1190 w1209 w1228 w1251 w1311 w1395 w1470 w1521 w1585 w1649 w1713 w1744 w1788 w1836 w1908 w1928 w1964 w1977 w2015 w2044 w2078 w2104 w2129 w2160 w2190 w2216 w2254 w2276 w2308 w2329 w2348 w2367 w2386 w2429 w2476 w2502 w2534 w2555 w2574 w2593 w2612 w2654 w2714 w2731 w2765 w2801 w2829 w2850 w2877 w2901 w2924 w2951 w2975 w2994 w3015 w3063 w3087 w3113 _ w3154 w3187 w3208 w3229 w3250 w3272 w3299 w3319 w3346 w3366 w3390 w3424 w3457]
            tunnel: w1116 -> [_ _ _ _ _ _ _ _ _ _ _ _ _ _ _ _ _ _ _ _ _ _ _ _ _ _ _ _ _ _ _ _ _ _ _ _ _ _ _ _ _ _ _ _ _ _ _ _ _ _ _ _ _ _ _ _ _ _ _ _ w3175 w3196 w3217 w3238 w3262 _ _ _ _ _ _ _]
            tunnel: w1114 -> [_ _ _ _ _ _ _ _ _ _ _ _ _ _ _ _ _ _ _ _ w2071 _ w2116 w2153 w2177 w2206 w2242 w2270 w2301 _ _ _ _ w2413 w2462 w2498 w2528 _ _ _ _ _ _ _ _ _ _ _ _ _ _ _ _ _ _ _ _ _ _ _ _ _ _ _ _ _ _ _ _ _ _ _]
            tunnel: w1113 -> [_ _ _ _ _ _ _ _ _ _ _ _ _ _ _ _ _ _ _ _ _ _ _ _ _ _ _ _ _ _ _ _ _ _ _ _ _ _ _ _ _ _ _ _ _ _ _ _ _ _ _ _ _ _ _ _ _ _ _ _ _ _ _ _ _ _ _ w3334 _ _ _ _]
            tunnel: [w1189 w1208 w1227 w1250 w1310 w1394 w1469 w1520 w1584 w1648 w1712 w1743 w1787 w1835 w1907 w1924 w1948 w1974 w2017 w2043 w2077 w2103 w2128 w2159 w2189 w2215 w2253 w2275 w2307 w2328 w2347 w2366 w2385 w2428 w2475 w2501 w2533 w2554 w2573 w2592 w2611 w2650 w2713 w2730 w2764 w2786 w2828 w2849 w2876 w2900 w2923 w2950 w2974 w2993 w3014 w3061 w3074 w3111 w3132 w3156 w3174 w3195 w3216 w3237 w3259 w3279 w3308 w3328 w3355 w3376 w3415 w3448] -> w1107
            tunnel: w1108 -> [w1189 w1208 w1227 w1250 w1310 w1394 w1469 w1520 w1584 w1648 w1712 w1743 w1787 w1835 w1907 w1924 _ w1974 w2017 w2043 w2077 w2103 w2128 w2159 w2189 w2215 w2253 w2275 w2307 w2328 w2347 w2366 w2385 w2428 w2475 w2501 w2533 w2554 w2573 w2592 w2611 w2650 w2713 w2730 w2764 w2786 w2828 w2849 w2876 w2900 w2923 w2950 w2974 w2993 w3014 w3061 w3075 w3111 w3132 w3156 w3174 w3195 w3216 w3237 w3259 w3279 w3308 w3328 w3355 w3376 w3415 w3448]
            tunnel: w1106 -> [w1188 w1207 w1226 w1249 w1309 w1393 w1468 w1519 w1583 w1647 w1711 w1742 w1786 w1834 w1906 w1923 w1947 w1973 w2009 w2042 w2076 w2102 w2127 w2158 w2188 w2214 w2252 w2274 w2306 w2327 w2346 w2365 w2384 w2427 w2474 w2500 w2532 w2553 w2572 w2591 w2610 w2649 w2712 w2729 w2763 w2800 w2827 w2848 w2875 w2899 w2922 w2949 w2973 w2992 w3013 w3060 w3086 w3110 w3131 w3159 w3173 w3194 w3215 w3236 w3258 w3278 w3307 w3327 w3354 w3375 w3414 w3447]
            tunnel: w1105 -> [w1187 w1206 w1225 w1248 w1308 w1392 w1467 w1518 w1582 w1646 w1710 w1741 w1785 w1833 w1905 w1922 w1946 w1972 w2008 w2041 w2075 w2101 w2126 w2157 w2187 w2213 w2251 w2273 w2305 w2326 w2345 w2364 w2383 w2426 w2473 w2499 w2531 w2552 w2571 w2590 w2609 w2648 w2711 w2728 w2762 w2797 w2826 w2847 w2874 w2898 w2921 w2948 w2972 w2991 w3012 w3059 w3085 w3109 w3130 w3158 w3172 w3193 w3214 w3235 w3257 w3277 w3306 w3326 w3353 w3374 w3413 w3446]
            tunnel: [w1188 w1207 w1226 w1249 w1309 w1393 w1468 w1519 w1583 w1647 w1711 w1742 w1786 w1834 w1906 w1923 w1947 w1973 w2009 w2042 w2076 w2102 w2127 w2158 w2188 w2214 w2252 w2274 w2306 w2327 w2346 w2365 w2384 w2427 w2474 w2500 w2532 w2553 w2572 w2591 w2610 w2649 w2712 w2729 w2763 w2799 w2827 w2848 w2875 w2899 w2922 w2949 w2973 w2992 w3013 w3060 w3086 w3110 w3131 w3159 w3173 w3194 w3215 w3236 w3258 w3278 w3307 w3327 w3354 w3375 w3414 w3447] -> w1104
            tunnel: [w1187 w1206 w1225 w1248 w1308 w1392 w1467 w1518 w1582 w1646 w1710 w1741 w1785 w1833 w1905 w1922 w1946 w1972 w2008 w2041 w2075 w2101 w2126 w2157 w2187 w2213 w2251 w2273 w2305 w2326 w2345 w2364 w2383 w2426 w2473 w2499 w2531 w2552 w2571 w2590 w2609 w2648 w2711 w2728 w2762 w2798 w2826 w2847 w2874 w2898 w2921 w2948 w2972 w2991 w3012 w3059 w3085 w3109 w3130 w3158 w3172 w3193 w3214 w3235 w3257 w3277 w3306 w3326 w3353 w3374 w3413 w3446] -> w1103
            tunnel: w1102 -> [w1186 _ _ _ _ _ _ _ _ _ _ _ _ _ w1898 _ _ _ w2020 w2031 _ _ _ _ _ _ _ _ _ _ _ _ _ _ w2470 _ _ _ _ _ _ w2646 w2710 _ _ _ _ _ _ _ w2920 _ _ _ _ w3040 _ _ _ _ _ _ _ _ _ _ _ _ _ _ _ _]
            tunnel: w1101 -> [w1185 _ _ _ _ _ _ _ _ _ _ _ _ _ w1899 _ _ _ w2019 w2030 _ _ _ _ _ _ _ _ _ _ _ _ _ _ w2469 _ _ _ _ _ _ w2647 w2709 _ _ _ _ _ _ _ w2919 _ _ _ _ w3039 _ _ _ _ _ _ _ _ _ _ _ _ _ _ _ _]
            tunnel: w1099 -> [_ _ _ _ _ _ _ _ _ _ _ _ _ _ _ _ _ _ _ _ w2070 _ w2115 w2152 w2176 w2205 w2241 w2269 w2302 _ _ _ _ w2412 w2461 w2497 w2527 _ _ _ _ _ _ _ _ _ _ _ _ _ _ _ _ _ _ _ _ _ _ _ _ _ _ _ _ _ _ _ _ _ _ _]
            tunnel: w1098 -> [_ _ _ _ _ _ _ _ _ _ _ _ _ _ _ _ _ _ _ _ w2069 _ _ _ w2173 w2208 w2246 w2272 w2303 _ _ _ _ w2418 w2464 w2496 w2530 _ _ _ _ _ _ _ _ _ _ _ _ _ _ _ _ _ _ _ _ _ _ _ _ _ _ _ _ _ _ _ _ _ _ _]
            tunnel: w1097 -> [_ _ _ _ _ _ _ _ _ _ _ _ _ _ _ _ _ _ _ _ w2068 _ _ _ w2172 w2207 w2245 w2271 w2304 _ _ _ _ w2417 w2463 w2495 w2529 _ _ _ _ _ _ _ _ _ _ _ _ _ _ _ _ _ _ _ _ _ _ _ _ _ _ _ _ _ _ _ _ _ _ _]
            tunnel: [_ _ _ _ _ _ _ _ _ _ _ _ _ _ _ _ _ _ _ _ w2069 _ _ _ w2173 w2208 w2246 w2272 w2303 _ _ _ _ w2418 w2464 w2496 w2530 _ _ _ _ _ _ _ _ _ _ _ _ _ _ _ _ _ _ _ _ _ _ _ _ _ _ _ _ _ _ _ _ _ _ _] -> w1096
            tunnel: [_ _ _ _ _ _ _ _ _ _ _ _ _ _ _ _ _ _ _ _ w2068 _ _ _ w2172 w2207 w2245 w2271 w2304 _ _ _ _ w2417 w2463 w2495 w2529 _ _ _ _ _ _ _ _ _ _ _ _ _ _ _ _ _ _ _ _ _ _ _ _ _ _ _ _ _ _ _ _ _ _ _] -> w1095
            tunnel: [_ _ _ _ _ _ _ _ _ _ _ _ _ _ _ _ _ _ _ _ w2071 w2095 w2116 w2153 w2177 w2206 w2242 w2270 w2301 _ _ _ _ w2413 w2462 w2498 w2528 _ _ _ _ _ _ _ _ _ _ _ _ _ _ _ _ _ _ _ _ _ _ _ _ _ _ _ _ _ _ _ _ _ _ _] -> w1094
            tunnel: [_ _ _ _ _ _ _ _ _ _ _ _ _ _ _ _ _ _ _ _ w2070 w2096 w2115 w2152 w2176 w2205 w2241 w2269 w2302 _ _ _ _ w2412 w2461 w2497 w2527 _ _ _ _ _ _ _ _ _ _ _ _ _ _ _ _ _ _ _ _ _ _ _ _ _ _ _ _ _ _ _ _ _ _ _] -> w1093
            tunnel: [_ _ _ _ _ _ _ _ _ _ _ _ _ _ _ _ _ _ _ _ _ _ _ _ _ _ w2240 _ _ _ _ _ _ _ w2457 _ _ _ _ _ _ w2629 w2688 _ _ _ _ _ _ _ _ _ _ _ _ _ _ _ _ _ _ _ _ _ _ _ _ _ _ _ _ _] -> w1090
            tunnel: [_ _ _ _ _ _ _ _ _ _ _ _ _ _ _ _ _ _ _ _ _ _ _ _ _ _ w2239 _ _ _ _ _ _ _ w2456 _ _ _ _ _ _ w2628 w2689 _ _ _ _ _ _ _ _ _ _ _ _ _ _ _ _ _ _ _ _ _ _ _ _ _ _ _ _ _] -> w1092
            tunnel: [_ _ _ _ _ _ _ _ _ _ _ _ _ _ _ _ _ _ _ _ _ _ _ w2151 w2175 _ _ _ _ _ _ _ _ _ _ _ _ _ _ _ _ _ _ _ _ _ _ _ _ _ _ _ _ _ _ _ _ _ _ _ _ _ _ _ _ _ _ _ _ _ _ _] -> w1087
            tunnel: [_ _ _ _ _ _ _ _ _ _ _ _ _ _ _ _ _ _ _ _ _ _ _ _ TRUE ("Recording") _ _ _ _ _ _ _ _ _ _ _ _ _ _ _ _ _ _ _ _ _ _ _ _ _ _ _ _ _ _ _ _ _ _ _ _ _ _ _ _ _ _ _ _ _ _ _] -> w1084
            tunnel: [_ _ _ _ _ _ _ _ _ _ _ _ _ _ _ _ _ _ _ _ _ _ _ w2151 _ _ _ _ _ _ _ _ _ _ _ _ _ _ _ _ _ _ _ _ _ _ _ _ _ _ _ _ _ _ _ _ _ _ _ _ _ _ _ _ _ _ _ _ _ _ _ _] -> w1080
            tunnel: [_ _ _ _ _ _ _ _ _ _ _ _ _ _ _ TRUE _ _ _ _ _ _ _ _ _ _ _ _ _ _ _ _ _ _ _ _ _ _ _ _ _ _ _ _ _ _ _ _ _ _ _ _ _ _ _ _ _ _ _ _ _ _ _ _ _ _ _ _ _ _ _ _] -> w1077
            tunnel: [_ _ _ _ _ _ _ _ _ _ _ _ _ _ _ w1919 _ _ _ _ _ _ _ _ _ _ _ _ _ _ _ _ _ _ _ _ _ _ _ _ _ _ _ _ _ _ _ _ _ _ _ _ _ _ _ _ _ _ _ _ _ _ _ _ _ _ _ _ _ _ _ _] -> w1075
            tunnel: [_ _ _ _ _ _ _ _ _ _ _ _ _ _ _ _ _ TRUE _ _ _ _ _ _ _ _ _ _ _ _ _ _ _ _ _ _ _ _ _ _ _ _ _ _ _ _ _ _ _ _ _ _ _ _ _ _ _ _ _ _ _ _ _ _ _ _ _ _ _ _ _ _] -> w1074
            tunnel: [_ _ _ _ _ _ _ _ _ _ _ _ _ _ _ _ _ w1967 _ _ _ _ _ _ _ _ _ _ _ _ _ _ _ _ _ _ _ _ _ _ _ _ _ _ _ _ _ _ _ _ _ _ _ _ _ _ _ _ _ _ _ _ _ _ _ _ _ _ _ _ _ _] -> w1073
            tunnel: w1062 -> [_ _ _ _ _ _ _ _ _ _ _ _ _ _ _ _ _ _ _ _ w2057 _ _ _ _ w2201 w2238 w2268 w2300 _ _ _ _ w2411 w2460 w2494 w2526 _ _ _ _ w2632 w2683 _ _ _ _ _ _ _ _ _ _ _ _ _ _ _ _ _ _ _ _ _ _ _ _ _ _ _ _ _]
            tunnel: [_ _ _ _ _ _ _ _ _ _ _ _ _ _ _ _ _ _ _ _ w2057 _ _ _ w2171 w2201 w2238 w2268 w2300 _ _ _ _ w2411 w2460 w2494 w2526 _ _ _ _ w2632 w2683 _ _ _ _ _ _ _ _ _ _ _ _ _ _ _ _ _ _ _ _ _ _ _ _ _ _ _ _ _] -> w1061
            tunnel: w1060 -> [_ _ _ _ _ _ _ _ _ _ _ _ _ _ _ _ _ _ _ _ w2056 _ _ _ _ w2200 w2237 w2267 w2299 _ _ _ _ w2410 w2459 w2493 w2525 _ _ _ _ w2630 w2687 _ _ _ _ _ _ _ _ _ _ _ _ _ _ _ _ _ _ _ _ _ _ _ _ _ _ _ _ _]
            tunnel: [_ _ _ _ _ _ _ _ _ _ _ _ _ _ _ _ _ _ _ _ w2056 _ _ _ w2170 w2200 w2237 w2267 w2299 _ _ _ _ w2410 w2459 w2493 w2525 _ _ _ _ w2630 w2687 _ _ _ _ _ _ _ _ _ _ _ _ _ _ _ _ _ _ _ _ _ _ _ _ _ _ _ _ _] -> w1059
            tunnel: w1054 -> [_ _ _ _ _ _ _ _ _ _ _ _ _ _ _ _ _ _ _ _ _ _ _ _ _ _ _ _ _ _ _ _ _ _ _ _ _ _ _ _ _ _ _ _ _ _ _ _ _ _ _ _ _ _ _ _ _ _ _ _ _ _ _ _ _ _ _ _ _ _ w3411 w3444]
            tunnel: [_ _ _ _ _ _ _ _ _ _ _ _ _ _ _ _ _ _ _ _ _ _ _ _ _ _ _ _ _ _ _ _ _ _ _ _ _ _ _ _ _ _ _ _ _ _ _ _ _ _ _ _ _ _ _ _ _ _ _ _ _ _ _ _ _ _ _ _ _ _ w3409 w3442] -> w1053
            tunnel: w1049 -> [_ _ _ _ _ _ _ _ _ _ _ _ _ _ _ _ _ _ _ _ w2055 w2089 w2114 w2147 w2169 w2199 w2236 w2266 w2298 _ _ _ _ w2409 w2458 w2492 w2524 _ _ _ _ _ _ _ _ _ _ _ _ _ _ _ _ _ _ _ _ _ _ _ _ _ _ _ _ _ _ _ _ _ _ _]
            tunnel: [_ _ _ _ _ _ _ _ _ _ _ _ _ _ _ _ _ _ _ w2026 w2055 w2089 w2113 w2146 w2169 w2199 w2236 w2266 w2298 _ _ _ _ w2409 w2458 w2492 w2524 _ _ _ _ _ _ _ _ _ _ _ _ _ _ _ _ _ _ _ _ _ _ _ _ _ _ _ _ _ _ _ _ _ _ _] -> w1048
            tunnel: [_ _ _ _ _ _ _ _ _ _ _ _ _ _ _ _ _ _ _ _ _ _ _ _ _ _ _ _ _ _ _ _ _ _ w2455 _ _ _ _ _ _ _ _ _ _ _ _ _ _ _ _ _ _ _ _ _ _ _ _ _ _ _ _ _ _ _ _ _ _ _ _ _] -> w1043
            tunnel: [_ _ _ _ _ _ _ _ _ _ _ _ _ _ _ _ _ _ _ _ _ _ _ _ _ _ _ _ _ _ _ _ _ _ w2454 _ _ _ _ _ _ _ _ _ _ _ _ _ _ _ _ _ _ _ _ _ _ _ _ _ _ _ _ _ _ _ _ _ _ _ _ _] -> w1042
            tunnel: [_ _ _ _ _ _ _ _ _ _ _ _ _ _ _ _ _ _ _ _ _ _ _ _ _ _ _ _ _ _ _ _ _ _ w2453 _ _ _ _ _ _ _ _ _ _ _ _ _ _ _ _ _ _ _ _ _ _ _ _ _ _ _ _ _ _ _ _ _ _ _ _ _] -> w1041
            tunnel: [_ _ _ _ _ _ _ _ _ _ _ _ _ _ _ _ _ _ _ _ _ _ _ _ _ _ _ _ _ _ _ _ _ _ w2453 _ _ _ _ _ _ _ _ _ _ _ _ _ _ _ _ _ _ _ _ _ _ _ _ _ _ _ _ _ _ _ _ _ _ _ _ _] -> _
            frame "Start1", Default {
              w1184 = FALSE ("SelectionState")
              n600 = xnode "Read/Write Control"("FPGA VI Reference In"=w1186, "error in"=w1185, "SelectionState"=w1184, "LR_reward_Laser_l1"=w1184, "LR_wrong_Laser_l1"=w1184, "LR_reward_Event_l1"=w1184, "LR_wrong_Event_l1"=w1184, "Left(F)_or_Right(T)"=w1184, "ignoreWrong"=w1184, "SelectionState"=w1184, "LR_reward_Laser_l2"=w1184, "LR_wrong_laser_l2"=w1184, "LR_reward_Event_l2"=w1184, "LR_wrong_Event_l2"=w1184, "LC_Event_l1"=w1184, "LC_Laser_l1"=w1184, "LC_Laser_l2"=w1184, "LC_Event_l2"=w1184, "CueLed_Event"=w1184) -> ()  [unwired: 2 out]
            }
            frame "Start2" {
            }
            frame "Start3" {
            }
            frame "saveSettings1" {
              n601 = call "myRIO_BRig_RT_dataExp_Audio_freq__L.vi"() -> ("output_Audio_freq__L"=w1273:i32)  [unwired: 11 in]
              n602 = call "myRIO_BRig_RT_dataExp_Audio_freq__R.vi"() -> ("output_Audio_freq__R"=w1272:i32)  [unwired: 11 in]
              n603 = call "myRIO_BRig_RT_dataExp_Audio_amp__L.vi"() -> ("output_Audio_amp__L"=w1271:i32)  [unwired: 11 in]
              n604 = call "myRIO_BRig_RT_dataExp_Audio_amp__R.vi"() -> ("output_Audio_amp__R"=w1269:i32)  [unwired: 11 in]
              n605 = call "myRIO_BRig_RT_dataExp_TPB_min__L.vi"() -> ("output_TPB_min__L"=w1281:i32)  [unwired: 11 in]
              n606 = call "myRIO_BRig_RT_dataExp_TPB_min__R.vi"() -> ("output_TPB_min__R"=w1279:i32)  [unwired: 11 in]
              n607 = call "myRIO_BRig_RT_dataExp_TPB_max__L.vi"() -> ("output_TPB_max__L"=w1277:i32)  [unwired: 11 in]
              n608 = call "myRIO_BRig_RT_dataExp_TPB_max__R.vi"() -> ("output_TPB_max__R"=w1275:i32)  [unwired: 11 in]
              n609 = call "myRIO_BRig_RT_dataExp_ItrialUntilReward.vi"() -> ("output_I_trialUntilReward"=w1294:i32)  [unwired: 11 in]
              n610 = call "myRIO_BRig_RT_dataExp_IblockUntilReward.vi"() -> ("output_I_blockUntilReward"=w1290:i32)  [unwired: 11 in]
              n611 = call "myRIO_BRig_RT_dataExp_CueCycles.vi"() -> ("output_CueCycles"=w1289:i32)  [unwired: 11 in]
              n612 = call "myRIO_BRig_RT_dataExp_ENL_min.vi"() -> ("output_ENL_min"=w1287:i32)  [unwired: 11 in]
              n613 = call "myRIO_BRig_RT_dataExp_ENL_max.vi"() -> ("output_ENL_max"=w1285:i32)  [unwired: 11 in]
              n614 = call "myRIO_BRig_RT_dataExp_ENL_penalty.vi"() -> ("output_ENL_penalty"=w1283:i32)  [unwired: 11 in]
              n615 = local read "Audio_Freq__L"() -> (w1247:u8)
              n616 = local read "Audio_Freq__R"() -> (w1245:u8)
              n617 = local read "Audio_Amp__L"() -> (w1270:u16)
              n618 = local read "TpB_Min_L"() -> (w1280:u16)
              n619 = local read "TpB_Min_R"() -> (w1278:u16)
              n620 = local read "TpB_Max_L"() -> (w1276:u16)
              n621 = local read "TpB_Max_R"() -> (w1274:u16)
              n622 = local read "Audio_Amp__R"() -> (w1268:u16)
              n623 = local read "TrialUntilReward"() -> (w1293:bool)
              n624 = local read "CueCycles"() -> (w1288:u16)
              n625 = local read "Tcycle_ENL_min"() -> (w1286:u16)
              n626 = local read "Tcycle_ENL_max"() -> (w1284:u16)
              n627 = local read "Tcycle_ENLPenalty"() -> (w1282:u16)
              n628 = To Unsigned Word Integer(number=w1245) -> (unsigned 16bit integer=w1244:u16)
              n629 = To Unsigned Word Integer(number=w1247) -> (unsigned 16bit integer=w1246:u16)
              n630 = Boolean To (0,1)(Boolean=w1293) -> (0, 1=w1292:i16)
              n631 = To Unsigned Word Integer(number=w1292) -> (unsigned 16bit integer=w1291:u16)
              n632 = local read "BUR_min"() -> (w1262:u16)
              n633 = local read "BUR_max"() -> (w1263:u16)
              n634 = Not Equal To 0?(x=w1262) -> (x != 0?=w1261:bool)
              n635 = Not Equal To 0?(x=w1263) -> (x != 0?=w1260:bool)
              n636 = And(x=w1261, y=w1260) -> (x .and. y?=w1259:bool)
              n637 = Boolean To (0,1)(Boolean=w1259) -> (0, 1=w1264:i16)
              n638 = To Unsigned Word Integer(number=w1264) -> (unsigned 16bit integer=w1258:u16)
              n639 = Replace Array Subset(array=w1296, new element #1=w1291, index #1=w1294, new element #2=w1258, index #2=w1290, new element #3=w1288, index #3=w1289, new element #4=w1286, index #4=w1287, new element #5=w1284, index #5=w1285, new element #6=w1282, index #6=w1283, new element #7=w1280, index #7=w1281, new element #8=w1278, index #8=w1279, new element #9=w1276, index #9=w1277, new element #10=w1274, index #10=w1275, new element #11=w1246, index #11=w1273, new element #12=w1244, index #12=w1272, new element #13=w1270, index #13=w1271, new element #14=w1268, index #14=w1269) -> (w1295:u16[])
            }
            frame "saveSettings2" {
              n640 = call "myRIO_BRig_RT_dataExp_Tcycle_RewardPost.vi"() -> ("output_Tcycle_RewardPost"=w1333:i32)  [unwired: 11 in]
              n641 = call "myRIO_BRig_RT_dataExp_Tcycle_Wrong.vi"() -> ("output_Tcycle_Wrong"=w1331:i32)  [unwired: 11 in]
              n642 = call "myRIO_BRig_RT_dataExp_Tcycle_Timeout.vi"() -> ("output_Tcycle_Timeout"=w1329:i32)  [unwired: 11 in]
              n643 = call "myRIO_BRig_RT_dataExp_Tcycle_Cue_min.vi"() -> ("output_Tcycle_Cue_min"=w1327:i32)  [unwired: 11 in]
              n644 = call "myRIO_BRig_RT_dataExp_Tcycle_Cue_max.vi"() -> ("output_Tcycle_Cue_max"=w1326:i32)  [unwired: 11 in]
              n645 = call "myRIO_BRig_RT_dataExp_Tcycle_CuePenalty.vi"() -> ("output_Tcycle_CuePenalty"=w1325:i32)  [unwired: 11 in]
              n646 = call "myRIO_BRig_RT_dataExp_SolenoidProbability_L.vi"() -> ("output_SolenoidProbability_L"=w1305:i32)  [unwired: 11 in]
              n647 = call "myRIO_BRig_RT_dataExp_SolenoidProbability_R.vi"() -> ("output_SolenoidProbability_R"=w1304:i32)  [unwired: 11 in]
              n648 = call "myRIO_BRig_RT_dataExp_nBlock.vi"() -> ("output_nBlock"=w1342:i32)  [unwired: 11 in]
              n649 = call "myRIO_BRig_RT_dataExp_nTrial.vi"() -> ("output_nTrial"=w1341:i32)  [unwired: 11 in]
              n650 = call "myRIO_BRig_RT_dataExp_runTime_seconds.vi"() -> ("output_RunTime_minutes"=w1340:i32)  [unwired: 11 in]
              n651 = call "myRIO_BRig_RT_dataExp_Tcycle_Selection.vi"() -> ("output_Tcycle_Selection"=w1339:i32)  [unwired: 11 in]
              n652 = call "myRIO_BRig_RT_dataExp_Tcycle_Reward__L.vi"() -> ("output_Tcycle_Reward__L"=w1337:i32)  [unwired: 11 in]
              n653 = call "myRIO_BRig_RT_dataExp_Tcycle_Reward__R.vi"() -> ("output_Tcycle_Reward__R"=w1335:i32)  [unwired: 11 in]
              n654 = local read "Tcycle_RewardPost"() -> (w1332:u16)
              n655 = local read "Tcycle_Wrong"() -> (w1330:u16)
              n656 = local read "Tcycle_Timeout"() -> (w1328:u16)
              n657 = local read "Tcycle_CuePenalty"() -> (w1318:u16)
              n658 = local read "Tcycle_Cue_max"() -> (w1306:u16)
              n659 = local read "Tcycle_Cue_min"() -> (w1307:u16)
              n660 = local read "Tcycle_Selection"() -> (w1338:u16)
              n661 = local read "Tcycle_Reward_L"() -> (w1336:u16)
              n662 = local read "Tcycle_Reward_R"() -> (w1334:u16)
              n663 = local read "SolenoidProbability_R"() -> (w1302:u16)
              n664 = local read "SolenoidProbability_L"() -> (w1303:u16)
              n665 = Replace Array Subset(array=w1344, new element #1=u16 0, index #1=w1342, new element #2=u16 0, index #2=w1341, new element #3=u16 0, index #3=w1340, new element #4=w1338, index #4=w1339, new element #5=w1336, index #5=w1337, new element #6=w1334, index #6=w1335, new element #7=w1332, index #7=w1333, new element #8=w1330, index #8=w1331, new element #9=w1328, index #9=w1329, new element #10=w1307, index #10=w1327, new element #11=w1306, index #11=w1326, new element #12=w1318, index #12=w1325, new element #13=w1303, index #13=w1305, new element #14=w1302, index #14=w1304) -> (w1343:u16[])
            }
            frame "saveSettings3" {
              w1355 = 100.0 ("y")
              n666 = call "myRIO_BRig_RT_dataExp_laser1_Freq.vi"() -> ("output_laser1_Freq"=w1388:i32)  [unwired: 11 in]
              n667 = call "myRIO_BRig_RT_dataExp_laser1_Tpeak.vi"() -> ("output_laser1_Tpeak"=w1383:i32)  [unwired: 11 in]
              n668 = call "myRIO_BRig_RT_dataExp_laser1_Tshutter.vi"() -> ("output_laser1_Tshutter"=w1378:i32)  [unwired: 11 in]
              n669 = call "myRIO_BRig_RT_dataExp_FPGA_f_count2ms.vi"() -> ("output_FPGA_f_count2ms"=w1373:i32)  [unwired: 11 in]
              n670 = call "myRIO_BRig_RT_dataExp_laser1_Power_min.vi"() -> ("output_laser1_Power_min"=w1368:i32)  [unwired: 11 in]
              n671 = call "myRIO_BRig_RT_dataExp_laser1_Power_max.vi"() -> ("output_laser1_Power_max"=w1361:i32)  [unwired: 11 in]
              n672 = call "myRIO_BRig_RT_dataExp_laser1_Power_step.vi"() -> ("output_laser1_Power_step"=w1360:i32)  [unwired: 11 in]
              n673 = call "myRIO_BRig_RT_dataExp_laser1_duration.vi"() -> ("output_laser1_duration"=w1363:i32)  [unwired: 11 in]
              n674 = local read "Laser_Tshutter_l1"() -> (w1375:dbl)
              n675 = local read "Laser_Tpeak_l1"() -> (w1380:dbl)
              n676 = local read "Laser_power_max_l1"() -> (w1354:dbl)
              n677 = local read "Laser_power_step_l1"() -> (w1353:dbl)
              n678 = local read "Laser_power_min_l1"() -> (w1365:dbl)
              n679 = local read "Laser_Freq_l1"() -> (w1387:dbl)
              n680 = call "myRIO_BRig_RT_dataExp_BUR_min.vi"() -> ("output_BUR_min"=w1410:i32)  [unwired: 11 in]
              n681 = call "myRIO_BRig_RT_dataExp_BUR_max.vi"() -> ("output_BUR_max"=w1408:i32)  [unwired: 11 in]
              n682 = call "myRIO_BRig_RT_dataExp_Audio_sp__L.vi"() -> ("output_Audio_sp__L"=w1405:i32)  [unwired: 11 in]
              n683 = call "myRIO_BRig_RT_dataExp_Audio_sp__R.vi"() -> ("output_Audio_sp__R"=w1404:i32)  [unwired: 11 in]
              n684 = local read "FPGA_count2ms"() -> (w1370:dbl)
              n685 = local read "sp_LeftSpout"() -> (w1403:u16)
              n686 = local read "BUR_max"() -> (w1407:u16)
              n687 = local read "sp_RightSpout"() -> (w1402:u16)
              n688 = local read "BUR_min"() -> (w1409:u16)
              n689 = Multiply(x=w1387, y=w1355) -> (x*y=w1386:dbl)
              n690 = Multiply(x=w1380, y=w1355) -> (x*y=w1382:dbl)
              n691 = Multiply(x=w1375, y=w1355) -> (x*y=w1377:dbl)
              n692 = Multiply(x=w1370, y=w1355) -> (x*y=w1372:dbl)
              n693 = Multiply(x=w1365, y=w1355) -> (x*y=w1367:dbl)
              n694 = Multiply(x=w1354, y=w1355) -> (x*y=w1359:dbl)
              n695 = Multiply(x=w1353, y=w1355) -> (x*y=w1357:dbl)
              n696 = Round To Nearest(number=w1386) -> (nearest integer value=w1385:dbl)
              n697 = Round To Nearest(number=w1382) -> (nearest integer value=w1381:dbl)
              n698 = Round To Nearest(number=w1377) -> (nearest integer value=w1376:dbl)
              n699 = Round To Nearest(number=w1372) -> (nearest integer value=w1371:dbl)
              n700 = Round To Nearest(number=w1367) -> (nearest integer value=w1366:dbl)
              n701 = Round To Nearest(number=w1359) -> (nearest integer value=w1358:dbl)
              n702 = Round To Nearest(number=w1357) -> (nearest integer value=w1356:dbl)
              n703 = To Unsigned Word Integer(number=w1385) -> (unsigned 16bit integer=w1384:u16)
              n704 = To Unsigned Word Integer(number=w1381) -> (unsigned 16bit integer=w1379:u16)
              n705 = To Unsigned Word Integer(number=w1376) -> (unsigned 16bit integer=w1374:u16)
              n706 = To Unsigned Word Integer(number=w1371) -> (unsigned 16bit integer=w1369:u16)
              n707 = To Unsigned Word Integer(number=w1366) -> (unsigned 16bit integer=w1364:u16)
              n708 = To Unsigned Word Integer(number=w1358) -> (unsigned 16bit integer=w1352:u16)
              n709 = To Unsigned Word Integer(number=w1356) -> (unsigned 16bit integer=w1351:u16)
              n710 = local read "Laser_duration_l1"() -> (w1362:u16)
              n711 = call "myRIO_BRig_RT_dataCurrent_laser1_pulse_duration.vi"() -> ("output_laser1_pulse_duration"=w1389:i32)  [unwired: 11 in]
              n712 = Replace Array Subset(array=w1411, new element #1=w1409, index #1=w1410, new element #2=w1407, index #2=w1408, new element #3=w1403, index #3=w1405, new element #4=w1402, index #4=w1404, new element #5=w1384, index #5=w1388, new element #6=w1379, index #6=w1383, new element #7=w1374, index #7=w1378, new element #8=w1369, index #8=w1373, new element #9=w1364, index #9=w1368, new element #10=w1352, index #10=w1361, new element #11=w1351, index #11=w1360, new element #12=w1362, index #12=w1363) -> (w1406:u16[])
              n713 = Replace Array Subset(array=w1391, new element=w1362, index=w1389) -> (w1390:u16[])
            }
            frame "saveSettings4" {
              w1432 = 100.0 ("y")
              n714 = call "myRIO_BRig_RT_dataExp_laser2_Freq.vi"() -> ("output_laser2_Freq"=w1419:i32)  [unwired: 11 in]
              n715 = call "myRIO_BRig_RT_dataExp_laser2_Tpeak.vi"() -> ("output_laser2_Tpeak"=w1421:i32)  [unwired: 11 in]
              n716 = call "myRIO_BRig_RT_dataExp_laser2_Tshutter.vi"() -> ("output_laser2_Tshutter"=w1423:i32)  [unwired: 11 in]
              n717 = call "myRIO_BRig_RT_dataExp_laser2_Power_min.vi"() -> ("output_laser2_Power_min"=w1440:i32)  [unwired: 11 in]
              n718 = call "myRIO_BRig_RT_dataExp_laser2_Power_max.vi"() -> ("output_laser2_Power_max"=w1439:i32)  [unwired: 11 in]
              n719 = call "myRIO_BRig_RT_dataExp_laser2_Power_step.vi"() -> ("output_laser2_Power_step"=w1438:i32)  [unwired: 11 in]
              n720 = call "myRIO_BRig_RT_dataExp_laser2_duration.vi"() -> ("output_laser2_duration"=w1437:i32)  [unwired: 11 in]
              n721 = call "myRIO_BRig_RT_dataExp_CueLed_Freq.vi"() -> ("output_CueLed_Freq"=w1429:i32)  [unwired: 11 in]
              n722 = call "myRIO_BRig_RT_dataExp_CueLed_Tpeak.vi"() -> ("output_CueLed_Tpeak"=w1428:i32)  [unwired: 11 in]
              n723 = call "myRIO_BRig_RT_dataExp_CueLed_duration.vi"() -> ("output_CueLed_duration"=w1425:i32)  [unwired: 11 in]
              n724 = local read "Laser_Tshutter_l2"() -> (w1456:dbl)
              n725 = local read "Laser_Tpeak_l2"() -> (w1459:dbl)
              n726 = local read "Laser_power_max_l2"() -> (w1446:dbl)
              n727 = local read "Laser_power_step_l2"() -> (w1445:dbl)
              n728 = local read "Laser_power_min_l2"() -> (w1453:dbl)
              n729 = local read "Laser_Freq_l2"() -> (w1464:dbl)
              n730 = local read "CueLed_Tpeak"() -> (w1430:dbl)
              n731 = local read "CueLed_duration"() -> (w1424:u16)
              n732 = local read "CueLed_Freq"() -> (w1431:dbl)
              n733 = Multiply(x=w1464, y=w1432) -> (x*y=w1463:dbl)
              n734 = Multiply(x=w1459, y=w1432) -> (x*y=w1461:dbl)
              n735 = Multiply(x=w1456, y=w1432) -> (x*y=w1458:dbl)
              n736 = Multiply(x=w1453, y=w1432) -> (x*y=w1455:dbl)
              n737 = Multiply(x=w1446, y=w1432) -> (x*y=w1450:dbl)
              n738 = Multiply(x=w1445, y=w1432) -> (x*y=w1448:dbl)
              n739 = Multiply(x=w1431, y=w1432) -> (x*y=w1433:dbl)
              n740 = Multiply(x=w1430, y=w1432) -> (x*y=w1434:dbl)
              n741 = Round To Nearest(number=w1463) -> (nearest integer value=w1462:dbl)
              n742 = Round To Nearest(number=w1461) -> (nearest integer value=w1460:dbl)
              n743 = Round To Nearest(number=w1458) -> (nearest integer value=w1457:dbl)
              n744 = Round To Nearest(number=w1455) -> (nearest integer value=w1454:dbl)
              n745 = Round To Nearest(number=w1450) -> (nearest integer value=w1449:dbl)
              n746 = Round To Nearest(number=w1448) -> (nearest integer value=w1447:dbl)
              n747 = Round To Nearest(number=w1433) -> (nearest integer value=w1436:dbl)
              n748 = Round To Nearest(number=w1434) -> (nearest integer value=w1435:dbl)
              n749 = To Unsigned Word Integer(number=w1462) -> (unsigned 16bit integer=w1418:u16)
              n750 = To Unsigned Word Integer(number=w1460) -> (unsigned 16bit integer=w1420:u16)
              n751 = To Unsigned Word Integer(number=w1457) -> (unsigned 16bit integer=w1422:u16)
              n752 = To Unsigned Word Integer(number=w1454) -> (unsigned 16bit integer=w1452:u16)
              n753 = To Unsigned Word Integer(number=w1449) -> (unsigned 16bit integer=w1444:u16)
              n754 = To Unsigned Word Integer(number=w1447) -> (unsigned 16bit integer=w1443:u16)
              n755 = To Unsigned Word Integer(number=w1436) -> (unsigned 16bit integer=w1427:u16)
              n756 = To Unsigned Word Integer(number=w1435) -> (unsigned 16bit integer=w1426:u16)
              n757 = local read "Laser_duration_l2"() -> (w1451:u16)
              n758 = call "myRIO_BRig_RT_dataCurrent_laser2_pulse_duration.vi"() -> ("output_laser2_pulse_duration"=w1441:i32)  [unwired: 11 in]
              n759 = Replace Array Subset(array=w1466, new element=w1451, index=w1441) -> (w1465:u16[])
              n760 = Replace Array Subset(array=w1478, new element #1=w1418, index #1=w1419, new element #2=w1420, index #2=w1421, new element #3=w1422, index #3=w1423, new element #4=w1452, index #4=w1440, new element #5=w1444, index #5=w1439, new element #6=w1443, index #6=w1438, new element #7=w1451, index #7=w1437, new element #8=w1427, index #8=w1429, new element #9=w1426, index #9=w1428, new element #10=w1424, index #10=w1425) -> (w1477:u16[])
            }
            frame "saveSettings_LC_ENL_l1" {
              # "Selection First"
              # "Count"
              # "Tdelay"
              # "Probability"
              # "OnOff"
              # "Block"
              # "delayOpt"
              # "Count"
              # "Tdelay"
              # "Probability"
              # "OnOff"
              # "Block"
              # "ENL1 All"
              # "delayOpt"
              # "Count"
              # "Tdelay"
              # "Probability"
              # "OnOff"
              # "Block"
              # "ENL1 First"
              n761 = local read "LC_ENL1_delayOpt_Switch_l1"() -> (w1516:bool)
              n762 = call "myRIO_BRig_RT_dataLC_ENL1_Block_NS_l1.vi"() -> ("output_ENL1_All_Block"=w1513:i32)  [unwired: 11 in]
              n763 = call "myRIO_BRig_RT_dataLC_ENL1_OnOff_NS_l1.vi"() -> ("output_ENL1_OnOff_NS_l1"=w1503:i32)  [unwired: 11 in]
              n764 = call "myRIO_BRig_RT_dataLC_ENL1_Probability_NS_l1.vi"() -> ("output_ENL1_Probability_NS_l1"=w1502:i32)  [unwired: 11 in]
              n765 = call "myRIO_BRig_RT_dataLC_ENL1_Tdelay_NS_l1.vi"() -> ("output_ENL1_Tdelay_NS_l1"=w1501:i32)  [unwired: 11 in]
              n766 = call "myRIO_BRig_RT_dataLC_ENL1_Count_NS_l1.vi"() -> ("output_ENL1_Count_NS_l1"=w1500:i32)  [unwired: 11 in]
              n767 = call "myRIO_BRig_RT_dataLC_ENL1_delayOpt_NS_l1.vi"() -> ("output_ENL1_delayOpt_NS_l1"=w1499:i32)  [unwired: 11 in]
              n768 = call "myRIO_BRig_RT_dataLC_ENL1_Block_Switch_l1.vi"() -> ("output_ENL1_Block_Switch_l1"=w1539:i32)  [unwired: 11 in]
              n769 = call "myRIO_BRig_RT_dataLC_ENL1_OnOff_Switch_l1.vi"() -> ("output_ENL1_OnOff_Switch_l1"=w1537:i32)  [unwired: 11 in]
              n770 = call "myRIO_BRig_RT_dataLC_ENL1_Probability_Switch_l1.vi"() -> ("output_ENL1_Probability_Switch_l1"=w1533:i32)  [unwired: 11 in]
              n771 = call "myRIO_BRig_RT_dataLC_ENL1_Tdelay_Switch_l1.vi"() -> ("output_ENL1_Tdelay_Switch_l1"=w1531:i32)  [unwired: 11 in]
              n772 = call "myRIO_BRig_RT_dataLC_ENL1_Count_Switch_l1.vi"() -> ("output_ENL1_Count_Switch_l1"=w1529:i32)  [unwired: 11 in]
              n773 = call "myRIO_BRig_RT_dataLC_ENL1_delayOpt_Switch_l1.vi"() -> ("output_ENL1_delayOpt_Switch_l1"=w1515:i32)  [unwired: 11 in]
              n774 = local read "LC_ENL1_Count_Switch_l1"() -> (w1528:u16)
              n775 = local read "LC_ENL1_Probability_Switch_l1"() -> (w1532:u16)
              n776 = local read "LC_ENL1_Block_Switch_l1"() -> (w1538:u16)
              n777 = local read "LC_ENL1_Tdelay_Switch_l1"() -> (w1530:u16)
              n778 = local read "LC_ENL1_OnOff_Switch_l1"() -> (w1536:bool)
              n779 = call "myRIO_BRig_RT_dataLC_Selection_Block_Switch_l1.vi"() -> ("output_Selection_Block_Switch_l1"=w1497:i32)  [unwired: 11 in]
              n780 = call "myRIO_BRig_RT_dataLC_Selection_OnOff_Switch_l1.vi"() -> ("output_Selection_OnOff_Switch_l1"=w1496:i32)  [unwired: 11 in]
              n781 = call "myRIO_BRig_RT_dataLC_Selection_Probability_Switch_l1.vi"() -> ("output_Selection_Probability_Switch_l1"=w1495:i32)  [unwired: 11 in]
              n782 = call "myRIO_BRig_RT_dataLC_Selection_Tdelay_Switch_l1.vi"() -> ("output_Selection_Tdelay_Switch_l1"=w1494:i32)  [unwired: 11 in]
              n783 = call "myRIO_BRig_RT_dataLC_Selection_Count_Switch_l1.vi"() -> ("output_Selection_Count_Switch_l1"=w1493:i32)  [unwired: 11 in]
              n784 = local read "LC_ENL1_OnOff_NS_l1"() -> (w1509:bool)
              n785 = local read "LC_ENL1_Probability_NS_l1"() -> (w1507:u16)
              n786 = local read "LC_ENL1_delayOpt_NS_l1"() -> (w1505:bool)
              n787 = local read "LC_Sel_Probability_Switch_l1"() -> (w1488:u16)
              n788 = local read "LC_ENL1_Tdelay_NS_l1"() -> (w1498:u16)
              n789 = local read "LC_ENL1_Block_NS_l1"() -> (w1510:u16)
              n790 = local read "LC_ENL1_Count_NS_l1"() -> (w1506:u16)
              n791 = local read "LC_Sel_Tdelay_Switch_l1"() -> (w1487:u16)
              n792 = local read "LC_Sel_OnOff_Switch_l1"() -> (w1491:bool)
              n793 = local read "LC_Sel_Count_Switch_l1"() -> (w1486:u16)
              n794 = local read "LC_Sel_Block_Switch_l1"() -> (w1490:u16)
              n795 = Boolean To (0,1)(Boolean=w1516) -> (0, 1=w1517:i16)
              n796 = Boolean To (0,1)(Boolean=w1536) -> (0, 1=w1535:i16)
              n797 = Boolean To (0,1)(Boolean=w1509) -> (0, 1=w1512:i16)
              n798 = To Unsigned Word Integer(number=w1517) -> (unsigned 16bit integer=w1514:u16)
              n799 = To Unsigned Word Integer(number=w1535) -> (unsigned 16bit integer=w1534:u16)
              n800 = Boolean To (0,1)(Boolean=w1505) -> (0, 1=w1511:i16)
              n801 = To Unsigned Word Integer(number=w1512) -> (unsigned 16bit integer=w1508:u16)
              n802 = Boolean To (0,1)(Boolean=w1491) -> (0, 1=w1492:i16)
              n803 = To Unsigned Word Integer(number=w1511) -> (unsigned 16bit integer=w1504:u16)
              n804 = To Unsigned Word Integer(number=w1492) -> (unsigned 16bit integer=w1489:u16)
              n805 = Replace Array Subset(array=w1540, new element #1=w1538, index #1=w1539, new element #2=w1534, index #2=w1537, new element #3=w1532, index #3=w1533, new element #4=w1530, index #4=w1531, new element #5=w1528, index #5=w1529, new element #6=w1514, index #6=w1515, new element #7=w1510, index #7=w1513, new element #8=w1508, index #8=w1503, new element #9=w1507, index #9=w1502, new element #10=w1498, index #10=w1501, new element #11=w1506, index #11=w1500, new element #12=w1504, index #12=w1499, new element #13=w1490, index #13=w1497, new element #14=w1489, index #14=w1496, new element #15=w1488, index #15=w1495, new element #16=w1487, index #16=w1494, new element #17=w1486, index #17=w1493) -> (w1541:u16[])
            }
            frame "saveSettings_LC_ENL_l2" {
              # "Selection First"
              # "Count"
              # "Tdelay"
              # "Probability"
              # "OnOff"
              # "Block"
              # "delayOpt"
              # "Count"
              # "Tdelay"
              # "Probability"
              # "OnOff"
              # "Block"
              # "ENL1 All"
              # "delayOpt"
              # "Count"
              # "Tdelay"
              # "Probability"
              # "OnOff"
              # "Block"
              # "ENL1 First"
              n806 = local read "LC_ENL1_delayOpt_Switch_l1"() -> (w1580:bool)
              n807 = call "myRIO_BRig_RT_dataLC_ENL1_Block_NS_l1.vi"() -> ("output_ENL1_All_Block"=w1577:i32)  [unwired: 11 in]
              n808 = call "myRIO_BRig_RT_dataLC_ENL1_OnOff_NS_l1.vi"() -> ("output_ENL1_OnOff_NS_l1"=w1567:i32)  [unwired: 11 in]
              n809 = call "myRIO_BRig_RT_dataLC_ENL1_Probability_NS_l1.vi"() -> ("output_ENL1_Probability_NS_l1"=w1566:i32)  [unwired: 11 in]
              n810 = call "myRIO_BRig_RT_dataLC_ENL1_Tdelay_NS_l1.vi"() -> ("output_ENL1_Tdelay_NS_l1"=w1565:i32)  [unwired: 11 in]
              n811 = call "myRIO_BRig_RT_dataLC_ENL1_Count_NS_l1.vi"() -> ("output_ENL1_Count_NS_l1"=w1564:i32)  [unwired: 11 in]
              n812 = call "myRIO_BRig_RT_dataLC_ENL1_delayOpt_NS_l1.vi"() -> ("output_ENL1_delayOpt_NS_l1"=w1563:i32)  [unwired: 11 in]
              n813 = call "myRIO_BRig_RT_dataLC_ENL1_Block_Switch_l1.vi"() -> ("output_ENL1_Block_Switch_l1"=w1603:i32)  [unwired: 11 in]
              n814 = call "myRIO_BRig_RT_dataLC_ENL1_OnOff_Switch_l1.vi"() -> ("output_ENL1_OnOff_Switch_l1"=w1601:i32)  [unwired: 11 in]
              n815 = call "myRIO_BRig_RT_dataLC_ENL1_Probability_Switch_l1.vi"() -> ("output_ENL1_Probability_Switch_l1"=w1597:i32)  [unwired: 11 in]
              n816 = call "myRIO_BRig_RT_dataLC_ENL1_Tdelay_Switch_l1.vi"() -> ("output_ENL1_Tdelay_Switch_l1"=w1595:i32)  [unwired: 11 in]
              n817 = call "myRIO_BRig_RT_dataLC_ENL1_Count_Switch_l1.vi"() -> ("output_ENL1_Count_Switch_l1"=w1593:i32)  [unwired: 11 in]
              n818 = call "myRIO_BRig_RT_dataLC_ENL1_delayOpt_Switch_l1.vi"() -> ("output_ENL1_delayOpt_Switch_l1"=w1579:i32)  [unwired: 11 in]
              n819 = local read "LC_ENL1_Count_Switch_l1"() -> (w1592:u16)
              n820 = local read "LC_ENL1_Probability_Switch_l1"() -> (w1596:u16)
              n821 = local read "LC_ENL1_Block_Switch_l1"() -> (w1602:u16)
              n822 = local read "LC_ENL1_Tdelay_Switch_l1"() -> (w1594:u16)
              n823 = local read "LC_ENL1_OnOff_Switch_l1"() -> (w1600:bool)
              n824 = call "myRIO_BRig_RT_dataLC_Selection_Block_Switch_l1.vi"() -> ("output_Selection_Block_Switch_l1"=w1561:i32)  [unwired: 11 in]
              n825 = call "myRIO_BRig_RT_dataLC_Selection_OnOff_Switch_l1.vi"() -> ("output_Selection_OnOff_Switch_l1"=w1560:i32)  [unwired: 11 in]
              n826 = call "myRIO_BRig_RT_dataLC_Selection_Probability_Switch_l1.vi"() -> ("output_Selection_Probability_Switch_l1"=w1559:i32)  [unwired: 11 in]
              n827 = call "myRIO_BRig_RT_dataLC_Selection_Tdelay_Switch_l1.vi"() -> ("output_Selection_Tdelay_Switch_l1"=w1558:i32)  [unwired: 11 in]
              n828 = call "myRIO_BRig_RT_dataLC_Selection_Count_Switch_l1.vi"() -> ("output_Selection_Count_Switch_l1"=w1557:i32)  [unwired: 11 in]
              n829 = local read "LC_ENL1_OnOff_NS_l1"() -> (w1573:bool)
              n830 = local read "LC_ENL1_Probability_NS_l1"() -> (w1571:u16)
              n831 = local read "LC_ENL1_delayOpt_NS_l1"() -> (w1569:bool)
              n832 = local read "LC_Sel_Probability_Switch_l1"() -> (w1552:u16)
              n833 = local read "LC_ENL1_Tdelay_NS_l1"() -> (w1562:u16)
              n834 = local read "LC_ENL1_Block_NS_l1"() -> (w1574:u16)
              n835 = local read "LC_ENL1_Count_NS_l1"() -> (w1570:u16)
              n836 = local read "LC_Sel_Tdelay_Switch_l1"() -> (w1551:u16)
              n837 = local read "LC_Sel_OnOff_Switch_l1"() -> (w1555:bool)
              n838 = local read "LC_Sel_Count_Switch_l1"() -> (w1550:u16)
              n839 = local read "LC_Sel_Block_Switch_l1"() -> (w1554:u16)
              n840 = Boolean To (0,1)(Boolean=w1580) -> (0, 1=w1581:i16)
              n841 = Boolean To (0,1)(Boolean=w1600) -> (0, 1=w1599:i16)
              n842 = Boolean To (0,1)(Boolean=w1573) -> (0, 1=w1576:i16)
              n843 = To Unsigned Word Integer(number=w1581) -> (unsigned 16bit integer=w1578:u16)
              n844 = To Unsigned Word Integer(number=w1599) -> (unsigned 16bit integer=w1598:u16)
              n845 = Boolean To (0,1)(Boolean=w1569) -> (0, 1=w1575:i16)
              n846 = To Unsigned Word Integer(number=w1576) -> (unsigned 16bit integer=w1572:u16)
              n847 = Boolean To (0,1)(Boolean=w1555) -> (0, 1=w1556:i16)
              n848 = To Unsigned Word Integer(number=w1575) -> (unsigned 16bit integer=w1568:u16)
              n849 = To Unsigned Word Integer(number=w1556) -> (unsigned 16bit integer=w1553:u16)
              n850 = Replace Array Subset(array=w1604, new element #1=w1602, index #1=w1603, new element #2=w1598, index #2=w1601, new element #3=w1596, index #3=w1597, new element #4=w1594, index #4=w1595, new element #5=w1592, index #5=w1593, new element #6=w1578, index #6=w1579, new element #7=w1574, index #7=w1577, new element #8=w1572, index #8=w1567, new element #9=w1571, index #9=w1566, new element #10=w1562, index #10=w1565, new element #11=w1570, index #11=w1564, new element #12=w1568, index #12=w1563, new element #13=w1554, index #13=w1561, new element #14=w1553, index #14=w1560, new element #15=w1552, index #15=w1559, new element #16=w1551, index #16=w1558, new element #17=w1550, index #17=w1557) -> (w1605:u16[])
            }
            frame "saveSettings_LC_Cue_l1" {
              # "Selection All"
              # "Count"
              # "Tdelay"
              # "Probability"
              # "OnOff"
              # "Block"
              # "delayOpt"
              # "Count"
              # "Tdelay"
              # "Probability"
              # "OnOff"
              # "Block"
              # "Cue1 All"
              # "delayOpt"
              # "Count"
              # "Tdelay"
              # "Probability"
              # "OnOff"
              # "Block"
              # "Cue1 First"
              n851 = call "myRIO_BRig_RT_dataLC_Cue1_delayOpt_Switch_l1.vi"() -> ("output_Cue1_delayOpt_Switch_l1"=w1644:i32)  [unwired: 11 in]
              n852 = call "myRIO_BRig_RT_dataLC_Cue1_Block_Switch_l1.vi"() -> ("output_Cue1_Block_Switch_l1"=w1667:i32)  [unwired: 11 in]
              n853 = call "myRIO_BRig_RT_dataLC_Cue1_OnOff_Switch_l1.vi"() -> ("output_Cue1_OnOff_Switch_l1"=w1665:i32)  [unwired: 11 in]
              n854 = call "myRIO_BRig_RT_dataLC_Cue1_Probability_Switch_l1.vi"() -> ("output_Cue1_Probability_Switch_l1"=w1661:i32)  [unwired: 11 in]
              n855 = call "myRIO_BRig_RT_dataLC_Cue1_Tdelay_Switch_l1.vi"() -> ("output_Cue1_Tdelay_Switch_l1"=w1659:i32)  [unwired: 11 in]
              n856 = call "myRIO_BRig_RT_dataLC_Cue1_Count_Switch_l1.vi"() -> ("output_Cue1_Count_Switch_l1"=w1657:i32)  [unwired: 11 in]
              n857 = local read "LC_Cue1_delayOpt_Switch_l1"() -> (w1643:bool)
              n858 = call "myRIO_BRig_RT_dataLC_Cue1_Block_NS_l1.vi"() -> ("output_Cue1_Block_NS_l1"=w1641:i32)  [unwired: 11 in]
              n859 = call "myRIO_BRig_RT_dataLC_Cue1_OnOff_NS_l1.vi"() -> ("output_Cue1_OnOff_NS_l1"=w1640:i32)  [unwired: 11 in]
              n860 = call "myRIO_BRig_RT_dataLC_Cue1_Probability_NS_l1.vi"() -> ("output_Cue1_l1_All_Probability"=w1639:i32)  [unwired: 11 in]
              n861 = call "myRIO_BRig_RT_dataLC_Cue1_Tdelay_NS_l1.vi"() -> ("output_Cue1_Tdelay_NS_l1"=w1638:i32)  [unwired: 11 in]
              n862 = call "myRIO_BRig_RT_dataLC_Cue1_Count_NS_l1.vi"() -> ("output_Cue1_Count_NS_l1"=w1637:i32)  [unwired: 11 in]
              n863 = call "myRIO_BRig_RT_dataLC_Cue1_delayOpt_NS_l1.vi"() -> ("output_Cue1_delayOpt_NS_l1"=w1636:i32)  [unwired: 11 in]
              n864 = local read "LC_Cue1_Count_Switch_l1"() -> (w1656:u16)
              n865 = local read "LC_Cue1_Probability_Switch_l1"() -> (w1660:u16)
              n866 = local read "LC_Cue1_Block_Switch_l1"() -> (w1666:u16)
              n867 = local read "LC_Cue1_Tdelay_Switch_l1"() -> (w1658:u16)
              n868 = local read "LC_Cue1_OnOff_Switch_l1"() -> (w1664:bool)
              n869 = local read "LC_Cue1_OnOff_NS_l1"() -> (w1632:bool)
              n870 = call "myRIO_BRig_RT_dataLC_Selection_Block_NS_l1.vi"() -> ("output_Selection_Block_NS_l1"=w1625:i32)  [unwired: 11 in]
              n871 = call "myRIO_BRig_RT_dataLC_Selection_OnOff_NS_l1.vi"() -> ("output_Selection_OnOff_NS_l1"=w1624:i32)  [unwired: 11 in]
              n872 = call "myRIO_BRig_RT_dataLC_Selection_Probability_NS_l1.vi"() -> ("output_Selection_Probability_NS_l1"=w1623:i32)  [unwired: 11 in]
              n873 = call "myRIO_BRig_RT_dataLC_Selection_Tdelay_NS_l1.vi"() -> ("output_Selection_Tdelay_NS_l1"=w1622:i32)  [unwired: 11 in]
              n874 = call "myRIO_BRig_RT_dataLC_Selection_Count_NS_l1.vi"() -> ("output_Selection_Count_NS_l1"=w1615:i32)  [unwired: 11 in]
              n875 = local read "LC_Cue1_delayOpt_NS_l1"() -> (w1633:bool)
              n876 = local read "LC_Cue1_Probability_NS_l1"() -> (w1629:u16)
              n877 = local read "LC_Cue1_Tdelay_NS_l1"() -> (w1628:u16)
              n878 = local read "LC_Cue1_Count_NS_l1"() -> (w1627:u16)
              n879 = local read "LC_Cue1_Block_NS_l1"() -> (w1631:u16)
              n880 = local read "LC_Sel_Probability_NS_l1"() -> (w1617:u16)
              n881 = local read "LC_Sel_Tdelay_NS_l1"() -> (w1616:u16)
              n882 = local read "LC_Sel_OnOff_NS_l1"() -> (w1619:bool)
              n883 = local read "LC_Sel_Count_NS_l1"() -> (w1614:u16)
              n884 = local read "LC_Sel_Block_NS_l1"() -> (w1621:u16)
              n885 = Boolean To (0,1)(Boolean=w1643) -> (0, 1=w1645:i16)
              n886 = Boolean To (0,1)(Boolean=w1664) -> (0, 1=w1663:i16)
              n887 = Boolean To (0,1)(Boolean=w1632) -> (0, 1=w1635:i16)
              n888 = To Unsigned Word Integer(number=w1645) -> (unsigned 16bit integer=w1642:u16)
              n889 = To Unsigned Word Integer(number=w1663) -> (unsigned 16bit integer=w1662:u16)
              n890 = To Unsigned Word Integer(number=w1635) -> (unsigned 16bit integer=w1630:u16)
              n891 = Boolean To (0,1)(Boolean=w1633) -> (0, 1=w1634:i16)
              n892 = Boolean To (0,1)(Boolean=w1619) -> (0, 1=w1620:i16)
              n893 = To Unsigned Word Integer(number=w1634) -> (unsigned 16bit integer=w1626:u16)
              n894 = To Unsigned Word Integer(number=w1620) -> (unsigned 16bit integer=w1618:u16)
              n895 = Replace Array Subset(array=w1668, new element #1=w1666, index #1=w1667, new element #2=w1662, index #2=w1665, new element #3=w1660, index #3=w1661, new element #4=w1658, index #4=w1659, new element #5=w1656, index #5=w1657, new element #6=w1642, index #6=w1644, new element #7=w1631, index #7=w1641, new element #8=w1630, index #8=w1640, new element #9=w1629, index #9=w1639, new element #10=w1628, index #10=w1638, new element #11=w1627, index #11=w1637, new element #12=w1626, index #12=w1636, new element #13=w1621, index #13=w1625, new element #14=w1618, index #14=w1624, new element #15=w1617, index #15=w1623, new element #16=w1616, index #16=w1622, new element #17=w1614, index #17=w1615) -> (w1669:u16[])
            }
            frame "saveSettings_LC_Cue_l2" {
              # "Selection All"
              # "Count"
              # "Tdelay"
              # "Probability"
              # "OnOff"
              # "Block"
              # "delayOpt"
              # "Count"
              # "Tdelay"
              # "Probability"
              # "OnOff"
              # "Block"
              # "Cue1 All"
              # "delayOpt"
              # "Count"
              # "Tdelay"
              # "Probability"
              # "OnOff"
              # "Block"
              # "Cue1 First"
              n896 = call "myRIO_BRig_RT_dataLC_Cue1_delayOpt_Switch_l2.vi"() -> ("output_Cue1_delayOpt_Switch_l2"=w1708:i32)  [unwired: 11 in]
              n897 = call "myRIO_BRig_RT_dataLC_Cue1_Block_Switch_l2.vi"() -> ("output_Cue1_Block_Switch_l2"=w1731:i32)  [unwired: 11 in]
              n898 = call "myRIO_BRig_RT_dataLC_Cue1_OnOff_Switch_l2.vi"() -> ("output_Cue1_OnOff_Switch_l2"=w1729:i32)  [unwired: 11 in]
              n899 = call "myRIO_BRig_RT_dataLC_Cue1_Probability_Switch_l2.vi"() -> ("output_Cue1_l2_First_Probability"=w1725:i32)  [unwired: 11 in]
              n900 = call "myRIO_BRig_RT_dataLC_Cue1_Tdelay_Switch_l2.vi"() -> ("output_Cue1_Tdelay_Switch_l2"=w1723:i32)  [unwired: 11 in]
              n901 = call "myRIO_BRig_RT_dataLC_Cue1_Count_Switch_l2.vi"() -> ("output_Cue1_Count_Switch_l2"=w1721:i32)  [unwired: 11 in]
              n902 = local read "LC_Cue1_delayOpt_Switch_l2"() -> (w1707:bool)
              n903 = call "myRIO_BRig_RT_dataLC_Cue1_Block_NS_l2.vi"() -> ("output_Cue1_Block_NS_l2"=w1705:i32)  [unwired: 11 in]
              n904 = call "myRIO_BRig_RT_dataLC_Cue1_OnOff_NS_l2.vi"() -> ("output_Cue1_OnOff_NS_l2"=w1704:i32)  [unwired: 11 in]
              n905 = call "myRIO_BRig_RT_dataLC_Cue1_Probability_NS_l2.vi"() -> ("output_Cue1_l2_All_Probability"=w1703:i32)  [unwired: 11 in]
              n906 = call "myRIO_BRig_RT_dataLC_Cue1_Tdelay_NS_l2.vi"() -> ("output_Cue1_Tdelay_NS_l2"=w1702:i32)  [unwired: 11 in]
              n907 = call "myRIO_BRig_RT_dataLC_Cue1_Count_NS_l2.vi"() -> ("output_Cue1_Count_NS_l2"=w1701:i32)  [unwired: 11 in]
              n908 = call "myRIO_BRig_RT_dataLC_Cue1_delayOpt_NS_l2.vi"() -> ("output_Cue1_delayOpt_NS_l2"=w1700:i32)  [unwired: 11 in]
              n909 = local read "LC_Cue1_Count_Switch_l2"() -> (w1720:u16)
              n910 = local read "LC_Cue1_Probability_Switch_l2"() -> (w1724:u16)
              n911 = local read "LC_Cue1_Block_Switch_l2"() -> (w1730:u16)
              n912 = local read "LC_Cue1_Tdelay_Switch_l2"() -> (w1722:u16)
              n913 = local read "LC_Cue1_OnOff_Switch_l2"() -> (w1728:bool)
              n914 = local read "LC_Cue1_OnOff_NS_l2"() -> (w1696:bool)
              n915 = call "myRIO_BRig_RT_dataLC_Selection_Block_NS_l1.vi"() -> ("output_Selection_Block_NS_l1"=w1689:i32)  [unwired: 11 in]
              n916 = call "myRIO_BRig_RT_dataLC_Selection_OnOff_NS_l1.vi"() -> ("output_Selection_OnOff_NS_l1"=w1688:i32)  [unwired: 11 in]
              n917 = call "myRIO_BRig_RT_dataLC_Selection_Probability_NS_l1.vi"() -> ("output_Selection_Probability_NS_l1"=w1687:i32)  [unwired: 11 in]
              n918 = call "myRIO_BRig_RT_dataLC_Selection_Tdelay_NS_l1.vi"() -> ("output_Selection_Tdelay_NS_l1"=w1686:i32)  [unwired: 11 in]
              n919 = call "myRIO_BRig_RT_dataLC_Selection_Count_NS_l1.vi"() -> ("output_Selection_Count_NS_l1"=w1679:i32)  [unwired: 11 in]
              n920 = local read "LC_Cue1_delayOpt_NS_l2"() -> (w1697:bool)
              n921 = local read "LC_Cue1_Probability_NS_l2"() -> (w1693:u16)
              n922 = local read "LC_Cue1_Tdelay_NS_l2"() -> (w1692:u16)
              n923 = local read "LC_Cue1_Count_NS_l2"() -> (w1691:u16)
              n924 = local read "LC_Cue1_Block_NS_l2"() -> (w1695:u16)
              n925 = local read "LC_Sel_Probability_NS_l1"() -> (w1681:u16)
              n926 = local read "LC_Sel_Tdelay_NS_l1"() -> (w1680:u16)
              n927 = local read "LC_Sel_OnOff_NS_l1"() -> (w1683:bool)
              n928 = local read "LC_Sel_Count_NS_l1"() -> (w1678:u16)
              n929 = local read "LC_Sel_Block_NS_l1"() -> (w1685:u16)
              n930 = Boolean To (0,1)(Boolean=w1707) -> (0, 1=w1709:i16)
              n931 = Boolean To (0,1)(Boolean=w1728) -> (0, 1=w1727:i16)
              n932 = Boolean To (0,1)(Boolean=w1696) -> (0, 1=w1699:i16)
              n933 = To Unsigned Word Integer(number=w1709) -> (unsigned 16bit integer=w1706:u16)
              n934 = To Unsigned Word Integer(number=w1727) -> (unsigned 16bit integer=w1726:u16)
              n935 = To Unsigned Word Integer(number=w1699) -> (unsigned 16bit integer=w1694:u16)
              n936 = Boolean To (0,1)(Boolean=w1697) -> (0, 1=w1698:i16)
              n937 = Boolean To (0,1)(Boolean=w1683) -> (0, 1=w1684:i16)
              n938 = To Unsigned Word Integer(number=w1698) -> (unsigned 16bit integer=w1690:u16)
              n939 = To Unsigned Word Integer(number=w1684) -> (unsigned 16bit integer=w1682:u16)
              n940 = Replace Array Subset(array=w1732, new element #1=w1730, index #1=w1731, new element #2=w1726, index #2=w1729, new element #3=w1724, index #3=w1725, new element #4=w1722, index #4=w1723, new element #5=w1720, index #5=w1721, new element #6=w1706, index #6=w1708, new element #7=w1695, index #7=w1705, new element #8=w1694, index #8=w1704, new element #9=w1693, index #9=w1703, new element #10=w1692, index #10=w1702, new element #11=w1691, index #11=w1701, new element #12=w1690, index #12=w1700, new element #13=w1685, index #13=w1689, new element #14=w1682, index #14=w1688, new element #15=w1681, index #15=w1687, new element #16=w1680, index #16=w1686, new element #17=w1678, index #17=w1679) -> (w1733:u16[])
            }
            frame "saveSettings6_LC_l1_Other" {
              # "Trial"
              # "Tdelay"
              # "Probability"
              # "OnOff"
              # "Block"
              # "Wrong"
              # "Trial"
              # "Tdelay"
              # "Probability"
              # "OnOff"
              # "Block"
              # "Reward"
              n941 = call "myRIO_BRig_RT_dataLC_Wrong_Block_l1.vi"() -> ("output_Wrong_Block_l1"=w1762:i32)  [unwired: 11 in]
              n942 = call "myRIO_BRig_RT_dataLC_Wrong_OnOff_l1.vi"() -> ("output_Wrong_OnOff_l1"=w1761:i32)  [unwired: 11 in]
              n943 = call "myRIO_BRig_RT_dataLC_Wrong_Probability_l1.vi"() -> ("output_Wrong_Probability_l1"=w1760:i32)  [unwired: 11 in]
              n944 = call "myRIO_BRig_RT_dataLC_Wrong_Tdelay_l1.vi"() -> ("output_Wrong_Tdelay_l1"=w1759:i32)  [unwired: 11 in]
              n945 = call "myRIO_BRig_RT_dataLC_Wrong_Trial_l1.vi"() -> ("output_Wrong_Trial_l1"=w1758:i32)  [unwired: 11 in]
              n946 = call "myRIO_BRig_RT_dataLC_Reward_Block_l1.vi"() -> ("output_Reward_Block_l1"=w1774:i32)  [unwired: 11 in]
              n947 = call "myRIO_BRig_RT_dataLC_Reward_OnOff_l1.vi"() -> ("output_Reward_OnOff_l1"=w1772:i32)  [unwired: 11 in]
              n948 = call "myRIO_BRig_RT_dataLC_Reward_Probability_l1.vi"() -> ("output_Reward_Probability_l1"=w1768:i32)  [unwired: 11 in]
              n949 = call "myRIO_BRig_RT_dataLC_Reward_Tdelay_l1.vi"() -> ("output_Reward_Tdelay_l1"=w1766:i32)  [unwired: 11 in]
              n950 = call "myRIO_BRig_RT_dataLC_Reward_Trial_l1.vi"() -> ("output_Reward_Trial_l1"=w1764:i32)  [unwired: 11 in]
              n951 = local read "LC_Wrong_OnOff_l1"() -> (w1756:bool)
              n952 = local read "LC_Wrong_Probability_l1"() -> (w1753:u16)
              n953 = local read "LC_Wrong_Block_l1"() -> (w1755:u16)
              n954 = local read "LC_Wrong_Tdelay_l1"() -> (w1752:u16)
              n955 = local read "LC_Wrong_Trial_l1"() -> (w1751:u16)
              n956 = local read "LC_Reward_Probability_l1"() -> (w1767:u16)
              n957 = local read "LC_Reward_Block_l1"() -> (w1773:u16)
              n958 = local read "LC_Reward_Tdelay_l1"() -> (w1765:u16)
              n959 = local read "LC_Reward_OnOff_l1"() -> (w1771:bool)
              n960 = local read "LC_Reward_Trial_l1"() -> (w1763:u16)
              n961 = Boolean To (0,1)(Boolean=w1756) -> (0, 1=w1757:i16)
              n962 = Boolean To (0,1)(Boolean=w1771) -> (0, 1=w1770:i16)
              n963 = To Unsigned Word Integer(number=w1757) -> (unsigned 16bit integer=w1754:u16)
              n964 = To Unsigned Word Integer(number=w1770) -> (unsigned 16bit integer=w1769:u16)
              n965 = Replace Array Subset(array=w1775, new element #1=w1773, index #1=w1774, new element #2=w1769, index #2=w1772, new element #3=w1767, index #3=w1768, new element #4=w1765, index #4=w1766, new element #5=w1763, index #5=w1764, new element #6=w1755, index #6=w1762, new element #7=w1754, index #7=w1761, new element #8=w1753, index #8=w1760, new element #9=w1752, index #9=w1759, new element #10=w1751, index #10=w1758) -> (w1776:u16[])
            }
            frame "SaveSettings6_LC_l2_Other" {
              # "Trial"
              # "Tdelay"
              # "Probability"
              # "OnOff"
              # "Block"
              # "Wrong"
              # "Trial"
              # "Tdelay"
              # "Probability"
              # "OnOff"
              # "Block"
              # "Reward"
              n966 = call "myRIO_BRig_RT_dataLC_Wrong_Block_l1.vi"() -> ("output_Wrong_Block_l1"=w1806:i32)  [unwired: 11 in]
              n967 = call "myRIO_BRig_RT_dataLC_Wrong_OnOff_l1.vi"() -> ("output_Wrong_OnOff_l1"=w1805:i32)  [unwired: 11 in]
              n968 = call "myRIO_BRig_RT_dataLC_Wrong_Probability_l1.vi"() -> ("output_Wrong_Probability_l1"=w1804:i32)  [unwired: 11 in]
              n969 = call "myRIO_BRig_RT_dataLC_Wrong_Tdelay_l1.vi"() -> ("output_Wrong_Tdelay_l1"=w1803:i32)  [unwired: 11 in]
              n970 = call "myRIO_BRig_RT_dataLC_Wrong_Trial_l1.vi"() -> ("output_Wrong_Trial_l1"=w1802:i32)  [unwired: 11 in]
              n971 = call "myRIO_BRig_RT_dataLC_Reward_Block_l1.vi"() -> ("output_Reward_Block_l1"=w1818:i32)  [unwired: 11 in]
              n972 = call "myRIO_BRig_RT_dataLC_Reward_OnOff_l1.vi"() -> ("output_Reward_OnOff_l1"=w1816:i32)  [unwired: 11 in]
              n973 = call "myRIO_BRig_RT_dataLC_Reward_Probability_l1.vi"() -> ("output_Reward_Probability_l1"=w1812:i32)  [unwired: 11 in]
              n974 = call "myRIO_BRig_RT_dataLC_Reward_Tdelay_l1.vi"() -> ("output_Reward_Tdelay_l1"=w1810:i32)  [unwired: 11 in]
              n975 = call "myRIO_BRig_RT_dataLC_Reward_Trial_l1.vi"() -> ("output_Reward_Trial_l1"=w1808:i32)  [unwired: 11 in]
              n976 = local read "LC_Wrong_OnOff_l1"() -> (w1800:bool)
              n977 = local read "LC_Wrong_Probability_l1"() -> (w1797:u16)
              n978 = local read "LC_Wrong_Block_l1"() -> (w1799:u16)
              n979 = local read "LC_Wrong_Tdelay_l1"() -> (w1796:u16)
              n980 = local read "LC_Wrong_Trial_l1"() -> (w1795:u16)
              n981 = local read "LC_Reward_Probability_l1"() -> (w1811:u16)
              n982 = local read "LC_Reward_Block_l1"() -> (w1817:u16)
              n983 = local read "LC_Reward_Tdelay_l1"() -> (w1809:u16)
              n984 = local read "LC_Reward_OnOff_l1"() -> (w1815:bool)
              n985 = local read "LC_Reward_Trial_l1"() -> (w1807:u16)
              n986 = Boolean To (0,1)(Boolean=w1800) -> (0, 1=w1801:i16)
              n987 = Boolean To (0,1)(Boolean=w1815) -> (0, 1=w1814:i16)
              n988 = To Unsigned Word Integer(number=w1801) -> (unsigned 16bit integer=w1798:u16)
              n989 = To Unsigned Word Integer(number=w1814) -> (unsigned 16bit integer=w1813:u16)
              n990 = Replace Array Subset(array=w1819, new element #1=w1817, index #1=w1818, new element #2=w1813, index #2=w1816, new element #3=w1811, index #3=w1812, new element #4=w1809, index #4=w1810, new element #5=w1807, index #5=w1808, new element #6=w1799, index #6=w1806, new element #7=w1798, index #7=w1805, new element #8=w1797, index #8=w1804, new element #9=w1796, index #9=w1803, new element #10=w1795, index #10=w1802) -> (w1820:u16[])
            }
            frame "setSettings_Audio" {
              # "amp_L"
              # "amp_R"
              # "freq_L"
              # "freq_R"
              n991 = call "myRIO_BRig_RT_dataExp_Audio_amp__L.vi"() -> ("output_Audio_amp__L"=w1845:i32)  [unwired: 11 in]
              n992 = call "myRIO_BRig_RT_dataExp_Audio_amp__R.vi"() -> ("output_Audio_amp__R"=w1844:i32)  [unwired: 11 in]
              n993 = call "myRIO_BRig_RT_dataExp_Audio_freq__L.vi"() -> ("output_Audio_freq__L"=w1843:i32)  [unwired: 11 in]
              n994 = call "myRIO_BRig_RT_dataExp_Audio_freq__R.vi"() -> ("output_Audio_freq__R"=w1842:i32)  [unwired: 11 in]
              n995 = Index Array(array=w1841, index #1=w1845, index #2=w1844, index #3=w1843, index #4=w1842) -> (element #1=w1840:u16, element #2=w1839:u16, element #3=w1832:u16, element #4=w1830:u16)
              n996 = To Unsigned Byte Integer(number=w1832) -> (unsigned 8bit integer=w1831:u8)
              n997 = To Unsigned Byte Integer(number=w1830) -> (unsigned 8bit integer=w1829:u8)
            }
            frame "setSettings_Laser" {
              w1867 = u32 0 ("laser2_selRew_Ndelay")
              # "tDelay"
              # "Wrong l1"
              # "Reward l1"
              n998 = local read "Laser_Tpeak_l1"() -> (w1881:dbl)
              n999 = local read "Laser_Tshutter_l1"() -> (w1879:dbl)
              n1000 = local read "Laser_Freq_l1"() -> (w1880:dbl)
              n1001 = local read "Laser_duration_l1"() -> (w1876:u16)
              n1002 = local read "Laser_Tpeak_l2"() -> (w1875:dbl)
              n1003 = local read "Laser_Tshutter_l2"() -> (w1873:dbl)
              n1004 = local read "Laser_Freq_l2"() -> (w1874:dbl)
              n1005 = local read "Laser_duration_l2"() -> (w1872:u16)
              n1006 = local read "CueLed_Freq"() -> (w1859:dbl)
              n1007 = local read "CueLed_duration"() -> (w1858:u16)
              n1008 = local read "CueLed_Tpeak"() -> (w1860:dbl)
              n1009 = call "myRIO_BRig_RT_dataLC_Reward_Tdelay_l1.vi"() -> ("output_Reward_Tdelay_l1"=w1894:i32)  [unwired: 11 in]
              n1010 = call "myRIO_BRig_RT_dataLC_Wrong_Tdelay_l1.vi"() -> ("output_Wrong_Tdelay_l1"=w1895:i32)  [unwired: 11 in]
              n1011 = local read "FPGA_count2ms"() -> (w1861:dbl)
              n1012 = Index Array(array=w1891, index #1=w1894, index #2=w1895) -> (element #1=w1893:u16, element #2=w1892:u16)
              n1013 = To Double Precision Float(number=w1893) -> (double precision float=w1888:dbl)
              n1014 = To Double Precision Float(number=w1892) -> (double precision float=w1885:dbl)
              n1015 = To Unsigned Word Integer(number=w1861) -> (unsigned 16bit integer=w1882:u16)
              n1016 = call "myRIO_BRig_RT__calc_laser_FPGA_N.vi"("input_FPGA_count2ms"=w1861, "input_Tpeak"=w1881, "input_Freq"=w1880, "input_Tshutter"=w1879, "input_duration"=w1876) -> ("output_laser_Npeak"=w1866:u32, "output_laser_Nvalley"=w1865:u32, "output_laser_Nshutter"=w1864:u32, "output_laser_Nduration"=w1878:u32, "output_laser_Tduration"=w1877:u16)  [unwired: 6 in]
              n1017 = Multiply(x=w1861, y=w1888) -> (x*y=w1889:dbl)
              n1018 = Multiply(x=w1861, y=w1885) -> (x*y=w1886:dbl)
              n1019 = call "myRIO_BRig_RT__calc_laser_FPGA_N__CueLed.vi"("input_FPGA_count2ms"=w1861, "input_Tpeak"=w1860, "input_Freq"=w1859, "input_duration"=w1858) -> ("output_laser_Npeak"=w1857:u32, "output_laser_Nvalley"=w1856:u32, "output_laser_Tduration"=w1854:u16)  [unwired: 9 in]
              n1020 = call "myRIO_BRig_RT__calc_laser_FPGA_N.vi"("input_FPGA_count2ms"=w1861, "input_Tpeak"=w1875, "input_Freq"=w1874, "input_Tshutter"=w1873, "input_duration"=w1872) -> ("output_laser_Npeak"=w1871:u32, "output_laser_Nvalley"=w1870:u32, "output_laser_Nshutter"=w1869:u32, "output_laser_Nduration"=w1868:u32, "output_laser_Tduration"=w1862:u16)  [unwired: 6 in]
              n1021 = Round Toward +Infinity(x=w1889) -> (ceil(x): smallest int >= x=w1890:dbl)
              n1022 = Round Toward +Infinity(x=w1886) -> (ceil(x): smallest int >= x=w1887:dbl)
              n1023 = To Unsigned Long Integer(number=w1890) -> (unsigned 32bit integer=w1884:u32)
              n1024 = To Unsigned Long Integer(number=w1887) -> (unsigned 32bit integer=w1883:u32)
              n1025 = xnode "Read/Write Control"("FPGA VI Reference In"=w1898, "error in"=w1899, "LC_nPeak_l1"=w1866, "LC_nValley_l1"=w1865, "LC_nShutter_l1"=w1864, "LR_reward_nDelay_l1"=w1884, "LR_wrong_nDelay_l1"=w1883, "LR_reward_nTotal_l1"=w1878, "LR_wrong_nTotal_l1"=w1878, "k1__counter_per_ms"=w1882, "LC_nPeak_l2"=w1871, "LC_nValley_l2"=w1870, "LC_nShutter_l2"=w1869, "LR_reward_nDelay_l2"=w1867, "LR_wrong_nDelay_l2"=w1867, "LR_reward_nTotal_l2"=w1868, "LR_wrong_nTotal_l2"=w1868, "CueLed_nPeak"=w1857, "CueLed_nValley"=w1856) -> ("error out"=→"error out":errorcluster)  [unwired: 1 out]
              n1026 = call "myRIO_BRig_RT_dataCurrent_laser1_pulse_duration.vi"() -> ("output_laser1_pulse_duration"=w1896:i32)  [unwired: 11 in]
              n1027 = call "myRIO_BRig_RT_dataCurrent_laser2_pulse_duration.vi"() -> ("output_laser2_pulse_duration"=w1863:i32)  [unwired: 11 in]
              n1028 = call "myRIO_BRig_RT_dataCurrent_CueLed_pulse_duration.vi"() -> ("output_CueLed_pulse_duration"=w1855:i32)  [unwired: 11 in]
              n1029 = Replace Array Subset(array=w1891, new element #1=w1877, index #1=w1896, new element #2=w1862, index #2=w1863, new element #3=w1854, index #3=w1855) -> (w1897:u16[])
            }
            frame "initBlock" {
              n1030 = call "myRIO_Brig_RT__Case_Exp_State_initBlock.vi"("input_spout"=w1943, "input_dataExp"=w1941, "input_dataCurrent"=w1942) -> ("output_spout"=w1921:enum16{"Left", "Right"}, "output_state"=w1944:T2, "output_dataExp"=w1940:u16[], "output_dataCurrent"=w1926:u16[], "output_TpB_target"=→"TpB_target":u16)  [unwired: 4 in]
              "cSpout" <- w1921
              n1031 = call "myRIO_BRig_RT_dataCurrent_iBlock.vi"() -> ("output_iBlock"=w1925:i32)  [unwired: 11 in]
              n1032 = Index Array(array=w1926, index=w1925) -> (element=w1919:u16)
              "iBlock" <- w1919
            }
            frame "initBlock2" {
              n1033 = local write "nRewards_cur"(u16 0 ("nRewards_cur")) -> ()
              n1034 = call "myRIO_BRig_RT__Case_Exp_State_initBlock2.vi"("input_spout"=w1952, "input_dataBlock"=w1953, "input_dataCurrent"=w1951) -> ("idxDataBlock"=w1948:i32, "output_dataBlock"=w1950:u16[][])  [unwired: 7 in]
            }
            frame "initTrial" {
              n1035 = call "myRIO_Brig_RT__Case_Exp_State_initTrial.vi"("input_spout"=w1966, "input_dataExp"=w1987, "input_dataCurrent"=w1988) -> ("output_state"=w1989:T2, "output_dataExp"=w1986:u16[], "output_dataCurrent"=w1976:u16[])  [unwired: 6 in]
              n1036 = call "myRIO_BRig_RT_dataCurrent_iTrial.vi"() -> ("output_iTrial"=w1975:i32)  [unwired: 11 in]
              n1037 = call "myRIO_BRig_RT_dataCurrent_SolenoidReward.vi"() -> ("output_SolenoidReward"=w1971:i32)  [unwired: 11 in]
              n1038 = Index Array(array=w1976, index #1=w1975, index #2=w1971) -> (element #1=w1967:u16, element #2=w1970:u16)
              "iTrial" <- w1967
              n1039 = Not Equal To 0?(x=w1970) -> (x != 0?=→"SolenoidReward":bool)
            }
            frame "initTrial2" {
              # "trialUntilReward"
              n1040 = call "myRIO_BRig_RT__Case_Exp_subState_LC__initTrial.vi"("input_dataTrial"=w1996, "input_spout"=w2005, "input_dataCurrent"=w1994, "input_dataLC"=w1993) -> ("output_LC_Wrong"=w2006:bool, "output_LC_led_Wrong"=w1998:bool, "output_LC_Reward"=w2007:bool, "output_LC_led_Reward"=w1997:bool, "output_dataTrial"=w1995:u16[][])  [unwired: 2 in]
              n1041 = Equal?(x=w2005, y=enum16{"Left", "Right"}."Right") -> (x = y?=w2003:bool)
              n1042 = call "myRIO_BRig_RT_dataExp_ItrialUntilReward.vi"() -> ("output_I_trialUntilReward"=w2001:i32)  [unwired: 11 in]
              n1043 = Index Array(array=w2002, index=w2001) -> (element=w2000:u16)
              n1044 = Not Equal To 0?(x=w2000) -> (x != 0?=w1999:bool)
              n1045 = xnode "Read/Write Control"("FPGA VI Reference In"=w2020, "error in"=w2019, "SelectionState"=FALSE, "LR_reward_Laser_l1"=w2007, "LR_wrong_Laser_l1"=w2006, "LR_reward_Event_l1"=w1997, "LR_wrong_Event_l1"=w1998, "Left(F)_or_Right(T)"=w2003, "ignoreWrong"=w1999) -> ("error out"=→"error_initTrial":errorcluster)  [unwired: 1 out]
            }
            frame "initTrial3" {
              n1046 = call "myRIO_BRig_RT_arrTrig_init.vi"() -> ("output_arrTrig"=w2026:bool[])  [unwired: 11 in]
              n1047 = call "myRIO_BRig_RT__Case_Exp_State_initTrial_dataTrial.vi"("input_spout"=w2036, "input_dataCurrent"=w2037, "input_dataExp"=w2035, "input_dataTrial"=w2039) -> ("output_dataTrial"=w2038:u16[][], "output_laserPower_l1"=w2032:u16)  [unwired: 5 in, 1 out]
              n1048 = To Double Precision Float(number=w2032) -> (double precision float=w2034:dbl)
              n1049 = Divide(x=w2034, y=100.0 ("x")) -> (x/y=w2028:dbl)
              "output_PortA" <- w2028
              n1050 = call "myRIO__convert__Voltage_to_FPGAvalue.vi"("input_voltage"=w2028) -> ("output_PortC"=w2027:i16)  [unwired: 9 in, 1 out]
              n1051 = xnode "Read/Write Control"("FPGA VI Reference In"=w2031, "error in"=w2030, "AnaOut_0"=w2027) -> ("error out"=→"error out 4":errorcluster)  [unwired: 1 out]
            }
            frame "initTrial4" {
              n1052 = call "myRIO_BRig_RT_dataCurrent_idxDataTrial.vi"() -> ("output_idxDataTrial"=w2065:i32)  [unwired: 11 in]
              n1053 = call "myRIO_BRig_RT_dataTrial_activeRecording.vi"() -> ("output_activeRecording"=w2062:i32)  [unwired: 11 in]
              n1054 = Index Array(array=w2067, index=w2065) -> (element=w2064:u16)
              n1055 = Boolean To (0,1)(Boolean="Recording") -> (0, 1=w2061:i16)
              n1056 = To Long Integer(number=w2064) -> (32bit integer=w2063:i32)
              n1057 = To Unsigned Word Integer(number=w2061) -> (unsigned 16bit integer=w2060:u16)
              n1058 = Replace Array Subset(array=w2066, new element=w2060, index (row)=w2063, index (col)=w2062) -> (w2059:u16[][])
            }
            frame "initTrial_LC_ENL1" {
              n1059 = call "myRIO_BRig_RT__Case_Exp_State_initTrial_LC_ENL1__v2.vi"("input_dataTrial"=w2092, "input_spout"=w2097, "input_dataBlock"=w2090, "input_dataLC"=w2098, "input_dataCurrent"=w2094) -> ("output_LC__ENL1"=w2096:bool, "output_LC_led__ENL1"=w2095:bool, "output_dataTrial"=w2091:u16[][], "output_dataCurrent"=w2093:u16[])  [unwired: 3 in]
            }
            frame "initTrial_LC_Cue1" {
              n1060 = call "myRIO_BRig_RT__Case_Exp_State_initTrial_LC_Cue1__v3.vi"("input_dataTrial"=w2119, "input_spout"=w2122, "input_arrTrig"=w2114, "input_dataBlock"=w2117, "input_dataLC"=w2123, "input_dataCurrent"=w2121) -> ("output_arrTrig"=w2113:bool[], "output_dataTrial"=w2118:u16[][], "output_dataCurrent"=w2120:u16[])  [unwired: 3 in]
            }
            frame "initTrial_LC_Cue1_2" {
              w2151 = TRUE ("Recording")
              n1061 = local read "Cue1Param_AudioLed_Probability_Switch"() -> (w2144:u16)
              n1062 = local read "Cue1Param_AudioLed_Count_Switch"() -> (w2143:u16)
              n1063 = local read "Cue1Param_AudioLed_Probability_NS"() -> (w2141:u16)
              n1064 = local read "Cue1Param_AudioLed_Count_NS"() -> (w2140:u16)
              n1065 = local read "Cue1Param_CueType_Switch"() -> (w2145:u16)
              n1066 = local read "Cue1Param_CueType_NS"() -> (w2142:u16)
              n1067 = call "myRIO_BRig_RT__Case_Exp_State_initTrial_LC_Cue1_2.vi"("input_CueType_Switch"=w2145, "input_Probability_Switch"=w2144, "input_Count_Switch"=w2143, "input_CueType_NS"=w2142, "input_Probability_NS"=w2141, "input_Count_NS"=w2140, "input_spout"=w2139, "input_dataBlock"=w2138, "input_dataCurrent"=w2149, "input_arrTrig"=w2147) -> ("output_dataCurrent"=w2148:u16[], "output_arrTrig"=w2146:bool[])  [unwired: 8 in]
            }
            frame "initTrial_LC_Sel" {
              n1068 = call "myRIO_BRig_RT__Case_Exp_State_initTrial_LC_Sel__v2.vi"("input_dataTrial"=w2180, "input_spout"=w2183, "input_dataBlock"=w2178, "input_dataLC"=w2184, "input_dataCurrent"=w2182) -> ("output_LC__Sel"=w2170:bool, "output_LC_led__Sel"=w2171:bool, "output_dataTrial"=w2179:u16[][], "output_dataCurrent"=w2181:u16[])  [unwired: 3 in]
              n1069 = local read "Recording"() -> (w2175:bool)
            }
            frame "ENL1_pre" {
              # "ENL1_n"
              # "Tcycle"
              # "counter"
              n1070 = call "myRIO_BRig_RT_dataCurrent_Tcycle_generic.vi"() -> ("output_Tcycle_generic"=w2231:i32)  [unwired: 11 in]
              n1071 = call "myRIO_BRig_RT_dataCurrent_count_generic.vi"() -> ("output_count_generic"=w2233:i32)  [unwired: 11 in]
              n1072 = call "myRIO_BRig_RT_dataCurrent_Tcycle_ENL.vi"() -> ("output_ENL"=w2230:i32)  [unwired: 11 in]
              n1073 = call "myRIO_BRig_RT_dataCurrent_nENL1.vi"() -> ("output_nENL1"=w2204:i32)  [unwired: 11 in]
              n1074 = Index Array(array=w2224, index #1=w2230, index #2=w2204) -> (element #1=w2229:u16, element #2=w2203:u16)
              n1075 = Increment(x=w2203) -> (x+1=w2202:u16)
              n1076 = Replace Array Subset(array=w2224, new element #1=u16 0 ("new element/subarray"), index #1=w2233, new element #2=w2229, index #2=w2231, new element #3=w2202, index #3=w2204) -> (w2228:u16[])
              n1077 = Select(t=myRIO_BRig_RT__Case_Exp_stateList."ENL1Penalty_pre" ("Enum"), s=w2212, f=myRIO_BRig_RT__Case_Exp_stateList."ENL1" ("Enum")) -> (s? t:f=w2209:T2)
            }
            frame "ENL1" {
              n1078 = call "myRIO_BRig_RT__Case_Exp_State_ENL1__v2.vi"("input_LC"=w2241, "I_lick"=w2244, "input_LC_led"=w2242, "input_state"=w2250, "input_dataCurrent"=w2249) -> ("output_trigger_laser_led"=w2240:bool, "output_state"=w2247:T2, "output_dataCurrent"=w2248:u16[], "output_trigger_laser"=w2239:bool)  [unwired: 3 in]
            }
            frame "ENL1Penalty_pre" {
              # "Tcycle"
              # "counter"
              n1079 = call "myRIO_BRig_RT_dataCurrent_Tcycle_generic.vi"() -> ("output_Tcycle_generic"=w2291:i32)  [unwired: 11 in]
              n1080 = call "myRIO_BRig_RT_dataCurrent_count_generic.vi"() -> ("output_count_generic"=w2293:i32)  [unwired: 11 in]
              n1081 = call "myRIO_BRig_RT_dataExp_ENL_penalty.vi"() -> ("output_ENL_penalty"=w2286:i32)  [unwired: 11 in]
              n1082 = Index Array(array=w2287, index=w2286) -> (element=w2290:u16)
              n1083 = Replace Array Subset(array=w2288, new element #1=u16 0 ("new element/subarray"), index #1=w2293, new element #2=w2290, index #2=w2291) -> (w2289:u16[])
            }
            frame "ENL1Penalty" {
              n1084 = call "myRIO_BRig_RT__Case_Exp_State_ENL1Penalty.vi"("input_state"=w2317, "input_dataCurrent"=w2321) -> ("output_state"=w2318:T2, "output_dataCurrent"=w2320:u16[])  [unwired: 8 in]
            }
            frame "ENL2_pre" {
            }
            frame "ENL2" {
            }
            frame "ENL2Penalty_pre" {
            }
            frame "ENL2Penalty" {
            }
            frame "Cue1_pre" {
              # "Cue1_n"
              # "Tcycle_Cue1"
              # "0 = L, 1 = R, 2 = both"
              # "sp_R"
              # "sp_L"
              # "Tcycle"
              # "counter"
              n1085 = call "myRIO_BRig_RT_arrTrig_Cue1_CueType_AudioLed.vi"() -> ("output_arrTrig_Cue1_CueType_AudioLed"=w2408:i32)  [unwired: 11 in]
              n1086 = Index Array(array=w2409, index=w2408) -> (element=w2407:bool)
              n1087 = Equal?(x=w2438, y=enum16{"Left", "Right"}."Left") -> (x = y?=w2437:bool)
              n1088 = call "myRIO_BRig_RT_dataExp_Audio_sp__L.vi"() -> ("output_Audio_sp__L"=w2436:i32)  [unwired: 11 in]
              n1089 = call "myRIO_BRig_RT_dataExp_Audio_sp__R.vi"() -> ("output_Audio_sp__R"=w2435:i32)  [unwired: 11 in]
              n1090 = call "myRIO_BRig_RT_dataCurrent_Tcycle_generic.vi"() -> ("output_Tcycle_generic"=w2448:i32)  [unwired: 11 in]
              n1091 = call "myRIO_BRig_RT_dataCurrent_count_generic.vi"() -> ("output_count_generic"=w2450:i32)  [unwired: 11 in]
              n1092 = Not(x=w2407) -> (.not. x?=w2402:bool)
              n1093 = Select(t=w2436, s=w2437, f=w2435) -> (s? t:f=w2434:i32)
              n1094 = call "myRIO_BRig_RT_dataCurrent_nCue1.vi"() -> ("output_nCue1"=w2414:i32)  [unwired: 11 in]
              n1095 = call "myRIO_BRig_RT_dataCurrent_Tcycle_cue.vi"() -> ("output_Tcycle_cue"=w2423:i32)  [unwired: 11 in]
              n1096 = Index Array(array=w2440, index=w2434) -> (element=w2432:u16)
              n1097 = Index Array(array=w2424, index #1=w2423, index #2=w2414) -> (element #1=w2425:u16, element #2=w2416:u16)
              n1098 = Increment(x=w2416) -> (x+1=w2415:u16)
              n1099 = Not Equal To 0?(x=w2432) -> (x != 0?=w2404:bool)
              n1100 = Not Equal?(x=w2432, y=u16 1) -> (x != y?=w2406:bool)
              n1101 = Replace Array Subset(array=w2424, new element #1=u16 0 ("new element/subarray"), index #1=w2450, new element #2=w2425, index #2=w2448, new element #3=w2415, index #3=w2414) -> (w2447:u16[])
              n1102 = Select(t=myRIO_BRig_RT__Case_Exp_stateList."Cue1Penalty_pre" ("Enum"), s=w2420, f=myRIO_BRig_RT__Case_Exp_stateList."Cue1" ("Enum")) -> (s? t:f=w2421:T2)
              n1103 = And(x=w2404, y=w2402) -> (x .and. y?=w2403:bool)
              n1104 = And(x=w2406, y=w2402) -> (x .and. y?=w2405:bool)
            }
            frame "Cue1" {
              n1105 = call "myRIO_BRig_RT__Case_Exp_State_Cue1__v3.vi"("I_lick"=w2466, "input_arrTrig"=w2458, "input_state"=w2468, "input_dataCurrent"=w2486) -> ("output_l1_laserOn"=w2456:bool, "output_l1_laserEvent"=w2457:bool, "output_state"=w2467:T2, "output_dataCurrent"=w2485:u16[], "output_l2_laserEvent"=w2455:bool, "output_CueLed_Event"=w2453:bool, "output_l2_laserOn"=w2454:bool)  [unwired: 1 in]
              n1106 = Equal?(x=myRIO_BRig_RT__Case_Exp_stateList."Selection_pre", y=w2467) -> (x = y?=w2471:bool)
              n1107 = xnode "Read/Write Control"("FPGA VI Reference In"=w2470, "error in"=w2469, "SelectionState"=w2471) -> ()  [unwired: 2 out]
            }
            frame "Cue1Penalty_pre" {
              # "Tcycle"
              # "counter"
              n1108 = call "myRIO_BRig_RT_dataCurrent_Tcycle_generic.vi"() -> ("output_Tcycle_generic"=w2518:i32)  [unwired: 11 in]
              n1109 = call "myRIO_BRig_RT_dataCurrent_count_generic.vi"() -> ("output_count_generic"=w2520:i32)  [unwired: 11 in]
              n1110 = call "myRIO_BRig_RT_dataExp_Tcycle_CuePenalty.vi"() -> ("output_Tcycle_CuePenalty"=w2517:i32)  [unwired: 11 in]
              n1111 = Index Array(array=w2512, index=w2517) -> (element=w2516:u16)
              n1112 = Replace Array Subset(array=w2514, new element #1=u16 0 ("new element/subarray"), index #1=w2520, new element #2=w2516, index #2=w2518) -> (w2513:u16[])
            }
            frame "Cue1Penalty" {
              n1113 = call "myRIO_BRig_RT__Case_Exp_State_Cue1Penalty.vi"("input_state"=w2547, "input_dataCurrent"=w2548) -> ("output_state"=w2545:T2, "output_dataCurrent"=w2546:u16[])  [unwired: 8 in]
            }
            frame "Cue2_pre" {
              n1114 = call "myRIO_BRig_RT__Case_Exp_subState_LC__Cue2.vi"("input_spout"=w2565, "input_dataCurrent"=w2566, "input_dataLC"=w2564) -> ()  [unwired: 6 in, 2 out]
            }
            frame "Cue2" {
            }
            frame "Cue2Penalty_pre" {
            }
            frame "Cue2Penalty" {
            }
            frame "Selection_pre" {
              # "Tcycle"
              # "counter"
              n1115 = call "myRIO_BRig_RT_dataCurrent_laser1_tSel_start.vi"() -> ("output_laser1_tSel_start"=w2636:i32)  [unwired: 11 in]
              n1116 = xnode "Read/Write Control"("FPGA VI Reference In"=w2646, "error in"=w2647) -> ("error out"=→"error_Selection_pre":errorcluster, "SelectReward"=w2640:bool, "SelectWrong"=w2641:bool)  [unwired: 1 out]
              n1117 = call "myRIO_BRig_RT_dataExp_Tcycle_Selection.vi"() -> ("output_Tcycle_Selection"=w2666:i32)  [unwired: 11 in]
              n1118 = call "myRIO_BRig_RT_dataCurrent_Tcycle_generic.vi"() -> ("output_Tcycle_generic"=w2667:i32)  [unwired: 11 in]
              n1119 = call "myRIO_BRig_RT_dataCurrent_count_generic.vi"() -> ("output_count_generic"=w2669:i32)  [unwired: 11 in]
              n1120 = Index Array(array=w2637, index=w2636) -> (element=w2635:u16)
              n1121 = Index Array(array=w2663, index=w2666) -> (element=w2665:u16)
              n1122 = Equal To 0?(x=w2635) -> (x = 0?=w2633:bool)
              n1123 = Replace Array Subset(array=w2637, new element #1=u16 0 ("new element/subarray"), index #1=w2669, new element #2=w2665, index #2=w2667) -> (w2664:u16[])
              n1124 = Or(x=w2640, y=w2641) -> (x .or. y?=w2631:bool)
              n1125 = Not(x=w2631) -> (.not. x?=w2634:bool)
              n1126 = Compound Arithmetic op=AND(w2634, w2633, w2632) -> (w2629:bool)
              n1127 = And(x=w2629, y=w2630) -> (x .and. y?=w2628:bool)
              n1128 = Select(t=myRIO_BRig_RT__Case_Exp_stateList."SelectReward_pre" ("Enum"), s=w2640, f=myRIO_BRig_RT__Case_Exp_stateList."SelectWrong_pre" ("Enum")) -> (s? t:f=w2645:T2)
              n1129 = Select(t=w2645, s=w2631, f=myRIO_BRig_RT__Case_Exp_stateList."Selection" ("Enum")) -> (s? t:f=w2642:T2)
            }
            frame "Selection" {
              # "counter\nSelection"
              # "increment"
              # "get Tcycle"
              # "get count"
              n1130 = call "myRIO_BRig_RT_dataCurrent_Tcycle_generic.vi"() -> ("output_Tcycle_generic"=w2703:i32)  [unwired: 11 in]
              n1131 = call "myRIO_BRig_RT_dataCurrent_count_generic.vi"() -> ("output_count_generic"=w2699:i32)  [unwired: 11 in]
              n1132 = call "myRIO_BRig_RT_dataCurrent_laser1_tSel_start.vi"() -> ("output_laser1_tSel_start"=w2691:i32)  [unwired: 11 in]
              n1133 = call "myRIO_BRig_RT_dataCurrent_laser1_tSel_end.vi"() -> ("output_laser1_tSel_end"=w2690:i32)  [unwired: 11 in]
              n1134 = call "myRIO_BRig_RT__increment_u16.vi"() -> ("output_increment__u16"=w2677:u16)  [unwired: 11 in]
              n1135 = xnode "Read/Write Control"("FPGA VI Reference In"=w2710, "error in"=w2709) -> ("error out"=→"error_Selection":errorcluster, "SelectReward"=w2706:bool, "SelectWrong"=w2707:bool)  [unwired: 1 out]
              n1136 = call "myRIO_BRig_RT_dataCurrent_laser1_triggered_Sel.vi"() -> ("output_laser1_triggered_Selection"=w2678:i32)  [unwired: 11 in]
              n1137 = Index Array(array=w2704, index #1=w2703, index #2=w2699, index #3=w2691, index #4=w2690, index #5=w2678) -> (element #1=w2698:u16, element #2=w2676:u16, element #3=w2675:u16, element #4=w2681:u16, element #5=w2672:u16)
              n1138 = Increment(x=w2672) -> (x+1=w2673:u16)
              n1139 = Equal?(x=w2676, y=w2675) -> (x = y?=w2674:bool)
              n1140 = Add(x=w2676, y=w2677) -> (x+y=w2682:u16)
              n1141 = Greater Or Equal?(x=w2682, y=w2675) -> (x >= y?=w2679:bool)
              n1142 = Less Or Equal?(x=w2682, y=w2681) -> (x <= y?=w2680:bool)
              n1143 = Greater?(x=w2698, y=w2682) -> (0:w2684:bool)
              n1144 = Select(t=w2673, s=w2674, f=w2672) -> (s? t:f=w2671:u16)
              n1145 = Select(t=myRIO_BRig_RT__Case_Exp_stateList."SelectReward_pre" ("Enum"), s=w2706, f=myRIO_BRig_RT__Case_Exp_stateList."SelectWrong_pre" ("Enum")) -> (s? t:f=w2705:T2)
              n1146 = Or(x=w2706, y=w2707) -> (x .or. y?=w2685:bool)
              n1147 = Not(x=w2685) -> (.not. x?=w2686:bool)
              n1148 = Select(t=w2702, s=w2684, f=myRIO_BRig_RT__Case_Exp_stateList."SelectTimeout_pre" ("Enum")) -> (s? t:f=w2693:T2)
              n1149 = Compound Arithmetic op=AND(w2684, w2686, w2679, w2680, w2683) -> (w2688:bool)
              n1150 = Select(t=w2682, s=w2684, f=w2698) -> (s? t:f=w2696:u16)
              n1151 = Select(t=w2705, s=w2685, f=w2693) -> (s? t:f=w2708:T2)
              n1152 = And(x=w2688, y=w2687) -> (x .and. y?=w2689:bool)
              n1153 = call "myRIO_BRig_RT_dataCurrent_count_selection.vi"() -> ("output_count_generic"=w2697:i32)  [unwired: 11 in]
              n1154 = Replace Array Subset(array=w2704, new element #1=w2696, index #1=w2699, new element #2=w2696, index #2=w2697, new element #3=w2671, index #3=w2678) -> (w2701:u16[])
            }
            frame "SelectReward_pre" {
              # "iState"
              # "Tcycle\nReward"
              # "nRewTrials"
              # "Tcycle\nGeneric"
              # "counter"
              n1155 = call "myRIO_BRig_RT_dataCurrent_nRewTrials.vi"() -> ("output_nRewTrials"=w2742:i32)  [unwired: 11 in]
              n1156 = Equal?(x=w2751, y=enum16{"Left", "Right"}."Left") -> (x = y?=w2752:bool)
              n1157 = Index Array(array=w2743, index=w2742) -> (element=w2741:u16)
              n1158 = call "myRIO_BRig_RT_dataExp_Tcycle_Reward__L.vi"() -> ("output_Tcycle_Reward__L"=w2755:i32)  [unwired: 11 in]
              n1159 = call "myRIO_BRig_RT_dataExp_Tcycle_Reward__R.vi"() -> ("output_Tcycle_Reward__R"=w2756:i32)  [unwired: 11 in]
              n1160 = Increment(x=w2741) -> (x+1=w2740:u16)
              n1161 = Select(t=w2755, s=w2752, f=w2756) -> (s? t:f=w2754:i32)
              n1162 = call "myRIO_BRig_RT__Case_Exp_subState_LC__Reward.vi"("input_spout"=w2751, "input_dataCurrent"=w2743, "input_dataLC"=w2750) -> ()  [unwired: 6 in, 2 out]
              n1163 = call "myRIO_BRig_RT_dataCurrent_count_generic.vi"() -> ("output_count_generic"=w2745:i32)  [unwired: 11 in]
              n1164 = call "myRIO_BRig_RT_dataCurrent_Tcycle_generic.vi"() -> ("output_Tcycle_generic"=w2746:i32)  [unwired: 11 in]
              n1165 = Index Array(array=w2757, index=w2754) -> (element=w2747:u16)
              n1166 = call "myRIO_BRig_RT_dataCurrent_iState.vi"() -> ("output_iState"=w2735:i32)  [unwired: 11 in]
              n1167 = Replace Array Subset(array=w2743, new element #1=w2740, index #1=w2742, new element #2=u16 0 ("new element/subarray"), index #2=w2745, new element #3=w2747, index #3=w2746, new element #4=u16 1 ("new element/subarray"), index #4=w2735) -> (w2758:u16[])
            }
            frame "SelectReward" {
              n1168 = call "myRIO_BRig_RT__Case_Exp_State_Reward.vi"("input_dataCurrent"=w2779, "input_state"=w2776, "input_spout"=w2774) -> ("output_dataCurrent"=w2778:u16[], "output_state"=w2777:T2, "output__L"=w2772:bool, "output__R"=w2773:bool)  [unwired: 9 in]
            }
            frame "SelectRewardPost_pre" {
              # "nRewards"
              # "nRewTrials"
              # "Tcycle"
              # "counter"
              n1169 = call "myRIO_BRig_RT_dataBlock_nRewards__L.vi"() -> ("output_nRewards__L"=w2795:i32)  [unwired: 11 in]
              n1170 = call "myRIO_BRig_RT_dataBlock_nRewards__R.vi"() -> ("output_nRewards__R"=w2794:i32)  [unwired: 11 in]
              n1171 = call "myRIO_BRig_RT_dataCurrent_Tcycle_generic.vi"() -> ("output_Tcycle_generic"=w2814:i32)  [unwired: 11 in]
              n1172 = call "myRIO_BRig_RT_dataCurrent_count_generic.vi"() -> ("output_count_generic"=w2816:i32)  [unwired: 11 in]
              n1173 = case shown="\"Left\", Default" w2788 {
                tunnel: w2800 -> [w2821 w2825]
                tunnel: [w2820 w2825] -> w2799
                tunnel: [w2822 w2823] -> w2798
                tunnel: w2797 -> [w2822 w2824]
                frame "Left", Default {
                  n1174 = Increment(x=w2821) -> (x+1=w2820:u16)
                }
                frame "Right" {
                  n1175 = Increment(x=w2824) -> (x+1=w2823:u16)
                }
              }
              "nRewards_Left" <- w2799
              "nRewards_Right" <- w2798
              n1176 = Equal?(x=w2788, y=enum16{"Left", "Right"}."Left") -> (x = y?=w2787:bool)
              n1177 = Select(t=w2795, s=w2787, f=w2794) -> (s? t:f=w2793:i32)
              n1178 = call "myRIO_BRig_RT_dataExp_Tcycle_RewardPost.vi"() -> ("output_Tcycle_RewardPost"=w2810:i32)  [unwired: 11 in]
              n1179 = call "myRIO_BRig_RT_dataCurrent_nRewTrials.vi"() -> ("output_nRewTrials"=w2796:i32)  [unwired: 11 in]
              n1180 = Index Array(array=w2811, index=w2810) -> (element=w2813:u16)
              n1181 = Index Array(array=w2790, index=w2796) -> (element=w2785:u16)
              n1182 = Replace Array Subset(array=w2790, new element #1=u16 0 ("new element/subarray"), index #1=w2816, new element #2=w2813, index #2=w2814) -> (w2812:u16[])
              n1183 = Replace Array Subset(array=w2792, new element=w2785, index (row)=w2786, index (col)=w2793) -> (w2791:u16[][])
              n1184 = local write "nRewards_cur"(w2785) -> ()
            }
            frame "SelectRewardPost" {
              n1185 = call "myRIO_BRig_RT__Case_Exp_State_RewardPost.vi"("input_state"=w2840, "input_dataCurrent"=w2843) -> ("output_state"=w2841:T2, "output_dataCurrent"=w2842:u16[])  [unwired: 8 in]
            }
            frame "SelectWrong_pre" {
              # "iState"
              # "Tcycle"
              # "counter"
              n1186 = call "myRIO_BRig_RT_dataCurrent_Tcycle_generic.vi"() -> ("output_Tcycle_generic"=w2868:i32)  [unwired: 11 in]
              n1187 = call "myRIO_BRig_RT_dataCurrent_count_generic.vi"() -> ("output_count_generic"=w2870:i32)  [unwired: 11 in]
              n1188 = call "myRIO_BRig_RT_dataExp_Tcycle_Wrong.vi"() -> ("output_Tcycle_Wrong"=w2866:i32)  [unwired: 11 in]
              n1189 = call "myRIO_BRig_RT__Case_Exp_subState_LC__Wrong.vi"("input_spout"=w2862, "input_dataCurrent"=w2863, "input_dataLC"=w2860) -> ()  [unwired: 6 in, 2 out]
              n1190 = Index Array(array=w2864, index=w2866) -> (element=w2867:u16)
              n1191 = call "myRIO_BRig_RT_dataCurrent_iState.vi"() -> ("output_iState"=w2854:i32)  [unwired: 11 in]
              n1192 = Replace Array Subset(array=w2863, new element #1=u16 0 ("new element/subarray"), index #1=w2870, new element #2=w2867, index #2=w2868, new element #3=u16 2 ("new element/subarray"), index #3=w2854) -> (w2865:u16[])
            }
            frame "SelectWrong" {
              n1193 = call "myRIO_BRig_RT__Case_Exp_State_Wrong.vi"("input_state"=w2884, "input_dataCurrent"=w2893) -> ("output_state"=w2881:T2, "output_dataCurrent"=w2892:u16[])  [unwired: 8 in]
              n1194 = Not Equal?(x=w2884, y=w2881) -> (x != y?=w2883:bool)
              n1195 = Select(t=myRIO_BRig_RT__Case_Exp_stateList."SelectWrong_post" ("Enum"), s=w2883, f=w2881) -> (s? t:f=w2880:T2)
            }
            frame "SelectWrong_post" {
            }
            frame "SelectTimeout_pre" {
              # "iState"
              # "Tcycle"
              # "counter"
              n1196 = xnode "Read/Write Control"("FPGA VI Reference In"=w2920, "error in"=w2919, "SelectionState"=FALSE) -> ("error out"=→"error out 3":errorcluster)  [unwired: 1 out]
              n1197 = call "myRIO_BRig_RT_dataCurrent_Tcycle_generic.vi"() -> ("output_Tcycle_generic"=w2942:i32)  [unwired: 11 in]
              n1198 = call "myRIO_BRig_RT_dataCurrent_count_generic.vi"() -> ("output_count_generic"=w2940:i32)  [unwired: 11 in]
              n1199 = call "myRIO_BRig_RT_dataExp_Tcycle_Timeout.vi"() -> ("output_Tcycle_Timeout"=w2944:i32)  [unwired: 11 in]
              n1200 = call "myRIO_BRig_RT__Case_Exp_subState_LC__Timeout.vi"("input_spout"=w2935, "input_dataCurrent"=w2936, "input_dataLC"=w2934) -> ()  [unwired: 6 in, 2 out]
              n1201 = Index Array(array=w2938, index=w2944) -> (element=w2943:u16)
              n1202 = call "myRIO_BRig_RT_dataCurrent_iState.vi"() -> ("output_iState"=w2928:i32)  [unwired: 11 in]
              n1203 = Replace Array Subset(array=w2936, new element #1=u16 0 ("new element/subarray"), index #1=w2940, new element #2=w2943, index #2=w2942, new element #3=u16 3 ("new element/subarray"), index #3=w2928) -> (w2939:u16[])
            }
            frame "SelectTimeout" {
              n1204 = call "myRIO_BRig_RT__Case_Exp_State_Timeout.vi"("input_dataLC"=w2963, "input_state"=w2954, "input_dataCurrent"=w2968) -> ("output_state"=w2955:T2, "output_dataCurrent"=w2967:u16[])  [unwired: 6 in, 1 out]
              n1205 = Not Equal?(x=w2954, y=w2955) -> (x != y?=w2958:bool)
              n1206 = Select(t=myRIO_BRig_RT__Case_Exp_stateList."SelectTimeout_post" ("Enum"), s=w2958, f=w2955) -> (s? t:f=w2956:T2)
            }
            frame "SelectTimeout_post" {
            }
            frame "endTrial1" {
              # "Update dataBlock"
              n1207 = call "myRIO_BRig_RT__Case_Exp_State_endTrial1.vi"("input_spout"=w3001, "input_dataBlock"=w3000, "input_dataCurrent"=w2998) -> ("output_dataBlock"=w2999:u16[][], "output_dataCurrent"=w2997:u16[])  [unwired: 7 in]
            }
            frame "endTrial2" {
              # "update dataTrial"
              n1208 = call "myRIO_BRig_RT__Case_Exp_State_endTrial2.vi"("input_spout"=w3020, "input_dataTrial"=w3024, "input_dataCurrent"=w3022) -> ("output_dataTrial"=w3023:u16[][], "output_dataCurrent"=w3021:u16[])  [unwired: 7 in]
            }
            frame "endTrial3" {
              # "nRewTrials"
              # "iTrial"
              # "I_blockUntilReward"
              # "TPB"
              # "end block?"
              n1209 = local read "STOP_endTrial"() -> (w3050:bool)
              n1210 = local read "STOP_abort"() -> (w3049:bool)
              n1211 = xnode "Read/Write Control"("FPGA VI Reference In"=w3040, "error in"=w3039, "SelectionState"=FALSE) -> ("error out"=→"error out 2":errorcluster)  [unwired: 1 out]
              n1212 = local read "START"() -> (w3047:bool)
              n1213 = call "myRIO_BRig_RT_dataExp_IblockUntilReward.vi"() -> ("output_I_blockUntilReward"=w3057:i32)  [unwired: 11 in]
              n1214 = Index Array(array=w3043, index=w3057) -> (element=w3041:u16)
              n1215 = Not(x=w3047) -> (.not. x?=w3048:bool)
              n1216 = Not Equal To 0?(x=w3041) -> (x != 0?=w3055:bool)
              n1217 = Compound Arithmetic op=OR(w3050, w3048, w3049) -> (w3035:bool)
              n1218 = call "myRIO_BRig_RT_dataCurrent_nRewTrials.vi"() -> ("output_nRewTrials"=w3053:i32)  [unwired: 11 in]
              n1219 = call "myRIO_BRig_RT_dataCurrent_iTrial.vi"() -> ("output_iTrial"=w3054:i32)  [unwired: 11 in]
              n1220 = Select(t=w3053, s=w3055, f=w3054) -> (s? t:f=w3052:i32)
              n1221 = call "myRIO_BRig_RT_dataCurrent_TpB.vi"() -> ("output_TpB"=w3056:i32)  [unwired: 11 in]
              n1222 = Index Array(array=w3044, index #1=w3056, index #2=w3052) -> (element #1=w3045:u16, element #2=w3046:u16)
              n1223 = Less Or Equal?(x=w3045, y=w3046) -> (x <= y?=w3036:bool)
              n1224 = Or(x=w3035, y=w3036) -> (x .or. y?=w3033:bool)
              n1225 = Select(t=myRIO_BRig_RT__Case_Exp_stateList."saveData_dataBlock" ("Enum"), s=w3033, f=myRIO_BRig_RT__Case_Exp_stateList."dummyState" ("Enum")) -> (s? t:f=w3042:T2)
            }
            frame "endBlock" {
              # "R"
              # "L"
              # "idxDataBlock"
              n1226 = Equal?(x=w3081, y=enum16{"Left", "Right"}."Left") -> (x = y?=w3080:bool)
              n1227 = call "myRIO_BRig_RT_dataCurrent_idxDataBlockL.vi"() -> ("output_idxDataBlock__L"=w3084:i32)  [unwired: 11 in]
              n1228 = call "myRIO_BRig_RT_dataCurrent_idxDataBlockR.vi"() -> ("output_idxDataBlock__R"=w3083:i32)  [unwired: 11 in]
              n1229 = Increment(x=w3075) -> (x+1=w3074:i32)
              n1230 = local read "START"() -> (w3104:bool)
              n1231 = local read "STOP_endBlock"() -> (w3099:bool)
              n1232 = local read "STOP_endTrial"() -> (w3102:bool)
              n1233 = local read "STOP_abort"() -> (w3101:bool)
              n1234 = Select(t=w3084, s=w3080, f=w3083) -> (s? t:f=w3078:i32)
              n1235 = To Unsigned Word Integer(number=w3074) -> (unsigned 16bit integer=w3076:u16)
              n1236 = Not(x=w3104) -> (.not. x?=w3103:bool)
              n1237 = Replace Array Subset(array=w3079, new element=w3076, index=w3078) -> (w3077:u16[])
              n1238 = Compound Arithmetic op=OR(w3103, w3099, w3102, w3101) -> (w3100:bool)
              n1239 = Select(t=myRIO_BRig_RT__Case_Exp_stateList."endExp" ("Enum"), s=w3100, f=myRIO_BRig_RT__Case_Exp_stateList."dummyState_endBlock" ("Enum")) -> (s? t:f=w3108:T2)
            }
            frame "endExp" {
            }
            frame "commConnect" {
              n1240 = call "myRIO_BRig_RT_comm_webdav_connect.vi"("input_password"="Host Password", "input_username"="Host UserName") -> ("output_Iconnected"=w3129:bool, "output_hSession"=w3147:T6)  [unwired: 7 in, 1 out]
              "Connected To Host?" <- w3129
              n1241 = case shown="False" w3129 {
                frame False {
                  n1242 = One Button Dialog(message="Connection Failed!\nData not being saved!") -> ()  [unwired: 1 in, 1 out]
                }
                frame True {
                }
              }
            }
            frame "commUpload_pre" {
              n1243 = Select(t=myRIO_BRig_RT__Case_Exp_stateList."commUpload_dataBlock" ("Enum"), s=w3154, f=myRIO_BRig_RT__Case_Exp_stateList."endBlock") -> (s? t:f=w3152:T2)
            }
            frame "commUpload_dataBlock" {
              n1244 = call "myRIO_BRig_RT_comm_webdav_uploadFile__data.vi"("input_fileName_prefix"=w3175, "input_fileName"="dataBlock" ("input_filename"), "input_hSession"=w3177) -> ()  [unwired: 8 in, 1 out]
            }
            frame "commUpload_dataCurrent" {
              n1245 = call "myRIO_BRig_RT_comm_webdav_uploadFile__data.vi"("input_fileName_prefix"=w3196, "input_fileName"="dataCurrent" ("input_filename"), "input_hSession"=w3198) -> ()  [unwired: 8 in, 1 out]
            }
            frame "commUpload_dataExp" {
              n1246 = call "myRIO_BRig_RT_comm_webdav_uploadFile__data.vi"("input_fileName_prefix"=w3217, "input_fileName"="dataExp" ("input_filename"), "input_hSession"=w3219) -> ()  [unwired: 8 in, 1 out]
            }
            frame "commUpload_dataLC" {
              n1247 = call "myRIO_BRig_RT_comm_webdav_uploadFile__data.vi"("input_fileName_prefix"=w3238, "input_fileName"="dataLC" ("input_filename"), "input_hSession"=w3240) -> ()  [unwired: 8 in, 1 out]
            }
            frame "commUpload_dataTrial" {
              n1248 = call "myRIO_BRig_RT_comm_webdav_uploadFile__data.vi"("input_fileName_prefix"=w3262, "input_fileName"="dataTrial" ("input_filename"), "input_hSession"=w3264) -> ()  [unwired: 8 in, 1 out]
            }
            frame "saveData_dataBlock" {
              # "idxDataBlockR"
              # "idxDataBlockL"
              n1249 = call "myRIO_BRig_RT_dataCurrent_idxDataBlockL.vi"() -> ("output_idxDataBlock__L"=w3288:i32)  [unwired: 11 in]
              n1250 = call "myRIO_BRig_RT_dataCurrent_idxDataBlockR.vi"() -> ("output_idxDataBlock__R"=w3289:i32)  [unwired: 11 in]
              n1251 = Index Array(array=w3290, index #1=w3288, index #2=w3289) -> (element #1=w3287:u16, element #2=w3286:u16)
              n1252 = Greater?(x=w3287, y=w3286) -> (0:w3285:bool)
              n1253 = Select(t=w3287, s=w3285, f=w3286) -> (s? t:f=w3283:u16)
              n1254 = Increment(x=w3283) -> (x+1=w3282:u16)
              n1255 = To Long Integer(number=w3282) -> (32bit integer=w3281:i32)
              n1256 = Array Subset(array=w3284, length (row)=w3281) -> (w3280:u16[][])  [unwired: 3 in]
              n1257 = call "myRIO_BRig_RT_comm_webdav_saveArrayToFile__2D_u16.vi"("Array"=w3280, "input_filename"="dataBlock") -> ()  [unwired: 10 in]
            }
            frame "saveData_dataCurrent" {
              n1258 = call "myRIO_BRig_RT_comm_webdav_saveArrayToFile__1D_u16.vi"("Array"=w3309, "input_filename"="dataCurrent") -> ()  [unwired: 10 in]
            }
            frame "saveData_dataExp" {
              # "runTime"
              n1259 = Get Date/Time In Seconds() -> (seconds since 1Jan1904=w3337:timestamp)
              n1260 = To Double Precision Float(number=w3337) -> (double precision float=w3336:dbl)
              n1261 = call "myRIO_BRig_RT_dataExp_runTime_seconds.vi"() -> ("output_RunTime_minutes"=w3335:i32)  [unwired: 11 in]
              n1262 = Subtract(x=w3336, y=w3334) -> (x-y=w3331:dbl)
              n1263 = To Unsigned Word Integer(number=w3331) -> (unsigned 16bit integer=w3330:u16)
              n1264 = Replace Array Subset(array=w3329, new element=w3330, index=w3335) -> (w3332:u16[])
              n1265 = call "myRIO_BRig_RT_comm_webdav_saveArrayToFile__1D_u16.vi"("Array"=w3332, "input_filename"="dataExp") -> ()  [unwired: 10 in]
            }
            frame "saveData_dataLC" {
              n1266 = call "myRIO_BRig_RT_comm_webdav_saveArrayToFile__1D_u16.vi"("Array"=w3356, "input_filename"="dataLC") -> ()  [unwired: 10 in]
            }
            frame "saveData_dataTrial" {
              # "idxTrial"
              n1267 = call "myRIO_BRig_RT_dataCurrent_idxDataTrial.vi"() -> ("output_idxDataTrial"=w3380:i32)  [unwired: 11 in]
              n1268 = Index Array(array=w3381, index=w3380) -> (element=w3373:u16)
              n1269 = Increment(x=w3373) -> ()  [unwired: 1 out]
              n1270 = To Long Integer(number=w3373) -> (32bit integer=w3377:i32)
              n1271 = Array Subset(array=w3378, length (row)=w3377) -> (w3379:u16[][])  [unwired: 3 in]
              n1272 = call "myRIO_BRig_RT_comm_webdav_saveArrayToFile__2D_u16.vi"("Array"=w3379, "input_filename"="dataTrial") -> ()  [unwired: 10 in]
            }
            frame "dummyState" {
              n1273 = call "myRIO_BRig_RT_dataCurrent_iTrial.vi"() -> ("output_iTrial"=w3403:i32)  [unwired: 11 in]
              n1274 = Index Array(array=w3404, index=w3403) -> (element=w3402:u16)
              n1275 = Equal?(x=w3402, y=u16 1) -> (x = y?=w3400:bool)
              n1276 = Equal To 0?(x=w3411) -> (x = 0?=w3412:bool)
              n1277 = Select(t=u16 13, s=w3400, f=u16 15) -> (s? t:f=w3397:u16)
              n1278 = Select(t=w3397, s=w3412, f=w3411) -> (s? t:f=w3410:u16)
              n1279 = Decrement(x=w3410) -> (x-1=w3409:u16)
              n1280 = Equal To 0?(x=w3409) -> (x = 0?=w3408:bool)
              n1281 = Select(t=myRIO_BRig_RT__Case_Exp_stateList."initTrial" ("Enum"), s=w3408, f=w3406) -> (s? t:f=w3405:T2)
            }
            frame "dummyState_endBlock" {
              n1282 = call "myRIO_BRig_RT_dataCurrent_iTrial.vi"() -> ("output_iTrial"=w3436:i32)  [unwired: 11 in]
              n1283 = Index Array(array=w3437, index=w3436) -> (element=w3435:u16)
              n1284 = Equal?(x=w3435, y=u16 1) -> (x = y?=w3433:bool)
              n1285 = Equal To 0?(x=w3444) -> (x = 0?=w3445:bool)
              n1286 = Select(t=u16 1, s=w3433, f=u16 3) -> (s? t:f=w3430:u16)
              n1287 = Select(t=w3430, s=w3445, f=w3444) -> (s? t:f=w3443:u16)
              n1288 = Decrement(x=w3443) -> (x-1=w3442:u16)
              n1289 = Equal To 0?(x=w3442) -> (x = 0?=w3441:bool)
              n1290 = Select(t=myRIO_BRig_RT__Case_Exp_stateList."initBlock" ("Enum"), s=w3441, f=w3439) -> (s? t:f=w3438:T2)
            }
          }
          n1291 = Select(t=w1084, s=w1087, f=w1085) -> (s? t:f=w1086:bool)
          n1292 = Or(x=w1046, y=w1047) -> (x .or. y?=w1045:bool)
          n1293 = Or(x=w1126, y=w1125) -> (x .or. y?=w1044:bool)
          n1294 = case shown="True" w1154 {
            tunnel: w1151 -> [w1175 w1183]
            tunnel: w1153 -> [_ w1179]
            tunnel: w1152 -> [_ w1178]
            tunnel: w1058 -> [_ w1177]
            tunnel: w1123 -> [_ w1176]
            tunnel: [w1175 w1182] -> w1150
            tunnel: w1149 -> [w1174 w1181]
            tunnel: [w1174 w1180] -> w1148
            frame False {
            }
            frame True {
              n1295 = call "myRIO_BRig_RT__Case_Exp__recordLick.vi"("intput_state__trialEnd"=w1176, "intput_state__trialStart"=w1177, "input_lick__R"=w1178, "input_lick__L"=w1179, "input_dataCurrent"=w1181, "input_dataLick"=w1183) -> ("output_dataCurrent"=w1180:u16[], "output_dataLick"=w1182:u16[][])  [unwired: 4 in]
            }
          }
          n1296 = Or(x=w1127, y=w1111) -> (x .or. y?=w1100:bool)
          n1297 = Or(x=w1110, y=w1128) -> (x .or. y?=w1124:bool)
          n1298 = Or(x=w1155, y="STOP_abort") -> (x .or. y?=w1157:bool)
          n1299 = Or(x=w1090, y=w1091) -> (x .or. y?=w1088:bool)
          n1300 = Or(x=w1092, y=w1091) -> (x .or. y?=w1089:bool)
          n1301 = Select(t=w1073, s=w1074, f=w1072) -> (s? t:f=w1057:u16)
          n1302 = Select(t=w1075, s=w1077, f=w1076) -> (s? t:f=w1056:u16)
          n1303 = Select(t=u16 0, s=w1080, f=w1079) -> (s? t:f=w1064:u16)
          n1304 = xnode "Read/Write Control"("FPGA VI Reference In"=w1102, "error in"=w1101, "A3_SL"=w1045, "A1_SR"=w1044, "A6_Act"=w1086, "audioTrigger_L"=w1100, "audioAmp_L"=w1137, "audioFreq_L_kHz"=w1109, "audioTrigger_R"=w1124, "audioAmp_R"=w1138, "audioFreq_R_kHz"=w1139, "LC_Event_l1"=w1088, "LC_Laser_l1"=w1089, "LC_Event_l2"=w1043, "LC_Laser_l2"=w1042, "CueLed_Event"=w1041) -> ("FPGA VI Reference Out"=w1147:refnum<k20>, "error out"=w1146:errorcluster, "AnaIn_0"=w1050:i16, "AnaIn_1"=w1063:i16)
          n1305 = call "myRIO_BRig_RT_dataAnalog_enterData__PortC.vi"("input_iState"=w1058, "input_AI0"=w1050, "input_iEvent"=w1064, "input_AI1"=w1063, "input_iTrial"=w1057, "input_iBlock"=w1056, "input_index"=w1065, "input_dataAnalog"=w1083) -> ("output_dataAnalog"=w1082:u16[][])  [unwired: 3 in]
          n1306 = call "myRIO_BRig_RT_TCP__v3__PortC.vi"("input_hTCP"=w1070, "input_AI1"=w1063, "input_AI0"=w1050, "input_I_connected_TCP"=w1066, "input_iBlock"=w1056, "input_spout"=w1055, "input_iTrial"=w1057, "input_error"=w1068, "input_countTrial"=w1052, "input_iState"=w1058) -> ("output_hTCP"=w1069:refnum<k5>, "output_countTrial"=w1051:u16, "output_error"=w1067:errorcluster)  [unwired: 3 in]
          n1307 = node-c288() -> ()  [unwired: 1 in, 1 out]
          n1308 = Increment(x=w1064) -> (x+1=w1071:u16)
          n1309 = Increment(x=w1065) -> (x+1=w1081:i32)
          "cState" <- w1058
        }
        n1310 = node-c288(w991) -> ()  [unwired: 1 out]
        n1311 = flat-sequence {
          tunnel: w987 -> [w1036]
          tunnel: w986 -> [w1035]
          tunnel: [w1034] -> w979
          tunnel: [w1033] -> w978
          tunnel: [w1039] -> w980
          tunnel: [w1040] -> w985
          tunnel: w979 -> [w1040]
          tunnel: w978 -> [w1039]
          frame #0 {
            w1030 = u8 0
            w1031 = u16 0 ("AudioLeft_phase_inc")
            w1032 = FALSE
            n1312 = xnode "Read/Write Control"("FPGA VI Reference In"=w1036, "error in"=w1035, "Counts_Reset"=TRUE, "audioTrigger_L"=w1032, "audioFreq_L_kHz"=w1030, "audioAmp_L"=w1031, "audioTrigger_R"=w1032, "audioFreq_R_kHz"=w1030, "audioAmp_R"=w1031, "A3_SL"=w1032, "A1_SR"=w1032, "A6_Act"=w1032) -> ("FPGA VI Reference Out"=w1034:refnum<k20>, "error out"=w1033:errorcluster)
          }
          frame #1 {
            w1038 = FALSE ("START")
            n1313 = local write "START"(w1038) -> ()
            n1314 = local write "STOP_endTrial"(w1038) -> ()
            n1315 = local write "STOP_endBlock"(w1038) -> ()
          }
        }
        n1316 = stacked-sequence {
          tunnel: w963 -> [w1010 _]
          tunnel: w961 -> [w1011 _]
          tunnel: w960 -> [_ w1016]
          tunnel: w959 -> [_ w1015]
          tunnel: w958 -> [_ w1014]
          tunnel: w957 -> [w1004 _]
          tunnel: w937 -> [w1001 _]
          tunnel: w936 -> [w1000 _]
          frame #0 {
            n1317 = call "myRIO_BRig_RT_dataCurrent_idxDataLick.vi"() -> ("output_idxDataLick"=w1005:i32)  [unwired: 11 in]
            n1318 = Index Array(array=w1004, index=w1005) -> (element=w1007:u16)
            n1319 = Array Subset(array=w1001, length (row)=w1000) -> (w1002:u16[][])  [unwired: 3 in]
            n1320 = Increment(x=w1007) -> (x+1=w1008:u16)
            n1321 = call "myRIO_BRig_RT_comm_webdav_saveArrayToFile__1D_u16.vi"("Array"=w1011, "input_filename"="dataMTrig") -> ()  [unwired: 10 in]
            n1322 = To Long Integer(number=w1008) -> (32bit integer=w1006:i32)
            n1323 = Array Subset(array=w1010, length (row)=w1006) -> (w1009:u16[][])  [unwired: 3 in]
            n1324 = call "myRIO_BRig_RT_comm_webdav_saveArrayToFile__2D_u16.vi"("Array"=w1009, "input_filename"="dataLick") -> ()  [unwired: 10 in]
            n1325 = call "myRIO_BRig_RT_comm_webdav_saveArrayToFile__2D_u16.vi"("Array"=w1002, "input_filename"="dataAnalog") -> ()  [unwired: 10 in]
          }
          frame #1 {
            n1326 = case shown="True" w1016 {
              tunnel: w1015 -> [_ w1018]
              tunnel: w1014 -> [_ w1017]
              frame False {
              }
              frame True {
                n1327 = stacked-sequence {
                  tunnel: w1018 -> [w1020 w1027 w1029]
                  tunnel: w1017 -> [w1021 w1026 _]
                  frame #0 {
                    n1328 = call "myRIO_BRig_RT_comm_webdav_uploadFile__announce.vi"("input_addText"=TRUE, "input_fileName_prefix"=w1021, "intput_fileName"="curExp_end", "intput_hSession"=w1020) -> ("output_Isuccess"=w1019:bool)  [unwired: 6 in, 1 out]
                    n1329 = case shown="True" w1019 {
                      frame False {
                        n1330 = One Button Dialog(message="!!! Warning !!! Your data is located at C:\\BehaviorRig\\commTransfer") -> ()  [unwired: 1 in, 1 out]
                      }
                      frame True {
                        n1331 = Wait (ms)(milliseconds to wait=u32 20) -> ()  [unwired: 1 out]
                      }
                    }
                  }
                  frame #1 {
                    n1332 = call "myRIO_BRig_RT__endExp_sendData.vi"("input_fileName_prefix"=w1026, "input_hSession"=w1027) -> ()  [unwired: 8 in, 2 out]
                  }
                  frame #2 {
                    n1333 = local write "Connected To Host?"(FALSE ("Connected To Host?")) -> ()
                    n1334 = call <vilib>:"Close Session.vi"("session handle"=w1029) -> ()  [unwired: 14 in, 1 out]
                  }
                }
              }
            }
          }
        }
      }
    }
    n1335 = local read "STOP_abort"() -> (w44:bool)
  }
  n1336 = case shown="True" w5 {
    tunnel: w4 -> [_ w3468]
    tunnel: w3 -> [_ w3467]
    frame False {
    }
    frame True {
      n1337 = call "myRIO__TCP_disconnect_forWrite.vi"("input_error"=w3467, "input_hTCP"=w3468) -> ()  [unwired: 9 in, 1 out]
    }
  }
  n1338 = xnode "Read/Write Control"("FPGA VI Reference In"=w16, "error in"=w15, "FPGA_Stop"=TRUE) -> ("FPGA VI Reference Out"=w21:refnum<k20>, "error out"=w22:errorcluster)
  n1339 = xnode "Close FPGA VI Reference"("FPGA VI Reference In"=w21, "error in"=w22) -> ("error out"=w20:errorcluster)
  n1340 = call <vilib>:"Reset myRIO.vi"("error in (no error)"=w20) -> ()  [unwired: 10 in, 1 out]
